vi "WVDIAL+HSRL_v5.3.vi"() -> ()   [LabVIEW 2012]
uses:
  C:/Users/H2ODial/Desktop/Shared Telescope WV DIAL Code/Libraries and VIs/PowerMeterCommands.dll
  Shared Telescope WV DIAL Code/Libraries and VIs/PowerMeterCommands.dll
  <vilib>/DAQmx/write.llb/DAQmx Write (Digital 1D Bool NChan 1Samp 1Line).vi
  <vilib>/DAQmx/miscellaneous.llb/DAQmx Fill In Error Info.vi
  <vilib>/Analysis/baseanly.llb/Mean (DBL).vi
  NCAR_DIAL_Labview/AMCS_Data.vi
  Shared Telescope WV DIAL Code/Libraries and VIs/Scalar_Data.vi
  <vilib>/Analysis/NI_AALBase.lvlib
  Shared Telescope WV DIAL Code/Libraries and VIs/Scalar_Data_2.vi
  Shared Telescope WV DIAL Code/Libraries and VIs/Scalar_Data_4.vi
  Shared Telescope WV DIAL Code/Libraries and VIs/Scalar_Data_3.vi
  Shared Telescope WV DIAL Code/bristol/CLDevIFace.dll
panel:
  out "sigma_off_total":dbl[](array[numeric])=[4.7361664206831265e-25, 4.704555265189846e-25, 4.67312277669019e-25, 4.641868603215992e-25, 4.610792386086212e-25, 4.5798937599868365e-25, 4.549172353018389e-25, 4.51862778677416e-25, 4.488259676402069e-25, 4.458067630633013e-25, 4.428051251896184e-25, 4.398210136337557e-25, 4.368543873901429e-25, 4.339052048374652e-25, 4.309734237462183e-25, 4.280590012841455e-25, 4.251618940197595e-25, 4.2228205793205105e-25, 4.194194484107976e-25, 4.165740202676913e-25, 4.137457277365156e-25, 4.109345244819803e-25, 4.0814036360397235e-25, 4.0536319764083216e-25, 4.026029785750973e-25, 3.99859657840818e-25, 3.9713318632399474e-25, 3.944235143701286e-25, 3.917305917875353e-25, 3.8905436785136965e-25, 3.8639479130808273e-25, 3.8375181038031018e-25, 3.8112537276873907e-25, 3.785154256573241e-25, 3.759219157169389e-25, 3.7334478910754945e-25, 3.7078399148261516e-25, 3.6823946799305074e-25, 3.6571116328753168e-25, 3.631990215175425e-25, 3.6070298633991576e-25, 3.5822300091890585e-25, 3.5575900792854463e-25, 3.5331094955517765e-25, 3.5087876749908485e-25, 3.4846240297677933e-25, 3.4606179672362523e-25, 3.436768889934375e-25, 3.413076195617018e-25, 3.3895392772615455e-25, 3.3661575230847493e-25, 3.342930316532612e-25, 3.319857036317709e-25, 3.296937056408611e-25, 3.2741697460261917e-25, 3.251554469671832e-25, 3.2290905870931807e-25, 3.2067774533121854e-25, 3.1846144186158143e-25, 3.162600828540832e-25, 3.140736023869109e-25, 3.119019340630677e-25, 3.097450110083946e-25, 3.0760276586997706e-25, 3.0547513081546247e-25, 3.0336203753156617e-25, 3.0126341721968216e-25, 2.991792005980208e-25, 2.971093178956684e-25, 2.9505369885181706e-25, 2.930122727127669e-25, 2.9098496822848683e-25, 2.889717136509742e-25, 2.8697243672739283e-25, 2.8498706470054586e-25, 2.830155243027821e-25, 2.8105774175268934e-25, 2.7911364274987386e-25, 2.7718315247081357e-25, 2.752661955653541e-25, 2.7336269615027698e-25, 2.7147257780457946e-25, 2.6959576356446162e-25, 2.6773217591650263e-25, 2.6588173679341805e-25, 2.6404436756788697e-25, 2.622199890449384e-25, 2.604085214561746e-25, 2.586098844541831e-25, 2.568239971051803e-25, 2.550507778817499e-25, 2.5329014465553983e-25, 2.5154201469120286e-25, 2.4980630463842063e-25, 2.480829305237817e-25, 2.4637180774559744e-25, 2.446728510637542e-25, 2.4298597459368107e-25, 2.413110917982359e-25, 2.3964811547911274e-25, 2.379969577731832e-25, 2.3635753013998594e-25, 2.347297433572206e-25, 2.3311350751401097e-25, 2.31508732002067e-25, 2.2991532551047967e-25, 2.2833319601734517e-25, 2.2676225078671837e-25, 2.252023963583222e-25, 2.236535385474671e-25, 2.221155824352112e-25, 2.2058843236723785e-25, 2.190719919472833e-25, 2.1756616403747133e-25, 2.160708507518757e-25, 2.1458595345686165e-25, 2.1311137277120556e-25, 2.1164700856449227e-25, 2.1019275995907964e-25, 2.087485253289068e-25, 2.073142023094825e-25, 2.0588968779652238e-25, 2.0447487795305943e-25, 2.0306966821944526e-25, 2.016739533161752e-25, 2.0028762726015144e-25, 1.9891058337447025e-25, 1.975427143010045e-25, 1.9618391201384895e-25, 1.948340678436903e-25, 1.9349307248979029e-25, 1.9216081604537808e-25, 1.9083718801827206e-25, 1.895220773627962e-25, 1.8821537249925881e-25, 1.869169613534671e-25, 1.8562673138214617e-25, 1.8434456961361037e-25, 1.8307036268484988e-25, 1.8180399688349342e-25, 1.8054535818752412e-25, 1.7929433231795034e-25, 1.7805080478581835e-25, 1.7681466094122697e-25, 1.755857860345701e-25, 1.7436406526975642e-25, 1.7314938387295936e-25, 1.7194162714756045e-25, 1.7074068054790102e-25, 1.695464297486202e-25, 1.683587607177604e-25, 1.6717755978952424e-25, 1.6600271375100748e-25, 1.6483410991903818e-25, 1.6367163622623877e-25, 1.6251518130749766e-25, 1.6136463459136442e-25, 1.6021988639543779e-25, 1.5908082801260055e-25, 1.5794735181698975e-25, 1.5681935136280992e-25, 1.5569672147704635e-25, 1.5457935837366772e-25, 1.534671597460114e-25, 1.5236002488417742e-25, 1.5125785477293987e-25, 1.5016055220247154e-25, 1.4906802187584044e-25, 1.479801705155579e-25, 1.468969069798589e-25, 1.4581814235650682e-25, 1.4474379007909321e-25, 1.436737660408928e-25, 1.4260798867874899e-25, 1.4154637909757664e-25, 1.4048886116065242e-25, 1.3943536158832026e-25, 1.3838581006765858e-25, 1.3734013932288368e-25, 1.3629828522951373e-25, 1.3526018689008124e-25, 1.342257867119734e-25, 1.3319503049616873e-25, 1.3216786750244633e-25, 1.31144250521248e-25, 1.301241359412424e-25, 1.291074837942134e-25, 1.280942578189995e-25, 1.2708442550183176e-25, 1.2607795810937358e-25, 1.2507483073612695e-25, 1.240750223055036e-25, 1.2307851560870465e-25, 1.2208529730375792e-25, 1.210953579206839e-25, 1.2010869185647356e-25, 1.191252973591614e-25, 1.181451765122348e-25, 1.1716833520039885e-25, 1.1619478307265666e-25, 1.1522453350562395e-25, 1.1425760353747595e-25, 1.1329401381799674e-25, 1.1233378853998675e-25, 1.113769553537836e-25, 1.1042354529141042e-25, 1.0947359268328863e-25, 1.0852713503919777e-25, 1.0758421297055504e-25, 1.0664487005835578e-25, 1.0570915274849075e-25, 1.047771102223147e-25, 1.03848794275529e-25, 1.0292425918306789e-25, 1.0200356155490214e-25, 1.010867602053661e-25, 1.0017391599688187e-25, 9.926509169958122e-26, 9.836035183502962e-26, 9.745976252120823e-26, 9.65633913229687e-26, 9.567130708754601e-26, 9.478357978493009e-26, 9.390028035717989e-26, 9.302148055431555e-26, 9.214725277448196e-26, 9.127766990988825e-26, 9.041280518865252e-26, 8.955273202137755e-26, 8.869752384860457e-26, 8.784725399226806e-26, 8.700199550942864e-26, 8.616182105040356e-26, 8.532680271869519e-26, 8.449701193777957e-26, 8.367251931994412e-26, 8.285339454310501e-26, 8.203970622936562e-26, 8.123152183149593e-26, 8.042890752341435e-26, 7.963192809815122e-26, 7.884064686929539e-26, 7.805512558301465e-26, 7.727542432949971e-26, 7.650160146934502e-26, 7.57337135604093e-26, 7.497181529080177e-26, 7.421595942284274e-26, 7.346619674445024e-26, 7.272257601587051e-26, 7.198514394124386e-26, 7.125394512886316e-26, 7.052902207211764e-26, 6.981041512330182e-26, 6.909816249334807e-26, 6.839230023128457e-26, 6.769286223445015e-26, 6.699988025335878e-26, 6.631338390073311e-26, 6.563340066584491e-26, 6.49599559494312e-26, 6.42930730805647e-26, 6.363277335648878e-26, 6.297907608168418e-26, 6.233199860791015e-26, 6.169155638647973e-26, 6.105776301230497e-26, 6.043063030280447e-26, 5.981016833347322e-26, 5.919638551567296e-26, 5.858928867629214e-26, 5.798888310028938e-26, 5.739517264230729e-26, 5.680815977446289e-26, 5.622784570821595e-26, 5.565423042824561e-26, 5.508731282073838e-26, 5.452709076027738e-26, 5.397356119112836e-26, 5.342672021546054e-26, 5.288656322652946e-26, 5.235308497562398e-26, 5.182627968877097e-26, 5.1306141180432717e-26, 5.079266295448115e-26, 5.0285838305725196e-26, 4.9785660439920176e-26, 4.9292122597178655e-26, 4.880521816085966e-26, 4.832494077663027e-26, 4.785128445476612e-26, 4.738424375125138e-26, 4.6923813828266026e-26, 4.6469990631962226e-26, 4.602277098489981e-26, 4.558215278470542e-26, 4.5148135069875e-26, 4.472071819308421e-26, 4.4299904003223627e-26, 4.3885695940220764e-26, 4.34780992252792e-26, 4.3077121010301005e-26, 4.2682770570367184e-26, 4.229505941304242e-26, 4.191400156132326e-26, 4.153961360924621e-26, 4.1171915050160506e-26, 4.081092840060667e-26, 4.045667941127819e-26, 4.0109197318421695e-26, 3.976851511059284e-26, 3.94346696850793e-26, 3.910770219989253e-26, 3.878765828740234e-26, 3.847458837721502e-26, 3.8168548023517886e-26, 3.786959816579413e-26, 3.7577805545800425e-26, 3.729324308299501e-26, 3.7015990199603826e-26, 3.674613333708746e-26, 3.648376631776354e-26, 3.622899094820171e-26, 3.598191740617036e-26, 3.574266496427956e-26, 3.5511362455100554e-26, 3.528814896198588e-26, 3.507317461176492e-26, 3.486660118207953e-26, 3.466860307888483e-26, 3.4479368137858184e-26, 3.4299098560632234e-26, 3.412801205464934e-26, 3.3966342919810845e-26, 3.3814343251481105e-26, 3.367228427279176e-26, 3.354045786622697e-26, 3.3419178044404247e-26, 3.3308782806715067e-26, 3.3209635809193336e-26, 3.312212860029802e-26, 3.3046682753827244e-26, 3.2983752185562495e-26, 3.29338260025694e-26, 3.2897431142923784e-26, 3.287513568833748e-26, 3.2867552048982673e-26, 3.2875340853067966e-26, 3.289921476512414e-26, 3.2939942920704573e-26, 3.299835560859249e-26, 3.3075349233297295e-26, 3.31718918068937e-26, 3.3289028648791126e-26, 3.342788865753138e-26, 3.358969065149828e-26, 3.377575025168756e-26, 3.398748657265788e-26, 3.422642954607728e-26, 3.449422652081664e-26, 3.4792648667855453e-26, 3.512359674236963e-26, 3.5489105220039706e-26, 3.5891344431644435e-26, 3.633261965097536e-26, 3.6815365592521375e-26, 3.734213474993317e-26, 3.791557697858917e-26, 3.8538406892390413e-26, 3.9213356153192504e-26, 3.9943102879548856e-26, 4.073017384110245e-26, 4.1576808542827767e-26, 4.248477496232471e-26, 4.345512364768352e-26, 4.448786294634738e-26, 4.5581537709586704e-26, 4.6732692284515773e-26, 4.793519837808654e-26, 4.9179435948328834e-26, 5.0451328371338053e-26, 5.1731255142748e-26, 5.299290837924887e-26, 5.420222023626943e-26, 5.53165663953385e-26, 5.628454891291683e-26, 5.704674823501702e-26, 5.753787062260405e-26, 5.769064643115553e-26, 5.74415889460443e-26, 5.673827133946316e-26, 5.554718344465795e-26, 5.386066929337925e-26, 5.170120323121083e-26, 4.912158035835312e-26, 4.6200514475002547e-26, 4.3034358779098605e-26, 3.9726716277435353e-26, 3.6378128374023453e-26, 3.307772708312355e-26, 2.989791844851222e-26, 2.6892241436515096e-26, 2.409585649271807e-26, 2.1527785770835842e-26, 1.919402511159775e-26, 1.709083279709411e-26, 1.5207745119483158e-26, 1.3530095944864033e-26, 1.2040974338307356e-26, 1.0722654911053451e-26, 9.55758170763187e-27, 8.529000269297322e-27, 7.621326815896537e-27, 6.820331294600264e-27, 6.113193384990869e-27, 5.4884768053552995e-27, 4.936054405988233e-27, 4.447006306596712e-27, 4.01350649482812e-27, 3.6287074114691265e-27, 3.286628665045252e-27, 2.982053133857502e-27, 2.710432190494805e-27, 2.467800620632622e-27, 2.2507010863407657e-27, 2.0561176436578528e-27, 1.8814175678696082e-27, 1.724300676600419e-27, 1.5827553313450851e-27, 1.4550203259299805e-27, 1.3395518832270707e-27, 1.234995172388499e-27, 1.1401596616151055e-27, 1.0539978395563054e-27, 9.755868171920564e-28, 9.041124308282113e-28, 8.388554686323786e-28, 7.791797569678583e-28, 7.245218245948973e-28, 6.743819381596948e-28, 6.283163098755046e-28, 5.8593032346752675e-28, 5.468726321210164e-28, 5.108300131750884e-28, 4.775228773786931e-28, 4.467013412002027e-28, 4.181417907319234e-28, 3.916438696977483e-28, 3.670278362224614e-28, 3.4413224156682114e-28, 3.2281188706205514e-28, 3.029360261582784e-28, 2.8438677764436214e-28, 2.6705772634396255e-28, 2.5085268535677297e-28, 2.356846015299008e-28, 2.2147458604462534e-28, 2.081510545634908e-28, 1.9564896453728212e-28, 1.8390913738842352e-28, 1.7287765586913761e-28, 1.6250532759661657e-28, 1.5274720714661247e-28, 1.435621701168333e-28, 1.3491253280333026e-28, 1.2676371266924668e-28, 1.1908392491273447e-28, 1.1184391104493528e-28, 1.0501669588488019e-28, 9.857737007616221e-29, 9.250289505277767e-29, 8.677192817164208e-29, 8.136466585155294e-29, 7.626270269664177e-29, 7.144890498931933e-29, 6.690729697909333e-29, 6.262295865445962e-29, 5.858193379226559e-29, 5.477114719070298e-29, 5.117833016685385e-29, 4.779195345355935e-29, 4.460116672941723e-29, 4.159574412717862e-29, 3.8766035085313356e-29, 3.610292001520259e-29, 3.359777029252782e-29, 3.1242412137098097e-29, 2.902909398873338e-29, 2.695045702172569e-29, 2.499950848733905e-29, 2.3169597597114745e-29, 2.1454393688082381e-29, 1.984786644280984e-29, 1.8344267951922419e-29, 1.6938116433705343e-29, 1.5624181441700836e-29, 1.439747040443755e-29, 1.3253216363128416e-29, 1.2186866778564523e-29, 1.1194073298259488e-29, 1.027068237868702e-29, 9.41272667323786e-30, 8.616417100740263e-30, 7.878135520832268e-30, 7.194427947435567e-30, 6.561998239457055e-30, 5.9777022134514484e-30, 5.438542128318805e-30, 4.941661497222303e-30, 4.4843401864961795e-30, 4.0639897652743174e-30, 3.678149073494049e-30, 3.32447997937297e-30, 3.000763300568808e-30, 2.7048948662138683e-30, 2.4348816997231054e-30, 2.1888383046853783e-30, 1.9649830384363482e-30, 1.7616345601080574e-30, 1.5772083417641433e-30, 1.41021323314241e-30, 1.2592480721156737e-30, 1.1229983345711438e-30, 1.0002328188090904e-30, 8.898003608818597e-31, 7.906265785078758e-31, 7.017106423265677e-31, 6.221220742613051e-31, 5.509975737248236e-31, 4.875378732287941e-31, 4.3100462574946304e-31, 3.8071732687790596e-31, 3.3605027540420555e-31, 2.964295765136466e-31, 2.6133019224912582e-31, 2.302730443047367e-31, 2.028221746319981e-31, 1.785819698883956e-31, 1.571944569933226e-31, 1.383366812786611e-31, 1.217181992487339e-31, 1.0707887255920024e-31, 9.41901183885076e-32, 8.286711261751362e-32, 7.282214916074516e-32, 6.400758489832818e-32, 5.623904147671109e-32, 4.938867921697972e-32, 4.334463318815432e-32, 3.80089121769985e-32, 3.329583042957907e-32, 2.9130592710425146e-32, 2.544799971983946e-32, 2.219126721730452e-32, 1.9310955232755848e-32]
  out "sigma_on_total":dbl[](array[numeric])=[1.4787315438349907e-23, 1.471501798802285e-23, 1.464231394662418e-23, 1.4569216526022592e-23, 1.4495738897409737e-23, 1.4421894186265373e-23, 1.434769546715974e-23, 1.4273155759788748e-23, 1.4198288023456042e-23, 1.4123105152791947e-23, 1.4047619973042604e-23, 1.3971845236586865e-23, 1.3895793617371425e-23, 1.381947770795712e-23, 1.3742910015857432e-23, 1.3666102958094782e-23, 1.3589068859169402e-23, 1.3511819946965545e-23, 1.343436834852627e-23, 1.3356726088660775e-23, 1.3278905084359422e-23, 1.3200917143654812e-23, 1.3122773962181173e-23, 1.3044487120136741e-23, 1.2966068079379167e-23, 1.2887528181705935e-23, 1.280887864645543e-23, 1.2730130566668176e-23, 1.2651294909304667e-23, 1.2572382511131376e-23, 1.2493404078126522e-23, 1.2414370183434812e-23, 1.2335291264934119e-23, 1.2256177624718979e-23, 1.217703942715269e-23, 1.2097886697548654e-23, 1.2018729320712635e-23, 1.1939577040847508e-23, 1.1860439459053391e-23, 1.178132603369378e-23, 1.1702246078860594e-23, 1.1623208764429943e-23, 1.1544223114245504e-23, 1.1465298007100527e-23, 1.1386442174876053e-23, 1.1307664203452922e-23, 1.1228972532006195e-23, 1.1150375452637873e-23, 1.1071881110338761e-23, 1.0993497503734642e-23, 1.0915232484490551e-23, 1.0837093757279006e-23, 1.075908888098364e-23, 1.0681225268339973e-23, 1.0603510186352726e-23, 1.0525950757460925e-23, 1.0448553958493267e-23, 1.037132662354594e-23, 1.0294275442393744e-23, 1.0217406963238484e-23, 1.0140727591488213e-23, 1.0064243592154774e-23, 9.987961090294116e-24, 9.911886071512357e-24, 9.836024383391568e-24, 9.760381736518965e-24, 9.684963704924737e-24, 9.60977572847412e-24, 9.534823112538791e-24, 9.460111030247358e-24, 9.385644523289062e-24, 9.311428503379682e-24, 9.237467752939021e-24, 9.1637669272307e-24, 9.09033055529708e-24, 9.017163041332023e-24, 8.944268665880828e-24, 8.871651587851976e-24, 8.799315845358803e-24, 8.727265357183314e-24, 8.65550392483017e-24, 8.584035233431315e-24, 8.512862853443734e-24, 8.441990241976577e-24, 8.371420744879967e-24, 8.30115759752875e-24, 8.231203926927024e-24, 8.161562752887824e-24, 8.092236989774732e-24, 8.023229448060604e-24, 7.954542835889658e-24, 7.886179760290278e-24, 7.818142729624757e-24, 7.750434154096213e-24, 7.683056347675882e-24, 7.616011530181347e-24, 7.549301828314853e-24, 7.482929277057427e-24, 7.416895821895255e-24, 7.351203319362845e-24, 7.285853539749422e-24, 7.220848167799621e-24, 7.156188804409643e-24, 7.091876968465427e-24, 7.02791409755192e-24, 6.964301550724863e-24, 6.901040608572782e-24, 6.838132475952623e-24, 6.775578282364756e-24, 6.713379084183873e-24, 6.651535865939141e-24, 6.590049541293287e-24, 6.5289209550606835e-24, 6.46815088430602e-24, 6.40774003944497e-24, 6.347689066346921e-24, 6.2879985469666566e-24, 6.228669001264069e-24, 6.169700887964062e-24, 6.111094606297088e-24, 6.0528504971542e-24, 5.994968844369398e-24, 5.937449875851488e-24, 5.880293765105849e-24, 5.82350063219817e-24, 5.767070545238083e-24, 5.7110035214439225e-24, 5.655299527942129e-24, 5.5999584837121235e-24, 5.544980260090087e-24, 5.490364682162052e-24, 5.436111530002443e-24, 5.3822205392790905e-24, 5.328691403076694e-24, 5.275523772106918e-24, 5.2227172566077816e-24, 5.170271426653518e-24, 5.118185813533807e-24, 5.066459910980123e-24, 5.015093175565678e-24, 4.964085027910957e-24, 4.9134348538588365e-24, 4.863142005178444e-24, 4.813205800593375e-24, 4.7636255264628436e-24, 4.714400437887786e-24, 4.665529759575633e-24, 4.617012686584397e-24, 4.568848385057435e-24, 4.521035993359352e-24, 4.473574622567741e-24, 4.4264633574709985e-24, 4.379701257140268e-24, 4.333287356089523e-24, 4.2872206644216265e-24, 4.241500168960551e-24, 4.196124833867207e-24, 4.151093601530227e-24, 4.106405392776687e-24, 4.06205910811475e-24, 4.01805362783006e-24, 3.9743878130977926e-24, 3.931060506426416e-24, 3.888070532187342e-24, 3.845416697225424e-24, 3.803097791801521e-24, 3.761112589558677e-24, 3.719459848784516e-24, 3.6781383122768084e-24, 3.6371467083176915e-24, 3.596483751198191e-24, 3.556148141569368e-24, 3.5161385668725815e-24, 3.476453702237941e-24, 3.437092210484289e-24, 3.398052742913235e-24, 3.359333939535743e-24, 3.3209344298325475e-24, 3.282852832810783e-24, 3.2450877578143793e-24, 3.20763780456859e-24, 3.1705015639611164e-24, 3.1336776181464896e-24, 3.097164541012893e-24, 3.0609608986345336e-24, 3.0250652497092765e-24, 2.9894761456426302e-24, 2.9541921311120647e-24, 2.9192117444089036e-24, 2.8845335177057522e-24, 2.8501559773849925e-24, 2.8160776443587784e-24, 2.7822970344442195e-24, 2.7488126586004656e-24, 2.7156230232245448e-24, 2.6827266305003526e-24, 2.6501219784943642e-24, 2.6178075617335478e-24, 2.5857818711071018e-24, 2.554043394426032e-24, 2.5225906166099657e-24, 2.4914220197581437e-24, 2.460536083562059e-24, 2.4299312854227364e-24, 2.3996061007879786e-24, 2.3695590033135076e-24, 2.3397884650752963e-24, 2.3102929567234233e-24, 2.2810709477376482e-24, 2.2521209066220334e-24, 2.223441301144551e-24, 2.195030598367685e-24, 2.1668872649808488e-24, 2.139009767421492e-24, 2.1113965718990352e-24, 2.0840461448985418e-24, 2.0569569529523272e-24, 2.0301274631283374e-24, 2.0035561428054193e-24, 1.9772414602815678e-24, 1.9511818844995554e-24, 1.9253758853690898e-24, 1.899821933940881e-24, 1.8745185024029975e-24, 1.849464064377468e-24, 1.824657094743691e-24, 1.8000960701355398e-24, 1.775779468759368e-24, 1.7517057706694626e-24, 1.727873457712613e-24, 1.7042810137920967e-24, 1.680926924924265e-24, 1.6578096792577794e-24, 1.6349277672442792e-24, 1.6122796816898694e-24, 1.5898639178429036e-24, 1.5676789735498486e-24, 1.545723349156838e-24, 1.523995547803786e-24, 1.5024940753570163e-24, 1.4812174405527824e-24, 1.4601641549998617e-24, 1.439332733283451e-24, 1.418721693095806e-24, 1.3983295551688655e-24, 1.3781548434656219e-24, 1.3581960850812125e-24, 1.3384518105195583e-24, 1.31892055350055e-24, 1.2996008512285673e-24, 1.280491244321182e-24, 1.2615902768608962e-24, 1.2428964965013605e-24, 1.2244084544556605e-24, 1.2061247055972778e-24, 1.18804380847374e-24, 1.170164325267996e-24, 1.1524848220267015e-24, 1.1350038684587006e-24, 1.1177200382345184e-24, 1.1006319087873e-24, 1.0837380614524356e-24, 1.0670370815482544e-24, 1.0505275583081984e-24, 1.0342080849145352e-24, 1.0180772586459747e-24, 1.002133680786328e-24, 9.86375956699353e-25, 9.708026958102332e-25, 9.554125116984566e-25, 9.402040220982259e-25, 9.251758488791391e-25, 9.10326618133062e-25, 8.956549601324274e-25, 8.811595093934017e-25, 8.668389047146285e-25, 8.526917891169106e-25, 8.387168099226145e-25, 8.249126187726412e-25, 8.11277871624403e-25, 7.978112287690921e-25, 7.845113548837181e-25, 7.7137691895700685e-25, 7.584065944292599e-25, 7.455990591003361e-25, 7.329529951800705e-25, 7.204670893184894e-25, 7.0814003260182975e-25, 6.959705205656102e-25, 6.839572532380776e-25, 6.720989350586905e-25, 6.603942749997578e-25, 6.488419865446174e-25, 6.374407876399595e-25, 6.261894007954661e-25, 6.150865530211098e-25, 6.041309758809611e-25, 5.933214054752622e-25, 5.826565824909757e-25, 5.7213525213155325e-25, 5.617561642453114e-25, 5.515180732168093e-25, 5.41419738053984e-25, 5.314599223588945e-25, 5.2163739433775345e-25, 5.119509268339076e-25, 5.023992973354091e-25, 4.929812879269966e-25, 4.83695685390146e-25, 4.745412811324431e-25, 4.655168712306681e-25, 4.566212564494616e-25, 4.478532422285788e-25, 4.392116386922725e-25, 4.3069526067810185e-25, 4.223029277063312e-25, 4.1403346405654575e-25, 4.058856986900904e-25, 3.978584653260092e-25, 3.8995060243022608e-25, 3.821609531984159e-25, 3.7448836561800954e-25, 3.6693169242484616e-25, 3.594897911308621e-25, 3.5216152405774533e-25, 3.4494575830558584e-25, 3.3784136580262306e-25, 3.308472232608705e-25, 3.239622122625241e-25, 3.1718521918713437e-25, 3.1051513529593895e-25, 3.0395085668400436e-25, 2.974912843267899e-25, 2.9113532407655295e-25, 2.8488188666707203e-25, 2.7872988773817864e-25, 2.7267824785261776e-25, 2.667258924823239e-25, 2.6087175203327154e-25, 2.5511476187464887e-25, 2.49453862309765e-25, 2.4388799863481035e-25, 2.3841612111128817e-25, 2.3303718501202106e-25, 2.277501506014524e-25, 2.2255398318054605e-25, 2.1744765307872185e-25, 2.1243013566313854e-25, 2.0750041137677605e-25, 2.0265746572786782e-25, 1.979002893228296e-25, 1.9322787785775259e-25, 1.886392321556429e-25, 1.8413335817176915e-25, 1.7970926700451188e-25, 1.7536597491883382e-25, 1.711025033495423e-25, 1.6691787893275044e-25, 1.6281113350234714e-25, 1.5878130413225444e-25, 1.5482743312291127e-25, 1.509485680363358e-25, 1.471437617088968e-25, 1.4341207226803577e-25, 1.3975256314606232e-25, 1.3616430310380968e-25, 1.3264636623565183e-25, 1.2919783200560773e-25, 1.2581778524977242e-25, 1.2250531619775e-25, 1.1925952049379949e-25, 1.1607949921510753e-25, 1.1296435889026462e-25, 1.0991321151545042e-25, 1.0692517457601112e-25, 1.0399937106080184e-25, 1.011349294910818e-25, 9.83309839259911e-26, 9.558667400044944e-26, 9.290114492484407e-26, 9.027354752457115e-26, 8.770303823915941e-26, 8.518877916321012e-26, 8.27299380543734e-26, 8.03256883542986e-26, 7.797520921491743e-26, 7.567768551541595e-26, 7.343230788324e-26, 7.123827271679794e-26, 6.909478220177844e-26, 6.700104434191661e-26, 6.495627296924976e-26, 6.295968777330477e-26, 6.101051431943822e-26, 5.910798406908099e-26, 5.725133440543019e-26, 5.543980865221508e-26, 5.367265609180593e-26, 5.194913199682845e-26, 5.0268497641937015e-26, 4.8630020330495616e-26, 4.703297341402659e-26, 4.547663631716583e-26, 4.396029455705198e-26, 4.2483239762150683e-26, 4.104476969986872e-26, 3.9644188294962993e-26, 3.8280805650176317e-26, 3.6953938068621367e-26, 3.5662908074279575e-26, 3.4407044436409546e-26, 3.318568218574498e-26, 3.1998162639406745e-26, 3.0843833417969425e-26, 2.972204847042788e-26, 2.863216809168607e-26, 2.7573558942900653e-26, 2.654559407219964e-26, 2.554765293444751e-26, 2.457912141186444e-26, 2.363939182937315e-26, 2.2727862979161852e-26, 2.1843940134449242e-26, 2.0987035070561285e-26, 2.0156566082825927e-26, 1.9351958002386438e-26, 1.8572642216201332e-26, 1.781805668084179e-26, 1.7087645941906986e-26, 1.6380861147912063e-26, 1.5697160066987254e-26, 1.5036007100119938e-26, 1.4396873298802572e-26, 1.3779236375531374e-26, 1.3182580719565103e-26, 1.2606397408702273e-26, 1.2050184221481847e-26, 1.1513445649242606e-26, 1.0995692906135215e-26, 1.0496443940040375e-26, 1.0015223440988908e-26, 9.551562851196472e-27, 9.10500037130056e-27, 8.675080968505971e-27, 8.261356382660395e-27, 7.863385130749629e-27, 7.48073251201452e-27, 7.112970610797966e-27, 6.759678299302436e-27, 6.420441238803092e-27, 6.094851880388082e-27, 5.7825094633272326e-27, 5.4830200137799664e-27, 5.195996341708768e-27, 4.921058036596805e-27, 4.6578314617210455e-27, 4.405949747513591e-27, 4.165052783663769e-27, 3.934787209455887e-27, 3.714806402699178e-27, 3.504770468163001e-27, 3.304346223221544e-27, 3.1132071826646397e-27, 2.9310335423411182e-27, 2.7575121603379643e-27, 2.5923365371878643e-27, 2.435206794071242e-27, 2.2858296495546067e-27, 2.143918394444303e-27, 2.0091928647685935e-27, 1.8813794130513052e-27, 1.7602108778360022e-27, 1.6454265510772036e-27, 1.5367721436594311e-27, 1.4339997490158732e-27, 1.336867804720128e-27, 1.2451410519362652e-27, 1.1585904929406186e-27, 1.0769933462831097e-27, 1.000133000176548e-27, 9.277989633650412e-28, 8.597868139363997e-28, 7.958981459067521e-28, 7.359405136173592e-28, 6.797273736804779e-28, 6.2707802483043625e-28, 5.778175453184356e-28, 5.317767281066632e-28, 4.88792013621742e-28, 4.487054202631287e-28, 4.1136447250920456e-28, 3.7662212671886986e-28, 3.443366945925029e-28, 3.1437176427613727e-28, 2.865961192022443e-28, 2.6088365460259276e-28, 2.371132917499321e-28, 2.151688899969665e-28, 1.949391565444193e-28, 1.7631755410820872e-28, 1.5920220644483194e-28, 1.434958017745442e-28, 1.2910549427114306e-28, 1.1594280355518867e-28, 1.0392351235578676e-28, 9.296756237302285e-29, 8.299894847295184e-29, 7.394561126257081e-29, 6.573932819721393e-29, 5.831560330926628e-29, 5.161355567587526e-29, 4.557580677838355e-29, 4.014836686968421e-29, 3.528052051321694e-29, 3.0924711433038544e-29, 2.7036426854519976e-29, 2.3574081494715414e-29, 2.0498901383377131e-29, 1.777480770825479e-29, 1.5368300866534752e-29, 1.324834492861e-29, 1.1386252715954142e-29, 9.755571703889079e-30, 8.33197096263397e-30, 7.093129354141314e-30, 6.018625201493139e-30, 5.089827655697999e-30, 4.2897899756888136e-30, 3.603144942924524e-30, 3.01600262483193e-30, 2.515850699194995e-30, 2.091457544318933e-30, 1.7327782923547947e-30, 1.4308640334140687e-30, 1.1777743469393509e-30, 9.664933233041098e-31, 7.90849223599496e-31, 6.4543790881185804e-31, 5.255501504793574e-31, 4.2710291498533e-31, 3.46574691447889e-31, 2.809449101215201e-31, 2.2763747343352457e-31, 1.8446839685184108e-31, 1.495975304311734e-31, 1.2148430597163782e-31, 9.88474284013865e-32, 8.062840460655379e-32, 6.595877825497762e-32, 5.413091605652855e-32, 4.457216970219223e-32, 3.682221884745194e-32, 3.051338447860446e-32, 2.5353689151588993e-32, 2.111243128547078e-32]
  out "FileHour":i32=1
  out "L_Count":i32=763
  out "background start":u32=534
  in  "Tab Control 2":enum32{"WV ND ", "Beta aerosol"}(tab)
  out "Absolute Humdity":dbl[][](graph)=[[8.013524111720983, 11.092691238585498, 10.288221424893004, 9.585235543366469, 9.124349496709476, 7.922146661387423, 6.43212978075061, 6.65485118409192, 5.791003774591024, 5.36848606757388, 6.67460656379689, 5.935278628524312, 5.9856556340421845, 5.650166412066087, 5.358776976004566, 5.192654509264062, 4.925979260947111, 4.712563230203951, 4.329866427542913, 4.451826428685255, 4.756195124715099, 5.108044302901964, 4.751411039361093, 4.489181622537253, 3.737884330358757, 3.49073010674943, 3.9561366161724636, 4.719803048978352, 5.569629756780132, 6.285825882940165, 6.401804214100326, 5.955414796937688, 5.51889050588234, 5.209168052079253, 4.701835299576782, 4.630863252048436, 4.7066044948864265, 4.05528208798291, 4.632676987395666, 4.158823928633111, 4.699057947310015, 4.836965507895837, 4.737451804077713, 4.5132002398747835, 4.456157443873025, 4.32678379860644, 4.3093686574942724, 4.45865308519626, 4.340659868127958, 4.35232021408519, 3.643303086400929, 3.449988462089912, 3.3747258695791094, 3.17536369682735, 3.8717997904591805, 3.470162712497249, 3.856064549342613, 3.7088392501494374, 3.044004427358953, 3.3734186815883525, 3.0038156893614354, 3.034632240721526, 2.9674388039874557, 2.968346598385485, 2.558411980209298, 2.9987035305223118, 1.830798603341773, 1.985152828296957, 2.2742059018740557, 1.4997148541296401, 3.317740084405948, 3.1525842391224335, 3.3399613035461027, 3.346726519806233, 3.074849546353178, 2.6633489165508526, 3.2227003756697052, 2.7189183888944277, 2.41709116886834, 2.2878902079654804, 0.5566014311811843, 0.07127573913739212, -0.618419878963139, -0.8272211167165782, -0.9314508411121427, -0.6530566075787011, 0.06364118320104996, 0.7666113681832725, 1.360439270288413, 1.6489443581267853, 1.6010434708855796, 1.3363373133731895, 1.0765794030634948, 0.720959404037179, 0.4191305473317959, 0.26604510638431506, -0.025165402876267902, 0.1366199825101397, 0.6239339797942876, 1.550813303234633, 3.090739385617948, 4.761493001739283, 6.124270063819525, 8.538382013658808, 11.425052881091746, 9.65055967811851, 10.915587541664499, 12.729085631448612, 10.984473617772355, 16.301044099557103, 13.123755357766695, 7.780694671791993, 5.740537802892409, -0.31582738817183914, 2.4404649385545043, 7.114121651645781, 9.538781747442743, 6.354185086513254, 3.622117494877131, -4.0915981242938315, -1.159606171848143, 6.7640444801423385, 8.995504493825495, 10.389398503184573, 4.045683899100252, 0.003592192615548344, -2.629746525367323, -1.3604087110373004, -0.11029507889894587, -0.18400479097918468, -1.5722195068682385, -5.7920251850837925, -6.389239141780525, -3.186567588031156, -2.0584572218598485, -0.8310390063944286, -2.3727320561666434, -3.2820659747537353, -1.5131867727828292, -0.2861325643070063, -0.0791790440308039, 0.559099803054959, 0.2042303831245666, -0.44959487787876057, -0.6534818881145138, -1.13070332806575, -0.8370418712578157, -0.525977817157662, 0.05209489012004466, 0.21432025686680853, 0.5098615468039083, 0.5517740319688078, 0.9740697360200072, 1.8133267419305859, 2.0447091135601654, 2.6699084491034193, 2.4293959646613534, 1.454559510164313, 1.547575490735375, 1.7369946350546264, 1.7818720675739486, 2.4529745546318207, 2.18979954988764, 1.2211051927374852, 1.4668172992201733, 1.1881587522475676, 0.24708618976996918, 1.481991200481501, 0.9054676022560789, 0.6925233611336278, 0.7297268637564226, 0.3907135610725875, 0.15570078197763523, 2.4282440354053705, 2.3354482725531627, 1.1346044286013615, 1.9175385233886442, -0.8437685317346915, -0.3307482719078713, 0.47510562519216437, 2.482557430100584, 4.405029194633034, 3.833307540280627, 3.911032309002459, 2.9840203518239106, 4.844948148576043, 9.189677913322322, 9.970834390200139, 4.333205976962303, 0.8851905554896997, 0.537001112015682, -2.5225878362154392, 3.503757279919347, 0.30788715192909855, -5.174345752409806, -5.076317979097928, -8.837569874173193, -9.61411308904375, -0.44973803955927844, -3.2855259007407707, -3.6549167064717816, 1.78627421633821, -4.2379507677675194, -2.580617864570767, 3.1133701481237215, 4.804398665087993, 1.3565505544629082, 10.129022892732497, -7.576983797172085, 1.7172524032070147, 12.042679500140002, 13.309868432733435, 30.752131210373516, 15.19346881686317, -14.357572381686072, -18.229811798426834, -24.810486525744537, 1.0876196074210494, 81.575504510787, 95.65046720530243, 119.1495369519025, 79.2086587433161, 66.85908282291253, 0.8590524981517791, 46.8622425556482, 34.5172109379284, 71.74596501405112, 224.09160799629288, 68.18635539213379, 50.438357517156795, -93.74543443322608, -65.58963655593323, -73.29681727166235, 248.51527294070166, 74.82208173544622, 122.68245291460212, -115.0623040444003, -193.79112617387963, 459.9200936829966, -194.2378575583177, -131.45821392390621, 77.6834538920087, -122.83393804903073, -273.71825868845315, 332.0052992138547, -511.911198790546, -506.02785083502636, -289.83609721884216, -1714.3795471816625, 12.419730981910083, -121.88490739997839, -379.6105035874339, 249.26740392220114, -326.63750577538104, -1836.7213589755293, -264.6384923955867, 1107.2799647203044, -111.76502064831344, 140.9229405639405, -372.967152298866, 310.40468567480906, -63.87814127749086, 546.4791343076924, -340.0025136352076, 972.3405061781073, -1157.6851530907131, -1541.28588671552, 396.86656347236936, 464.11054720621064, -410.6631243237224, -1120.4941883092201, -1356.6857890508506, -1006.2172125895717, -57.18235363041792, 452.55419588813646, 1696.8518100513775, 1976.644154767608, 2353.269047473912, 103.88997581645728, 247.14372078823683, -172.49513834273407, 1392.436547815471, 1053.8594059556765, 1879.87861980049, -36.5562780975342, -383.003140650159, -1206.8935063926363, -2357.287854726186, 691.4265506115088, -1879.9385609164433, -2717.708257587145, -2878.005455653812, -2846.019105764703, -2030.0266501758895, -1035.6136862460694, -2926.2523124745385, -254.5677562186089, -196.26687287046437, 440.565270098482, 3353.107367441271, 6754.482681664373, 3894.379407442549, 5818.779031116694, 275.0551211608562, 143.4015325424874, 2333.5761741191163, -298.5788857156622, -59.01882814774661, -1158.077256921881, -912.278255502008, -3695.402824407278, -1233.1715667640563, -4954.319620969596, -205.3481255900909, -67.05749967044153, -138.6451609663425, -1934.8736921200682, -140.73223454929482, 227.36196532639724, 602.1489982454652, 834.8047002035399, -4706.917824621832, -889.2629422848714, -5346.760504196195, -2299.918580325633, -747.6640688460263, -477.40401824691816, -1347.8762430719107, -1286.5934396877838, -1006.0214110632136, 978.1761008903106, 4112.3789369771075, -815.5132035622793, 4381.420720327582, 3348.322798021013, 813.1489005635628, 2671.6819443453132, 983.1399000987108, 2023.777142257615, -2048.8629469441007, -2595.3357864836134, -1769.7055217793031, 3681.0238547835256, 5227.864122609879, 889.4024431118, 4049.897234507725, -449.0121696580251, -2486.9589737756805, -1664.6810407588496, 7039.234373622698, 3729.4110873975173, 4675.856598322998, -3176.130930424592, -26637.319616657882, 195.86644013782384, -197.81632575970642, 9990.75731964173, 7314.828324103919, -8778.07689285618, -6109.368401060864, -7559.186529976081, -5886.883404034405, -1045.9731526529101, 27970.323731761884, 4414.23233858691, -2701.3411763173244, -8494.839503751893, -6203.114044026042, 7694.171891508432, 9167.053482593556, 537.4286812940435, 4740.313935450109, 10502.908241370114, -1747.6388500440808, 2782.747913621642, 4079.8758863085004, -9651.2321523187, -3448.1241819121947, -19160.742472812428, -11803.164416636693, 9107.402402118081, -2857.6358814290475, -16301.11892363841, 915.4758133647605, -6199.685334636605, 86904.97937190029, -1673.2110274870029, -27173.718172329987, -175875.6375753611, -51426.386711433624, -39937.77183785317, -43255.44826186634, -54879.307327893686, -55184.85363606102, -39460.14591645426, -125656.60884272974, -16525.613992068582, -5436.813862077934, 160296.49432357878, 25357.465678612807, 9965.587697227144, 22851.587040093276, 43587.91416570906, 1757.2623095771235, -4553.556563885617, 39398.74364737146, -13878.046320554735, -22867.14444003368, -42131.699611613825, -64831.6648748474, -15867.164219875149, -39025.50516912196, -15821.761497495734, 69671.19364625846, 25141.99521242797, 15672.51590699608, 2662.304996208152, 8738.383479181082, 18058.896278346223, 44691.02277938234, -20243.21737777961, -1397.5594239007644, -12858.426552655406, -177125.639372152, -50000.66690364448, -27249.918371031632, 34123.17040967579, 83244.97120261466, 68959.44189274254, 24061.26591849187, 17443.96926280221, -16536.644546936812, 2869.2848412540507, 79583.04654881793, -29505.109760835767, -14305.428576573662, -23508.365106003766, -70027.76613371944, 28355.291917658065, 83413.81461548817, 60795.12694828051, 117098.32852207759, 258363.99739456666, 207589.24777410782, -23207.117568479105, 257018.6960502074, 33687.00301388019, 139991.7696829697, -85679.00826200172, 114153.0732389654, -42323.29108014541, -97946.2642061314, -297128.8225593948, -633494.2532802554, 30164.819537164905, -285062.21932897554, 20002.330100714807, -113619.98112104517, 89551.21552739848, -217382.38609179927, -285163.4608941957, -197927.68145352538, 130817.18416054407, 518039.0692672737, -366530.34738765116, 502395.0597158051, -116148.54408511781, -137657.22716846893, -153901.29948622966, 753163.4678734696, 577767.6447593329, 403166.29740177, 62501.33017968078, 717262.2383827901, 933824.1875649366, -634718.4086711712, -797302.5686909804, -349979.8438580412, 276254.3387246677, -753562.5789965567, -814.8355216278218, -784675.9408398503, -2027108.8603061775, -952729.1134820146, -804864.4770871834, -217674.35668206058, 1042495.7762176967, -274256.81191459665, -1003080.5390808955, -639594.1299538026, 1308690.97177827, 3821786.3447531303, 3122017.5489116167, 7346802.957570168, -1474805.2200785223, 9152536.79596, 1764761.7674513892, -8033959.797272627, 2128113.1158438805, -930005.2403280559, -7470162.602741275, -17278427.11173834, 1707025.1883956885, 13756139.166704044, 12024030.869362636, 10138183.081979012, 5069983.9182277415, 4286649.837321222, -22466674.014733188, -41528811.09220256, -20932767.14997173, -21295884.90120367, -692749.2987715302, -2778761.2828054084, 13434527.424383366, 2448811.581341309, 7341988.369137925, 54089991.938083746, -74351662.90754429, 103662777.09978938, -4162015.3993728594, -283660131.6044327, -40985094.58470669, -251054358.32237974, 108430641.20922936, -237257897.0270308, -698373761.5964577, 102415874.42354193, 2133000504.2990403, -139045389.20634097, 259300660.71948236, 631848947.7857363, 3307603797.596202, 2304753315.2244596, -1585263684.771963, 1264891768.041471, -382485493.9997457, -3586118671.5480056, 280291910.4616509, -317712325.0631372, 7038783518.743804, 917514824.129406, -14929172335.896292, -41150181801.02589, -54918033378.87475, 17609412153.846558, 113770720031.12256, 5952062153.46267, -19610954237.452915, -16896952728.569017, -24560286332.59649, -18523503867.204674, -5632856335.653218, 21785186731.319187, 0.0, 0.0, 0.0, 0.0, 0.0, 0.0]] caption="Water Vapor Number Density"
  out "CH3 RingBuffer long":dbl[][](array[numeric])
  out "CH3 RingBuffer short":dbl[][](array[numeric])
  in  "?":T1(tab)=enum."NRB combined"
  out "NRB WV Offline":dbl[][](graph)=[[2.136490397874901e-05, 7.775503892965314e-05, 0.0001738194317437546, 0.00031327898325496123, 0.00050905074146314, 0.0007709921923120845, 0.0011210082558800684, 0.001550816723073192, 0.0020922995036787386, 0.002746060414814386, 0.0034899724155252982, 0.004455719513652091, 0.0056747566751014075, 0.007223380288301658, 0.00908075375523663, 0.011265206327745593, 0.013831195790574737, 0.016857418407965303, 0.020424052485010676, 0.0243685673607689, 0.028710655546787027, 0.03349119534582278, 0.03856751063876057, 0.04404526030609718, 0.04958547935456178, 0.05512400687795353, 0.06037107802519336, 0.06544847897156217, 0.07062759095245083, 0.0757767117489249, 0.08129948299742407, 0.0871530456268756, 0.09360230512929102, 0.0996288790263056, 0.1059750258749744, 0.1121245379906857, 0.11715490531088922, 0.12213149908108062, 0.12771722335425853, 0.13307007280019367, 0.13876359912564343, 0.14491708319643634, 0.14928741669348666, 0.15391368150982457, 0.15765722712958113, 0.16077312739567534, 0.16419270999977167, 0.16714287789562318, 0.17007128120826956, 0.17377808411288473, 0.17772199031124758, 0.18089323981276878, 0.18462049445431242, 0.18737581097625, 0.19062936857164584, 0.19320469712387803, 0.19512822789155068, 0.1978649563844547, 0.19740722030595018, 0.20024362409091995, 0.20093417992598095, 0.19951653286337925, 0.20079269657801999, 0.19949070403330754, 0.2002976233169027, 0.20068192827424414, 0.20023155346997104, 0.1988609121300482, 0.19624486334414099, 0.19686275648435436, 0.19760844148317042, 0.19889404932396576, 0.2014091275232545, 0.20082981556674798, 0.20027013916793066, 0.20012784441128417, 0.20013698108096678, 0.20333618328901248, 0.20551133792406634, 0.20644159598677791, 0.20889841489188998, 0.20878103938207954, 0.21364943581221388, 0.22812399963865276, 0.2572034592206941, 0.31167733057671954, 0.39575343812216957, 0.5150167022204695, 0.7142583901170365, 1.2455111425139842, 2.2482754765406043, 3.705918715137743, 5.6162609103702374, 7.614723851719535, 9.787588324178028, 12.363218665485435, 15.78357953525832, 21.051935757233093, 27.37063645113918, 34.129547162604936, 39.33700281217425, 39.55034318328333, 35.36833950254932, 27.755874501690236, 19.245435141872182, 12.931819104076864, 8.933787018458988, 6.985508108543602, 6.055943951018168, 5.146358299495447, 4.177729790219288, 3.06974300078666, 2.0195604870029427, 1.2651059600818206, 0.7202222547753562, 0.3579263437139261, 0.1959056044073879, 0.10567278730784416, 0.04945784916592421, 0.03963686293626402, 0.03712057711628809, 0.030422198242041534, 0.032989132356697023, 0.03798575250157523, 0.041696881156003, 0.04629445112625132, 0.0459127314402871, 0.04647354088151787, 0.04489253092309751, 0.04903448937146409, 0.05526702074555916, 0.06452120608230616, 0.09534720438654214, 0.14407395528088807, 0.22750600998341844, 0.3668341424807134, 0.5534477588148872, 0.7923067704039555, 1.0630710947003668, 1.3203669943271144, 1.5421012359818196, 1.6678349738115243, 1.6574560611004452, 1.5334334103409804, 1.3218361909494654, 1.106324267711738, 0.9556252405841946, 0.8888862098039311, 0.9019348753897559, 0.9807916000433566, 1.096729618579646, 1.2211653737035626, 1.3663922001089581, 1.54338261806784, 1.7652368019100166, 2.0023829796967823, 2.223472132463722, 2.357151716351204, 2.3730638622363656, 2.313547208153507, 2.182278642240312, 2.0452728503122306, 1.9279164930003736, 1.8433784639098634, 1.8076699507050376, 1.7857603737938472, 1.7549087156980685, 1.7202701186500102, 1.6742031610692216, 1.6234732789291013, 1.6055038373780797, 1.6263623269316103, 1.69256717514342, 1.8351758457677287, 2.0004340133073115, 2.1289955819156194, 2.173458864049445, 2.0977573328300085, 1.944787493448179, 1.7599302986197884, 1.5816147502395692, 1.443862437402755, 1.3365164375340444, 1.2542210417094724, 1.185258035175079, 1.1213375574374271, 1.0596427224650145, 0.9894655271291357, 0.9343148838494275, 0.8841844059041496, 0.8408980011169703, 0.8153555516392741, 0.77712215992639, 0.7508687021971843, 0.7347705413230167, 0.7123257625074284, 0.6997857108929589, 0.6856937968305397, 0.6626021448305889, 0.6312790261349708, 0.6072850465979636, 0.567864507202352, 0.5368052589856285, 0.5326912863872157, 0.5582141087971394, 0.6299830440182558, 0.720115748723174, 0.7924764811743044, 0.8062811411614069, 0.787334707648705, 0.7106091809741025, 0.6292057721928113, 0.5553227618734741, 0.5003852535932269, 0.4791365754523358, 0.45711337428391147, 0.47227169340160197, 0.4464582418939512, 0.4008838108240358, 0.35182007771739726, 0.2823472978980242, 0.22294271676391242, 0.177688875389446, 0.15934500769821883, 0.15283656944078436, 0.14979540206976624, 0.15798853870864044, 0.1716046248623979, 0.1617240497641898, 0.1554409196764749, 0.1551826409341482, 0.12212440108432684, 0.09899210608396831, 0.08709450797513986, 0.069975084605282, 0.06888857789419713, 0.07538379774818305, 0.060106463892844054, 0.04903969700546438, 0.049128556424437794, 0.034715943622214626, 0.04378874925638807, 0.03694692568737197, 0.018992186230873148, 0.016662256809373745, 0.01219247359832311, 0.0075799284701044065, 0.009775530263112594, 0.013671439417785265, -0.0009793877694979514, -0.019603584345628988, -0.027934146587577625, -0.03467584204644256, -0.031628802114807585, -0.0019651268158940955, 0.0031542472892356235, 0.01589477039448426, 0.011175819832271703, 0.004505036855485832, -0.009004071554783184, -0.02462783346401739, -0.02351077242593529, -0.02996155259895564, -0.0096733021923099, -0.02350205911572084, -0.011879534308935298, -0.01236798758930022, -0.03127238588529212, -0.02024828166698114, -0.023418148555395327, -0.02318093160730606, -0.0002484310224400282, 0.005756017022915046, 0.013361249871438118, 0.014051490728565812, 0.0005115832228950398, 0.014686037673131374, 0.00986149374430582, -0.012633432275644976, -0.0037733819756610144, -0.024216228199947676, -0.03809634525007328, -0.0002689310142219862, 0.0016250106729653149, 0.0010909828455718546, 0.010895002945306797, -0.003595627588424957, -0.014204346299952824, -0.022342786315738376, -0.017885206918780542, -0.030614782013864392, -0.048289927166425786, -0.02978789209648048, -0.032216728531529966, 0.007889997927850903, 0.0037266131067918867, 0.01214412938415374, 0.01013866577999612, -0.00030019979775574207, 0.04916039631049798, 0.02788791233704273, 0.029298558654322213, 0.0189082891800152, 0.002482592952606906, 0.02176183134839148, 0.011423982978437417, 0.006646069958871979, -0.014440605517120132, -0.01111464946221091, 0.0053782481168627265, -0.004763428975458543, 0.042166922442077114, 0.04057344963103103, 0.024610124666575462, 0.01965818600825279, -0.013412220317672039, -0.01417210170463194, 0.001924199870581562, 0.03428455476090574, 0.03404136819062828, 0.012110093859300066, -0.009168211567350155, -0.01704915407067093, -0.03630708233467275, -0.0010640350119696224, 0.01867599129811249, 0.026331027234676004, 0.037811869809353325, 0.027502195108505188, 0.015114645066578622, -0.024280937313118645, -0.03775204504219293, -0.061065241569420406, -0.06929878506250564, -0.04760699606754217, -0.0813772459216619, -0.06457491141663163, -0.03644361229527094, -0.025854710863836006, 0.034677106972259356, 0.0347512344659542, 0.012044478991961082, -0.016855567338495796, -0.02635810712246815, -0.034638176037959136, -0.04931080720682156, -0.023180991031541847, -0.018706072430049247, -0.035173376628972707, -0.014259848128118018, -0.012548773013092608, -0.03328436695589118, -0.0022315981418272062, -0.01613056932103034, -0.03512365242523112, -0.04227262830242234, -0.06290949278746856, -0.06426657268273134, -0.08034960954799464, -0.027416448166531143, -0.012398782587012727, 0.011294204664155323, 0.028318075596104227, -0.04612177162076009, -0.04264763046545193, -0.02518930042459734, -0.036784566000318604, 0.002728444819674346, 0.03109082965087382, -0.028807508268508284, -0.05854278218754848, -0.022304543157316115, -0.06384737974428505, 0.00031312664730838175, 0.08625750762613756, 0.06345589788076947, 0.0797028106052045, 0.039023242173582925, -0.0040194340864300755, -0.024567198756508535, -0.046306074755731806, -0.07545874792893113, -0.11000453352741804, -0.08730882775559108, -0.09970915749072717, -0.1083992943059125, -0.0752678187966486, -0.08273427504998342, -0.09332340081182539, -0.035581121227181406, -0.02464114971697337, -0.01565161529763444, 0.01694178758131119, -0.024673216762682245, -0.0527404795035317, -0.13918749511882642, -0.13689248654649638, -0.1368738152513097, -0.12223847848556366, -0.06894814564777403, -0.07163306422792635, -0.016460352708239517, 0.019269219131989406, 0.0007307512636522593, 0.0053242104998820336, -0.019741551386681974, -0.04357129594714732, -0.032606406530512444, -0.04306439126756656, -0.052494662833103, -0.0468898620446755, -0.03989861710788867, -0.060520445106696505, -0.06810379250455728, -0.07922815835996076, -0.05404233415375057, -0.006617552485008731, 0.007822757521129226, 0.0385153125472173, 0.014018599869587324, 0.03570966708044792, 0.009966492587340071, 0.022430915133182766, 0.047489056030846084, -0.01981296556357138, 0.012593849034625447, -0.03632622579391642, -0.05105408566445973, -0.0059739146525617836, -0.025248872181091776, -0.06861373515570814, -0.0931629968448598, -0.16095636265884472, -0.11953692187441008, -0.13703178717617584, -0.09787498966045152, -0.03291762000026509, -0.039510315076274345, 0.014452783678493748, 0.010401452894195824, -0.012407894949626115, -0.06581941028068224, -0.03470638026779735, -0.02625779068082451, -0.012855651064119341, 0.007347352592016884, 0.022364702609174978, -0.028754853735309782, -0.05325353832194253, -0.04737131524328885, -0.041435152949554806, -0.010061802435893781, -0.01309234174401523, 0.01038177464161978, -0.006256522553794316, 0.01861947785186535, 0.06802615328591222, -0.009391549201155104, 0.0089609954340762, -0.01752642097352804, -0.033064478366325034, 0.07884041724772482, 0.041510417380815685, 0.07012606571180015, 0.05179277951492146, 0.009236399696613622, 0.01537878122060108, -0.025986214442708534, 0.04333186751210588, 0.04129154425489769, 0.03401816912610726, 0.024188212452394452, -0.05559288583079401, -0.010310668357449307, 0.06515639198330683, 0.10093664616692918, 0.13727113338028335, 0.11176083086071802, 0.04006308816298479, 0.05312502313573901, 0.04350592286552358, 0.0335453431647745, -0.03629560887442465, -0.05086707606566926, -0.047128218267760875, -0.02300051078495332, 0.003981953422003735, -0.015193595954791275, -0.07413797965351307, -0.10077793006454908, -0.06961874542154309, -0.08480419620488844, -0.07998051772407751, -0.03687506054234993, -0.05704503814136076, 0.0022029277038573157, 0.012165019769335211, -0.02609348816062642, -0.014492742372722509, 0.007835111847244815, -0.00618079946917177, -0.02171920762410189, -0.09147052328793727, -0.14699135926076087, -0.18439698436194357, -0.16048287672919304, -0.11796178450135289, -0.08925421901782307, 0.018269376343669524, -0.07336424832980767, -0.03770306553747256, -0.06513836589457632, -0.07894286774142562, -0.1034991083145259, -0.12052637681425568, -0.10460413024437729, -0.08077708921123379, 0.03874339568595994, 0.06663104404536727, 0.06719072131823209, 0.001215296623842227, -0.059473010880979164, -0.0774582115742726, -0.07345210061457812, -0.06077558049493359, 0.028800659232751383, 0.03637101248077918, 0.04587054100166154, 0.008770342137779344, -0.026096097862234633, 0.01167718180186694, -0.03674739625737049, 0.05119518958451774, 0.05106829346994571, 0.020183464800455513, 0.00353727811847548, -0.0035504869293726533, 0.030129747469836536, 0.055606124813770544, 0.09041024245012798, 0.07567566864532188, -0.011508347631405813, -0.044223136967964635, 0.026168130890529724, -0.012633477682001572, 0.13147202398101346, 0.14367600184170182, 0.08773073438997787, 0.029350253496344146, -0.12832360267704623, -0.1947140514856176, -0.16268115084290252, -0.13451929695453085, -0.1154253796700557, -0.056542436512332046, 0.0, 0.0, 0.0, 0.0, 0.0]] caption="Water Vapor Number Density"
  out "NRB HSRL Combined":dbl[][](graph)=[[3.531676609707886e-05, 8.061574065986715e-05, 0.00016344179170028832, 0.0003009082062207329, 0.000493811808511556, 0.0008223864205134831, 0.0012684467983665926, 0.0018343674875886862, 0.0025194771357405312, 0.0033925755089252857, 0.004554285196186569, 0.005950856388546895, 0.0075749989985705824, 0.009601220716645627, 0.01213974382059549, 0.015417534214227929, 0.01917760014105109, 0.023663127634360875, 0.028531485854115347, 0.033435164780009935, 0.0395531467738367, 0.04596018240323892, 0.05355271446329748, 0.06211359773054181, 0.07096669811434725, 0.07965705757789024, 0.0876666974930519, 0.09636728122532447, 0.10456125831305335, 0.11269660456596702, 0.12222476367055601, 0.1311395500446344, 0.1406880879821002, 0.15104620016805184, 0.16077275790183962, 0.16936391305383575, 0.17804585653385074, 0.1874161986441458, 0.19445462379456105, 0.20443145674437624, 0.2127067706339174, 0.2194292481116527, 0.2275147813166004, 0.23172151697900242, 0.23558264536212947, 0.23819885180906342, 0.24172892750410635, 0.24407906172424962, 0.24910975258578105, 0.2532004212823352, 0.25695596200755494, 0.2616753330151798, 0.2643774010606967, 0.26973081943263416, 0.2721375193339814, 0.27543751337424777, 0.27757114226891005, 0.2770867766338415, 0.2769335649297082, 0.28001294109789915, 0.28101385553807223, 0.2803798956057076, 0.2823230307838201, 0.27877689380931103, 0.2766544269900473, 0.27842701343030657, 0.2733437238185507, 0.26936057589567314, 0.2699703285231389, 0.2637307899518629, 0.2626995379139601, 0.2681603848264793, 0.2658710435738473, 0.2681538389819979, 0.2695902847164711, 0.26428648479582484, 0.25918333402960053, 0.2594925909088434, 0.25931701342947316, 0.2628829656161306, 0.2697398647867225, 0.27264877597199927, 0.2786180454881513, 0.29205269937814765, 0.3252498569405913, 0.3814090863698512, 0.47182667044409204, 0.5962682566908027, 0.797955300576425, 1.3183740493913436, 2.380837322937936, 4.01138438222123, 6.110508828771353, 8.376221605832542, 10.778888399741756, 13.589387449693461, 17.36322353991467, 23.25277188830477, 30.714519537230125, 38.58190095028087, 44.64975240907065, 45.30107744249218, 40.52386008260214, 31.951954414874805, 22.352364199157538, 14.90434861196459, 10.152407738150949, 7.687003363199806, 6.546254603104619, 5.568147665297147, 4.462763964347426, 3.2597031309384144, 2.1382421481391836, 1.2734714752113379, 0.6917363768071955, 0.3259600914164094, 0.14507051528035733, 0.05323672210745899, 0.005824930666770837, 0.0020408309402987755, -0.002398649336410658, -0.006835795012773685, -0.017841899989752406, -0.0207757652926152, -0.015759001213820716, -0.015423644087072716, -0.020905447065967694, -0.015475466431209691, -0.014820949732257595, -0.01286845579476302, 0.008890401599736664, 0.009790040243493291, 0.03803884557008005, 0.08997845455472989, 0.1630708922747877, 0.30425925996395575, 0.48789376872070667, 0.7228581704165505, 0.9967253060588264, 1.2550471244945107, 1.4666136349975456, 1.5960417315451763, 1.584000646348964, 1.454582367885092, 1.2739968242856423, 1.0660050825750664, 0.9139713399034067, 0.8483545407758429, 0.8510608864316965, 0.915940296748561, 1.0403291990115375, 1.1592736455822856, 1.2969604732271667, 1.4922504400017442, 1.6928829653520483, 1.931648846349778, 2.1466941330657536, 2.2547356427667045, 2.25934108888167, 2.1985191071480403, 2.0535678698940103, 1.9190809462519638, 1.8385306546246223, 1.758248620545835, 1.722033375642803, 1.7100486865979938, 1.6408259892731523, 1.6004290174831073, 1.5688890752720748, 1.4927391149841311, 1.4822243305917242, 1.4925466807597423, 1.5447426623576304, 1.6822658345336154, 1.8390333892805433, 1.98003017241296, 2.0499149452331387, 2.0116087927817863, 1.8818920743524898, 1.6960391433963309, 1.532214359897392, 1.3752764132157296, 1.283741323793992, 1.2089445494184268, 1.1339173341114988, 1.0680776410566735, 0.9568031080646108, 0.8609487728127759, 0.7676829103689111, 0.6881389613670481, 0.6837922843230365, 0.6550326593822933, 0.650230197976444, 0.6418361628791813, 0.6139254104463531, 0.6050348370968283, 0.5774533610318786, 0.6141837983185974, 0.6128789759316083, 0.6041687057730426, 0.5683483053130848, 0.47984857084465277, 0.4168922925576732, 0.3989322840580105, 0.46373897538460235, 0.555186263149815, 0.6300029096409825, 0.6871283988778601, 0.7273437276274323, 0.6775490147103279, 0.61539622571733, 0.5319696681798262, 0.4202741662630375, 0.3556733322268652, 0.3577064291599813, 0.37745338273603374, 0.3692080934646814, 0.3452738459074838, 0.2987019393882553, 0.204901108161069, 0.13811756708009482, 0.09789746495040876, 0.06369588858453065, 0.0851254896373914, 0.049771985724565614, 0.06616715909107164, 0.045508653618133756, 0.03826015421590885, 0.05579916625908955, 0.04047946747851708, 0.04964437858153962, -0.003920481254164459, -0.03200761170358941, -0.03363614438106183, -0.05551251010515025, -0.05360853977749061, -0.05658761471497385, -0.055793582731741294, -0.06511808042290688, -0.015454242335175401, 0.0065350802447480885, -0.02367319028532979, 0.005383650587619062, -0.08051081211939673, -0.09088128235515767, -0.08326358207337975, -0.09243964459039607, -0.01802168701254031, -0.06009510892052768, -0.06043835623454874, -0.12730285014491113, -0.1732567045335944, -0.16097432034042072, -0.2205102239931707, -0.17528836182137936, -0.2158996279020748, -0.19859830530039155, -0.12650224181619474, -0.15152087533062866, -0.0993888561865209, -0.06503220990567117, -0.0865819341155925, -0.06028301191547161, -0.11624912442569094, -0.18607207104052714, -0.15576861982187543, -0.16639075484229107, -0.13754745811168945, -0.12280749674758697, -0.0954712817437387, -0.1144936513021672, -0.05151464230313125, -0.013800887699379741, -0.06441914495362096, -0.077802665739456, -0.09899148731368074, -0.11005274154848672, -0.11996397627544518, -0.0529760790640059, -0.06639063190050937, -0.10624715596110039, -0.13353495890348904, -0.1625513619742886, -0.16478932238059749, -0.09834480405061008, -0.0870915800982878, -0.05457725401987913, -0.023558560466441572, -0.11810581994775339, -0.0919064868088516, -0.08369502133480551, -0.1312973959791811, -0.1350911912843443, -0.15698645760622135, -0.2170971060130658, -0.24110761957802668, -0.2268871405504334, -0.1990920276831138, -0.17823789338062818, -0.15496759624021444, -0.09382054362331216, -0.14095659329198104, -0.16591998474168732, -0.1266355431253272, -0.12830599040241528, -0.03879693075663992, 0.0030873501169492263, 0.021863414823045, 0.012459375972985434, -0.031073636197037752, -0.07614684270216611, -0.17581366059915515, -0.12257966374534782, -0.10652977795069862, -0.0919393589379882, -0.10418960466607896, -0.14853402723568698, -0.15560650132308554, -0.13052484914634344, -0.047604537244022894, -0.060982227127842216, -0.0522779770285684, -0.07076856836963476, -0.07097159764711837, -0.09312344086973898, -0.10945565943083456, -0.05595611327908435, -0.08542420984907258, -0.051535860778968615, -0.06604002805122486, -0.14422166391773605, -0.09061584699183797, -0.06562686876077772, -0.025795342732587465, 0.059399845204291896, 0.03324831085546676, -0.07231597616102353, -0.07428578947372878, -0.10248101609232989, -0.11503314355154573, -0.017482929484017837, -0.14385006167903397, -0.19239972117888707, -0.1895355216413721, -0.18729663761510418, -0.09532625982081648, -0.08830363134310815, -0.08187532732678537, -0.10054383533312507, -0.09355248193701554, -0.04966285845346254, -0.11912095312066076, -0.13323624432343245, -0.15172886998345647, -0.23313539403329803, -0.14903494278802173, -0.13083263964146513, -0.12868727464633575, -0.085106302760298, -0.07218740559658902, -0.13304893687591104, -0.14894887752017383, -0.18292828901343702, -0.21191754689572054, -0.1936292362507364, -0.1803969726840255, -0.18471256779136655, -0.24367751000854748, -0.17740144979138425, -0.18728340126983503, -0.10140480625042803, -0.15775810019508663, -0.22940283389859986, -0.16731509740258, -0.3876131636330018, -0.2265968605407243, -0.23115640123927553, -0.3270760636590232, -0.12309015635246696, -0.13623045470659, -0.1080864839623596, -0.10193389898435114, -0.154043746581354, -0.1805229578891064, -0.18096490528112386, -0.13671694923363756, -0.11101287173930682, -0.061530502490122846, -0.06830750893541247, -0.2712918883632617, -0.27268491245801324, -0.28685422344212735, -0.3799186508007351, -0.12639984140824773, -0.218179019198421, -0.28305029935710907, -0.08212294128151061, -0.06598864250155385, 0.0023535481489806768, 0.04352579748479461, -0.06554211986945647, -0.05370644925871785, -0.0612716309257711, -0.08156091515528195, -0.08030688410892786, -0.20457780394668731, -0.10380363167084537, -0.024092985899341134, -0.02120457063589285, 0.03005556696974859, -0.017996796655364408, -0.1536576358701627, -0.1329449265184344, -0.12242260141619214, -0.19343502080184155, -0.25190839866467185, -0.2287051108188207, -0.19722311685495295, -0.154781958840542, -0.02790898403739257, -0.12878758368531334, -0.2220200862308351, -0.1225773001187034, -0.12376338767393817, 0.010786604437314261, 0.1831073068870652, -0.015943321950705157, -0.07590004873899277, -0.18189812852326892, -0.31172618173624683, -0.2530834358344872, -0.2385367638650208, -0.2941885485770619, -0.305281403923959, -0.2701309307749537, -0.26304660843227107, -0.07226091338388518, -0.08142777003463683, -0.019016976858571528, 0.00525440846806823, -0.053053681265056794, 0.012983587269094151, -0.033694867856858796, -0.11091231142046352, -0.11875325413737071, -0.10699789430842764, -0.11870084003214688, -0.11089061660156734, -0.23458125283183098, -0.2529148256244628, -0.4288224178313208, -0.2996893523497138, -0.1866837303660876, -0.1791736682699893, 0.17539499897384417, 0.1873795632009268, 0.3310914840217238, 0.3532803030909103, 0.13139290130944103, 0.07206305862225437, -0.20097490869966247, -0.25795209936321317, -0.18418064736444073, -0.12959416597226747, 0.043275254908333616, 0.20422659048073927, 0.28301663927841686, 0.2544567377665192, 0.06947428200142952, -0.14562271687097747, -0.2651097572971141, -0.40487413882842566, -0.32944003738672123, -0.31064453918321194, -0.2888934660311954, -0.15521840703125456, -0.07305960672249047, -0.06592291388501377, -0.11645848600542173, -0.1974364702529806, -0.18370604007000374, -0.1849926324518976, -0.29739630442528847, -0.393620675991152, -0.3846800603005865, -0.2610391360218423, -0.21735702573528842, -0.12034087866859368, -0.23257631624631298, -0.5159023302604658, -0.5643153245622305, -0.5168596231074912, -0.5735629474298685, -0.2932785056082486, -0.26336537431780055, -0.3409789732557187, -0.3068401000097705, -0.3618419426049688, -0.4298641802173086, -0.26253459117819666, -0.21734569261408065, -0.36343194245767735, -0.10426275201842423, -0.30384563314516977, -0.29359381812791696, -0.20214812612039343, -0.31238221851169495, -0.12953733855038707, 0.04195690329174565, 0.09442420519013836, 0.05519411294452378, 0.1257932161948304, 0.051488070825899034, -0.05456135251503387, 0.01703054906720575, -0.27541842933194677, -0.40048747643374033, -0.385762500938531, -0.4402025077536688, -0.19799789145039912, -0.08898929271967145, -0.21237953765015377, -0.17540084678170167, -0.1578743096599539, -0.2742734445622387, -0.002436737171364981, 0.07368037711105412, 0.02071979378917679, 0.0013077537259663333, -0.15740837823375597, -0.030356790602889767, -0.1859405296872888, 0.12706864380343363, 0.17079224816161137, 0.2707909977271951, 0.34732934495585593, 0.15684292416417286, 0.31025532470498407, 0.09959333873238324, 0.1877552065332669, 0.11085521824358033, -0.10488763260890145, -0.06685371471338611, -0.32639774933060184, -0.35629253277281314, -0.2032230352272696, -0.05641430043163983, 0.0779826533670776, 0.1456469760312101, -0.05329683718955327, -0.1523950086848071, -0.2015529406653876, -0.031206672270889402, 0.027637547685797997, -0.07330143093795252, 0.0, 0.0, 0.0, 0.0, 0.0]] caption="Water Vapor Number Density"
  out "CH 1 (WV off) counts display":dbl[][](graph)=[[61.08, 53.08, 57.08, 40.08, 44.08, 51.08, 51.08, 42.08, 46.08, 53.08, 66.08, 61.08, 80.08, 96.08, 78.08, 103.08, 109.08, 125.08, 119.08, 151.07999999999998, 152.07999999999998, 154.07999999999998, 157.07999999999998, 164.07999999999998, 173.07999999999998, 195.07999999999998, 191.07999999999998, 199.07999999999998, 211.07999999999998, 225.07999999999998, 223.07999999999998, 213.07999999999998, 246.07999999999998, 224.07999999999998, 213.07999999999998, 263.08, 219.07999999999998, 234.07999999999998, 223.07999999999998, 217.07999999999998, 211.07999999999998, 202.07999999999998, 211.07999999999998, 225.07999999999998, 245.07999999999998, 216.07999999999998, 167.07999999999998, 226.07999999999998, 190.07999999999998, 201.07999999999998, 194.07999999999998, 191.07999999999998, 176.07999999999998, 162.07999999999998, 168.07999999999998, 171.07999999999998, 164.07999999999998, 169.07999999999998, 144.07999999999998, 159.07999999999998, 148.07999999999998, 146.07999999999998, 138.07999999999998, 143.07999999999998, 115.08, 116.08, 100.08, 112.08, 103.08, 96.08, 95.08, 102.08, 87.08, 75.08, 105.08, 93.08, 77.08, 82.08, 79.08, 69.08, 50.08, 72.08, 66.08, 73.08, 100.08, 83.08, 94.08, 125.08, 128.07999999999998, 180.07999999999998, 133.07999999999998, 171.07999999999998, 160.07999999999998, 187.07999999999998, 217.07999999999998, 194.07999999999998, 226.07999999999998, 495.08, 817.08, 1252.08, 1644.08, 1616.08, 1380.08, 924.08, 435.08, 137.07999999999998, 55.08, 39.08, 64.08, 35.08, 28.08, 24.08, 29.08, 28.08, 28.08, 39.08, 11.079999999999998, 30.08, 36.08, 20.08, 24.08, 21.08, 41.08, 10.079999999999998, 12.079999999999998, 14.079999999999998, 18.08, 32.08, 4.079999999999998, 14.079999999999998, 32.08, 18.08, 28.08, 14.079999999999998, 34.08, 34.08, 97.08, 143.07999999999998, 190.07999999999998, 313.08, 481.08, 573.08, 615.08, 568.08, 482.08, 387.08, 333.08, 299.08, 259.08, 224.07999999999998, 261.08, 329.08, 397.08, 411.08, 511.08, 625.08, 674.08, 725.08, 701.08, 721.08, 676.08, 547.08, 509.08, 451.08, 416.08, 442.08, 383.08, 391.08, 368.08, 398.08, 374.08, 378.08, 368.08, 418.08, 342.08, 422.08, 541.08, 594.08, 585.08, 614.08, 470.08, 420.08, 290.08, 338.08, 267.08, 280.08, 274.08, 288.08, 244.07999999999998, 202.07999999999998, 240.07999999999998, 221.07999999999998, 185.07999999999998, 195.07999999999998, 188.07999999999998, 191.07999999999998, 162.07999999999998, 156.07999999999998, 116.08, 106.08, 93.08, 105.08, 98.08, 100.08, 97.08, 97.08, 122.08, 135.07999999999998, 122.08, 143.07999999999998, 147.07999999999998, 121.08, 84.08, 70.08, 61.08, 64.08, 57.08, 60.08, 49.08, 65.08, 65.08, 50.08, 66.08, 55.08, 52.08, 58.08, 43.08, 26.08, 38.08, 35.08, 47.08, 39.08, 11.079999999999998, 15.079999999999998, 28.08, 16.08, 5.079999999999998, 18.08, 19.08, 13.079999999999998, 6.079999999999998, 25.08, 13.079999999999998, 8.079999999999998, -1.9200000000000017, 5.079999999999998, 11.079999999999998, 3.0799999999999983, 15.079999999999998, -0.9200000000000017, 11.079999999999998, -2.9200000000000017, -7.920000000000002, -7.920000000000002, -8.920000000000002, -4.920000000000002, -5.920000000000002, -7.920000000000002, -8.920000000000002, -6.920000000000002, -0.9200000000000017, -4.920000000000002, -6.920000000000002, -13.920000000000002, -10.920000000000002, -5.920000000000002, 3.0799999999999983, -11.920000000000002, 3.0799999999999983, -3.9200000000000017, -0.9200000000000017, -0.9200000000000017, 9.079999999999998, -3.9200000000000017, -5.920000000000002, 5.079999999999998, 3.0799999999999983, -1.9200000000000017, 5.079999999999998, -0.9200000000000017, 4.079999999999998, 2.0799999999999983, -2.9200000000000017, -5.920000000000002, 1.0799999999999983, 11.079999999999998, -1.9200000000000017, -3.9200000000000017, 2.0799999999999983, -7.920000000000002, 14.079999999999998, 13.079999999999998, -10.920000000000002, 6.079999999999998, -6.920000000000002, -0.9200000000000017, 3.0799999999999983, -0.9200000000000017, 1.0799999999999983, -9.920000000000002, -3.9200000000000017, -6.920000000000002, 1.0799999999999983, -1.9200000000000017, 5.079999999999998, -9.920000000000002, 15.079999999999998, 16.08, 0.0799999999999983, -10.920000000000002, 2.0799999999999983, 4.079999999999998, 7.079999999999998, -4.920000000000002, 1.0799999999999983, 6.079999999999998, -6.920000000000002, 9.079999999999998, 2.0799999999999983, 10.079999999999998, 12.079999999999998, -5.920000000000002, 3.0799999999999983, 0.0799999999999983, 5.079999999999998, -2.9200000000000017, 0.0799999999999983, -1.9200000000000017, 7.079999999999998, -9.920000000000002, 8.079999999999998, 3.0799999999999983, -6.920000000000002, -9.920000000000002, -10.920000000000002, -3.9200000000000017, -12.920000000000002, -3.9200000000000017, -13.920000000000002, -4.920000000000002, -1.9200000000000017, -4.920000000000002, -11.920000000000002, -0.9200000000000017, -1.9200000000000017, 5.079999999999998, -5.920000000000002, 4.079999999999998, -10.920000000000002, -5.920000000000002, -16.92, 3.0799999999999983, -0.9200000000000017, 5.079999999999998, -7.920000000000002, -1.9200000000000017, -5.920000000000002, -1.9200000000000017, 2.0799999999999983, 2.0799999999999983, 1.0799999999999983, -2.9200000000000017, -0.9200000000000017, -10.920000000000002, 2.0799999999999983, -1.9200000000000017, -3.9200000000000017, -2.9200000000000017, -1.9200000000000017, 9.079999999999998, -2.9200000000000017, -2.9200000000000017, 3.0799999999999983, -5.920000000000002, 6.079999999999998, 11.079999999999998, -5.920000000000002, -0.9200000000000017, -6.920000000000002, -12.920000000000002, 0.0799999999999983, -4.920000000000002, 5.079999999999998, -4.920000000000002, 4.079999999999998, -1.9200000000000017, 0.0799999999999983, 6.079999999999998, 7.079999999999998, -6.920000000000002, 9.079999999999998, 13.079999999999998, -12.920000000000002, 2.0799999999999983, 4.079999999999998, -11.920000000000002, 1.0799999999999983, -7.920000000000002, 12.079999999999998, -7.920000000000002, -0.9200000000000017, 9.079999999999998, -7.920000000000002, -4.920000000000002, 10.079999999999998, 7.079999999999998, -8.920000000000002, 2.0799999999999983, 8.079999999999998, -5.920000000000002, -10.920000000000002, -1.9200000000000017, -3.9200000000000017, 1.0799999999999983, 9.079999999999998, 12.079999999999998, -7.920000000000002, -7.920000000000002, 2.0799999999999983, -12.920000000000002, 2.0799999999999983, -11.920000000000002, -9.920000000000002, -17.92, 7.079999999999998, 14.079999999999998, 7.079999999999998, 8.079999999999998, -6.920000000000002, 11.079999999999998, -0.9200000000000017, 8.079999999999998, 5.079999999999998, -5.920000000000002, -3.9200000000000017, -11.920000000000002, -2.9200000000000017, -4.920000000000002, -3.9200000000000017, -8.920000000000002, 1.0799999999999983, -6.920000000000002, -9.920000000000002, -2.9200000000000017, 7.079999999999998, -10.920000000000002, 10.079999999999998, -6.920000000000002, -11.920000000000002, 12.079999999999998, -2.9200000000000017, 5.079999999999998, -6.920000000000002, 9.079999999999998, -20.92, -6.920000000000002, 0.0799999999999983, -0.9200000000000017, -8.920000000000002, 1.0799999999999983, -6.920000000000002, 9.079999999999998, -3.9200000000000017, -8.920000000000002, -16.92, -4.920000000000002, 1.0799999999999983, -19.92, -0.9200000000000017, 11.079999999999998, 1.0799999999999983, 1.0799999999999983, -1.9200000000000017, 4.079999999999998, 2.0799999999999983, -2.9200000000000017, 6.079999999999998, 0.0799999999999983, -3.9200000000000017, 3.0799999999999983, 11.079999999999998, -7.920000000000002, -15.920000000000002, 4.079999999999998, -8.920000000000002, 6.079999999999998, -2.9200000000000017, 2.0799999999999983, -5.920000000000002, -7.920000000000002, 4.079999999999998, 2.0799999999999983, -2.9200000000000017, 1.0799999999999983, -8.920000000000002, -2.9200000000000017, -6.920000000000002, 1.0799999999999983, 7.079999999999998, 2.0799999999999983, -2.9200000000000017, -11.920000000000002, 4.079999999999998, 4.079999999999998, 6.079999999999998, 3.0799999999999983, -1.9200000000000017, -0.9200000000000017, -7.920000000000002, -3.9200000000000017, -10.920000000000002, -14.920000000000002, 3.0799999999999983, 1.0799999999999983, -1.9200000000000017, 5.079999999999998, -2.9200000000000017, -7.920000000000002, -7.920000000000002, -4.920000000000002, 3.0799999999999983, -6.920000000000002, -4.920000000000002, 1.0799999999999983, 1.0799999999999983, 7.079999999999998, 1.0799999999999983, 0.0799999999999983, -5.920000000000002, -6.920000000000002, -1.9200000000000017, 5.079999999999998, 1.0799999999999983, -9.920000000000002, 9.079999999999998, 2.0799999999999983, -9.920000000000002, -6.920000000000002, -3.9200000000000017, -8.920000000000002, -8.920000000000002, 18.08, 7.079999999999998, -5.920000000000002, -1.9200000000000017, 2.0799999999999983, -7.920000000000002, 3.0799999999999983, -3.9200000000000017, 2.0799999999999983, 3.0799999999999983, -4.920000000000002, 5.079999999999998, 6.079999999999998, -8.920000000000002, -0.9200000000000017, 6.079999999999998, 9.079999999999998, 0.0799999999999983, 0.0]] caption="Water Vapor Number Density"
  out "CH 3 (HSRL comb) counts display":dbl[][](graph)=[[208.0, 79.0, 37.0, 69.0, 47.0, 69.0, 24.0, 32.0, 69.0, 87.0, 156.0, 106.0, 105.0, 160.0, 100.0, 152.0, 175.0, 197.0, 190.0, 202.0, 240.0, 232.0, 270.0, 232.0, 272.0, 271.0, 305.0, 320.0, 323.0, 332.0, 318.0, 376.0, 364.0, 378.0, 340.0, 378.0, 401.0, 339.0, 302.0, 350.0, 322.0, 319.0, 363.0, 298.0, 372.0, 294.0, 282.0, 326.0, 280.0, 262.0, 291.0, 294.0, 300.0, 258.0, 226.0, 275.0, 242.0, 246.0, 257.0, 225.0, 198.0, 185.0, 214.0, 148.0, 183.0, 181.0, 175.0, 153.0, 202.0, 175.0, 204.0, 121.0, 90.0, 114.0, 115.0, 82.0, 85.0, 86.0, 90.0, 126.0, 124.0, 122.0, 123.0, 65.0, 115.0, 117.0, 134.0, 195.0, 234.0, 230.0, 184.0, 189.0, 191.0, 210.0, 274.0, 262.0, 289.0, 555.0, 894.0, 1435.0, 1802.0, 1630.0, 1391.0, 961.0, 412.0, 194.0, 37.0, 80.0, 62.0, 83.0, 48.0, 23.0, 26.0, 30.0, 52.0, 67.0, 65.0, 88.0, 51.0, -2.0, 16.0, -21.0, 11.0, -4.0, 16.0, 14.0, 28.0, 18.0, 36.0, 9.0, 2.0, 45.0, 14.0, 29.0, 25.0, 61.0, 113.0, 132.0, 216.0, 324.0, 405.0, 656.0, 650.0, 730.0, 548.0, 398.0, 304.0, 330.0, 283.0, 275.0, 247.0, 287.0, 397.0, 461.0, 444.0, 540.0, 629.0, 701.0, 671.0, 655.0, 634.0, 565.0, 542.0, 473.0, 390.0, 411.0, 424.0, 368.0, 325.0, 370.0, 369.0, 361.0, 371.0, 323.0, 371.0, 402.0, 530.0, 553.0, 499.0, 582.0, 485.0, 361.0, 339.0, 320.0, 291.0, 272.0, 280.0, 253.0, 270.0, 252.0, 229.0, 178.0, 186.0, 211.0, 200.0, 192.0, 187.0, 119.0, 144.0, 147.0, 108.0, 101.0, 112.0, 72.0, 92.0, 112.0, 103.0, 103.0, 122.0, 141.0, 134.0, 130.0, 98.0, 71.0, 73.0, 40.0, 124.0, 66.0, 80.0, 57.0, 61.0, 51.0, 73.0, 28.0, 72.0, 56.0, 38.0, 57.0, 56.0, 23.0, 33.0, 33.0, 26.0, 22.0, 49.0, 23.0, 9.0, -17.0, 58.0, 8.0, 32.0, 22.0, 14.0, -15.0, 24.0, 10.0, 1.0, 40.0, 8.0, 21.0, -17.0, -23.0, 16.0, 27.0, -32.0, 4.0, 16.0, 5.0, -20.0, -44.0, -16.0, -12.0, 18.0, 19.0, -7.0, 12.0, 6.0, -6.0, 29.0, -6.0, -1.0, 8.0, 42.0, -5.0, 26.0, -29.0, -48.0, 17.0, 24.0, 7.0, 39.0, -29.0, 22.0, -42.0, 12.0, -17.0, -2.0, -18.0, -67.0, -4.0, -10.0, 26.0, -14.0, 43.0, 28.0, -30.0, 6.0, 13.0, 0.0, -33.0, -3.0, 32.0, -4.0, 4.0, 1.0, -59.0, 22.0, 1.0, -1.0, -25.0, 12.0, -14.0, 0.0, 1.0, -10.0, 10.0, 10.0, -25.0, -9.0, -5.0, 15.0, 40.0, 8.0, 14.0, 15.0, -16.0, 22.0, -14.0, -17.0, 12.0, -15.0, -18.0, 2.0, 5.0, 36.0, -12.0, -8.0, -3.0, 7.0, -7.0, -9.0, 33.0, -17.0, 31.0, 65.0, 39.0, -19.0, -13.0, -1.0, 18.0, -32.0, -38.0, -5.0, -29.0, -2.0, 27.0, 21.0, 1.0, -6.0, 13.0, 8.0, -51.0, 13.0, 18.0, -2.0, 27.0, 25.0, 24.0, 8.0, 11.0, -2.0, -17.0, -14.0, -24.0, 0.0, 17.0, 2.0, 38.0, 7.0, 18.0, 0.0, 43.0, 3.0, -22.0, 32.0, 21.0, 12.0, 11.0, -20.0, 27.0, 20.0, 15.0, -25.0, 13.0, 17.0, -26.0, -20.0, 51.0, 31.0, -3.0, 2.0, -4.0, 20.0, 5.0, 16.0, 10.0, 0.0, -3.0, -1.0, 2.0, -9.0, -53.0, -14.0, 26.0, 18.0, -3.0, -25.0, 26.0, 34.0, 18.0, -2.0, 1.0, 0.0, 5.0, -17.0, -22.0, -13.0, -30.0, 15.0, -17.0, 6.0, -20.0, 1.0, 6.0, 45.0, -15.0, -5.0, -19.0, -2.0, 34.0, 1.0, 23.0, 31.0, -30.0, 24.0, 22.0, 10.0, 36.0, 0.0, 46.0, -9.0, -27.0, 32.0, -19.0, -4.0, -63.0, -8.0, -6.0, 20.0, 6.0, 32.0, 4.0, -20.0, 17.0, -15.0, -9.0, 20.0, 16.0, -16.0, -3.0, -40.0, -10.0, -5.0, -31.0, 2.0, -8.0, 9.0, 24.0, 19.0, -18.0, 12.0, -11.0, 40.0, -11.0, 13.0, 9.0, 12.0, 1.0, -3.0, -13.0, 7.0, -23.0, -23.0, 1.0, -7.0, 7.0, -25.0, -5.0, -17.0, 48.0, -11.0, 23.0, -1.0, -11.0, -16.0, 8.0, 12.0, 41.0, 2.0, 3.0, 43.0, 17.0, 25.0, -9.0, 36.0, 23.0, -2.0, 19.0, 36.0, -9.0, -2.0, 3.0, 29.0, -2.0, -33.0, 18.0, 7.0, 3.0, 6.0, -4.0, 8.0, 38.0, -3.0, 32.0, -1.0, -11.0, 2.0, 9.0, 32.0, 0.0, -10.0, -49.0, -6.0, 2.0, -10.0, 31.0, -15.0, 25.0, 3.0, 17.0, -14.0, -26.0, 21.0, 5.0, -10.0, 9.0, 8.0, 5.0, -17.0, 0.0]] caption="Water Vapor Number Density"
  out "CH3 (HSRL combined) smooth S":dbl[](array[numeric])=[89.2305681818182, 50.94079545454545, 45.903863636363624, 47.53738636363635, 49.926590909090905, 57.73625, 65.42090909090909, 72.42943181818183, 78.59704545454547, 85.71920454545456, 95.09136363636365, 104.39534090909093, 113.21920454545455, 123.72204545454547, 136.25329545454545, 152.06295454545455, 167.5231818181818, 184.34420454545455, 199.45784090909092, 210.92374999999998, 226.28454545454545, 239.54590909090905, 255.33284090909083, 271.93795454545443, 286.295909090909, 297.077159090909, 303.1595454545453, 309.8470454545453, 313.3953409090908, 315.6282954545453, 320.56863636363624, 322.78170454545443, 325.60556818181806, 329.3044318181817, 330.76181818181806, 329.3527272727271, 327.7788636363635, 327.1112499999998, 322.230568181818, 322.0373863636362, 318.9379545454544, 313.5544318181817, 310.1737499999998, 301.73909090909075, 293.3101136363635, 283.8413636363635, 275.94363636363624, 267.16238636363624, 261.66806818181806, 255.44931818181806, 249.18795454545443, 244.1112499999999, 237.42943181818174, 233.35840909090905, 226.97204545454542, 221.60556818181817, 215.5686363636364, 207.8527272727273, 200.77034090909098, 196.30159090909095, 190.60840909090913, 184.1055681818182, 179.55159090909092, 171.81295454545455, 165.3101136363636, 161.37261363636364, 153.7447727272727, 147.09136363636364, 143.18795454545455, 135.9209090909091, 131.6084090909091, 130.6396590909091, 126.00613636363639, 123.67943181818183, 121.05159090909092, 115.5743181818182, 110.42375000000001, 107.74193181818183, 104.96352272727273, 103.76465909090909, 103.8584090909091, 102.43511363636364, 102.1709090909091, 104.56011363636365, 113.71068181818183, 130.23909090909092, 157.38681818181817, 194.32715909090905, 254.08852272727262, 409.85840909090894, 721.6226136363634, 1183.7845454545454, 1754.0771590909094, 2338.994772727273, 2928.366931818182, 3589.739090909091, 4450.73909090909, 5756.230568181818, 7321.497613636364, 8857.883977272728, 9925.98909090909, 9879.599886363636, 8777.716363636362, 6931.994772727272, 4867.554431818181, 3241.4436363636364, 2191.398181818182, 1638.2476136363637, 1373.489090909091, 1149.832840909091, 907.3498863636364, 652.707840909091, 421.62545454545455, 247.1709090909091, 132.09420454545455, 61.222045454545466, 26.79306818181818, 9.668068181818176, 1.0402272727272697, 0.3584090909090875, -0.4143181818181856, -1.1614772727272773, -2.9825000000000044, -3.417159090909095, -2.5506818181818227, -2.4569318181818227, -3.2779545454545493, -2.3887500000000035, -2.252386363636367, -1.9256818181818212, 1.3101136363636332, 1.420909090909088, 5.437954545454542, 12.670909090909085, 22.622613636363628, 41.582840909090905, 65.69363636363636, 95.89534090909089, 130.28454545454545, 161.66238636363633, 186.19647727272724, 199.7561363636363, 195.49477272727265, 177.07147727272724, 152.99477272727268, 126.3044318181818, 106.84420454545453, 97.84704545454542, 96.84704545454542, 102.8385227272727, 115.24761363636361, 126.72488636363636, 139.90954545454545, 158.86124999999996, 177.8669318181817, 200.3129545454544, 219.74193181818165, 227.8697727272726, 225.47772727272715, 216.69363636363624, 199.93511363636352, 184.57147727272718, 174.67943181818177, 165.03738636363636, 159.69363636363636, 156.68227272727273, 148.55727272727273, 143.18795454545457, 138.71636363636364, 130.44647727272726, 128.0203409090909, 127.41806818181816, 130.34988636363636, 140.31295454545452, 151.62261363636364, 161.38113636363633, 165.18795454545452, 160.29306818181817, 148.3044318181818, 132.19931818181817, 118.13113636363634, 104.88397727272724, 96.84420454545452, 90.21920454545453, 83.7135227272727, 78.01181818181817, 69.14534090909089, 61.562954545454545, 54.318636363636365, 48.182272727272725, 47.37829545454545, 44.915227272727265, 44.12545454545453, 43.10840909090908, 40.81295454545453, 39.81295454545454, 37.6140909090909, 39.602727272727265, 39.122613636363624, 38.18227272727271, 35.562954545454524, 29.730568181818164, 25.577159090909078, 24.236249999999984, 27.898181818181804, 33.07431818181817, 37.16806818181817, 40.1481818181818, 42.091363636363624, 38.83852272727271, 34.94363636363635, 29.92374999999999, 23.420909090909078, 19.63681818181817, 19.565795454545444, 20.454999999999988, 19.82431818181817, 18.369772727272718, 15.747613636363631, 10.704999999999998, 7.151022727272725, 5.023181818181816, 3.2390909090909075, 4.290227272727271, 2.486249999999998, 3.276022727272725, 2.233409090909088, 1.861249999999997, 2.6907954545454507, 1.9351136363636325, 2.352727272727269, -0.18420454545454978, -1.4910227272727312, -1.5535227272727312, -2.542159090909095, -2.4342045454545493, -2.5478409090909135, -2.4910227272727314, -2.8830681818181865, -0.6785227272727317, 0.2845454545454502, -1.0222727272727317, 0.2305681818181775, -3.420000000000005, -3.829090909090914, -3.4796590909090956, -3.831931818181823, -0.7410227272727313, -2.4512500000000044, -2.4455681818181865, -5.1103409090909135, -6.900113636363641, -6.3603409090909135, -8.644431818181822, -6.817727272727277, -8.331931818181824, -7.604659090909095, -4.80636363636364, -5.712613636363641, -3.718295454545459, -2.414318181818186, -3.1898863636363677, -2.2040909090909135, -4.218295454545459, -6.701250000000004, -5.567727272727278, -5.902954545454551, -4.8432954545454585, -4.292159090909095, -3.3120454545454585, -3.9427272727272773, -1.7609090909090954, -0.4682954545454589, -2.1700000000000044, -2.601818181818186, -3.2864772727272773, -3.627386363636368, -3.9256818181818223, -1.721136363636368, -2.141590909090913, -3.4029545454545493, -4.24670454545455, -5.133068181818186, -5.167159090909095, -3.0620454545454585, -2.692727272727277, -1.6756818181818227, -0.718295454545459, -3.5762500000000044, -2.7637500000000044, -2.499545454545459, -3.8944318181818227, -3.979659090909095, -4.5932954545454585, -6.309204545454549, -6.959772727272732, -6.505227272727277, -5.670000000000004, -5.042159090909095, -4.354659090909095, -2.6188636363636406, -3.9086363636363677, -4.570568181818186, -3.4654545454545502, -3.4881818181818227, -1.0478409090909135, 0.08284090909090469, 0.5828409090909048, 0.32999999999999563, -0.817727272727277, -1.9910227272727317, -4.567727272727277, -3.164318181818186, -2.7325000000000044, -2.343295454545459, -2.6387500000000044, -3.7381818181818227, -3.8915909090909135, -3.2438636363636406, -1.1756818181818225, -1.4967045454545498, -1.2751136363636406, -1.7154545454545496, -1.7097727272727317, -2.229659090909095, -2.604659090909095, -1.3234090909090952, -2.008068181818186, -1.204090909090913, -1.5336363636363677, -3.329090909090913, -2.0790909090909135, -1.4967045454545498, -0.5847727272727316, 1.3385227272727231, 0.744772727272723, -1.610340909090913, -1.6444318181818223, -2.255227272727277, -2.516590909090913, -0.38022727272727697, -3.1103409090909135, -4.135909090909095, -4.050681818181823, -3.9796590909090956, -2.0137500000000044, -1.8546590909090952, -1.7097727272727314, -2.0876136363636406, -1.9313636363636408, -1.0194318181818225, -2.4313636363636406, -2.7040909090909135, -3.0620454545454585, -4.678522727272732, -2.9739772727272764, -2.5961363636363677, -2.539318181818186, -1.6700000000000044, -1.4086363636363677, -2.5819318181818223, -2.874545454545459, -3.510909090909095, -4.045000000000004, -3.6756818181818227, -3.405795454545459, -3.4682954545454585, -4.550681818181822, -3.295000000000004, -3.4597727272727314, -1.8631818181818223, -2.883068181818186, -4.170000000000004, -3.02511363636364, -6.971136363636369, -4.053522727272732, -4.113181818181823, -5.789318181818187, -2.167159090909095, -2.385909090909095, -1.883068181818186, -1.7665909090909135, -2.655795454545459, -3.096136363636368, -3.087613636363641, -2.320568181818186, -1.8745454545454587, -1.0336363636363677, -1.1415909090909135, -4.510909090909095, -4.510909090909096, -4.721136363636369, -6.221136363636369, -2.05920454545455, -3.5364772727272773, -4.564886363636368, -1.3177272727272769, -1.0535227272727314, 0.03738636363635939, 0.6879545454545412, -1.0307954545454587, -0.8404545454545498, -0.9540909090909134, -1.2637500000000044, -1.2381818181818225, -3.1387500000000044, -1.5847727272727314, -0.36602272727273155, -0.32056818181818614, 0.4521590909090868, -0.26943181818182244, -2.289318181818186, -1.9711363636363677, -1.8063636363636406, -2.84045454545455, -3.681363636363641, -3.3262500000000044, -2.854659090909095, -2.2296590909090956, -0.40011363636364067, -1.8376136363636406, -3.15295454545455, -1.7325000000000041, -1.7410227272727317, 0.15102272727272295, 2.551590909090905, -0.2211363636363679, -1.0478409090909133, -2.4995454545454585, -4.263750000000004, -3.445568181818186, -3.2325000000000044, -3.968295454545459, -4.098977272727277, -3.6103409090909135, -3.499545454545459, -0.9569318181818226, -1.0734090909090952, -0.24954545454545884, 0.06863636363635939, -0.6898863636363679, 0.16806818181817756, -0.43420454545454973, -1.4228409090909133, -1.516590909090913, -1.3603409090909133, -1.502386363636368, -1.3972727272727314, -2.942727272727277, -3.158636363636368, -5.331931818181823, -3.7097727272727314, -2.3006818181818227, -2.198409090909095, 2.1424999999999956, 2.2788636363636323, 4.008977272727268, 4.258977272727268, 1.5771590909090865, 0.8612499999999955, -2.3915909090909135, -3.0563636363636406, -2.1728409090909135, -1.5222727272727319, 0.5061363636363593, 2.37829545454545, 3.2817045454545415, 2.937954545454541, 0.7987499999999956, -1.6671590909090952, -3.022272727272732, -4.596136363636369, -3.723977272727277, -3.4967045454545493, -3.2381818181818223, -1.7325000000000041, -0.8120454545454588, -0.7296590909090952, -1.2836363636363681, -2.167159090909095, -2.0080681818181865, -2.0137500000000044, -3.223977272727277, -4.249545454545459, -4.135909090909095, -2.7950000000000044, -2.317727272727277, -1.2779545454545498, -2.459772727272732, -5.43420454545455, -5.920000000000004, -5.400113636363641, -5.968295454545459, -3.039318181818186, -2.7182954545454585, -3.505227272727277, -3.1415909090909135, -3.689886363636368, -4.366022727272732, -2.6557954545454585, -2.1898863636363677, -3.6472727272727314, -1.0421590909090952, -3.025113636363641, -2.911477272727277, -1.99670454545455, -3.073409090909095, -1.2694318181818227, 0.4095454545454503, 0.9180681818181775, 0.53454545454545, 1.213522727272723, 0.4947727272727229, -0.5222727272727316, 0.16238636363635944, -2.616022727272732, -3.7893181818181865, -3.6359090909090956, -4.133068181818187, -1.851818181818186, -0.8290909090909133, -1.971136363636368, -1.6217045454545498, -1.4540909090909135, -2.516590909090913, -0.02227272727273155, 0.6709090909090867, 0.1879545454545412, 0.011818181818177509, -1.4171590909090952, -0.27227272727273166, -1.6614772727272773, 1.131136363636359, 1.5146590909090865, 2.3924999999999956, 3.057272727272723, 1.3754545454545415, 2.710681818181814, 0.8669318181818139, 1.6282954545454502, 0.9578409090909049, -0.9029545454545498, -0.5734090909090952, -2.789318181818186, -3.033636363636368, -1.723977272727277, -0.47681818181818625, 0.6567045454545409, 1.2220454545454502, -0.44556818181818625, -1.2694318181818225, -1.6728409090909133, -0.258068181818186, 0.22772727272726845, -0.6018181818181861]
  out "CH3 (HSRL combined) smooth L":dbl[](array[numeric])=[97.9276530612245, 54.374931972789106, 46.824761904761914, 47.954013605442185, 51.966768707482984, 58.3876870748299, 67.33071428571427, 73.84091836734692, 81.045, 90.04414965986398, 100.93190476190479, 112.2346258503402, 124.28734693877558, 136.7201700680273, 149.0152380952382, 162.67085034013616, 176.66489795918375, 191.54329931972796, 205.2796938775511, 218.4837755102041, 231.04670068027212, 243.62493197278906, 257.64789115646244, 271.51013605442154, 284.9106462585031, 297.11302721088407, 307.5586054421766, 316.658945578231, 325.4097959183671, 333.25843537414937, 339.76013605442154, 343.39959183673443, 346.2422789115644, 347.92340136054395, 347.86897959183653, 348.9718707482991, 347.41149659863925, 344.42765306122425, 341.25163265306105, 337.22527210884334, 333.13003401360527, 329.7507823129249, 326.1019727891154, 321.5305442176868, 316.81115646258473, 310.90979591836697, 303.98462585033985, 296.4344557823126, 289.15469387755076, 280.77969387755076, 272.17765306122425, 264.4302040816324, 255.66149659863922, 247.6189795918366, 240.48377551020397, 233.08836734693878, 226.36387755102047, 219.48292517006809, 211.93955782312932, 204.37578231292522, 195.84772108843543, 187.60027210884357, 179.43105442176875, 171.99568027210893, 166.12918367346947, 160.43360544217697, 155.61217687074839, 151.51098639455793, 145.2992517006804, 140.30435374149673, 135.66319727891167, 130.27204081632664, 126.78989795918373, 122.06285714285718, 117.96846938775514, 113.71591836734699, 111.21421768707488, 111.10962585034018, 117.57986394557827, 140.25163265306128, 182.6734013605443, 249.62238095238098, 341.9854761904762, 477.029693877551, 673.857925170068, 940.8477210884355, 1258.903843537415, 1575.6768027210883, 1844.925102040816, 2034.961666666666, 2133.364727891156, 2157.7439795918353, 2138.3213605442165, 2133.1734013605433, 2248.1929591836724, 2560.0926190476184, 3047.3332653061225, 3718.1376870748304, 4410.07306122449, 4953.437857142857, 5237.400442176871, 5031.440408163266, 4376.2754421768705, 3413.666598639455, 2347.2660884353736, 1442.9191496598637, 793.751632653061, 394.67510204081634, 182.56880952380948, 82.7193197278912, 43.020340136054436, 30.2745918367347, 26.770340136054436, 24.195510204081643, 22.837517006802734, 21.749931972789128, 20.46846938775511, 19.945510204081643, 19.08411564625851, 17.944659863945585, 17.135986394557825, 15.980374149659866, 15.262687074829934, 14.035646258503402, 13.740578231292515, 13.898741496598637, 13.359625850340132, 14.2762925170068, 14.869829931972792, 16.345170068027212, 20.288197278911568, 28.173401360544222, 44.58326530612244, 75.44976190476194, 125.36217687074829, 197.03904761904755, 285.49823129251683, 381.1768027210883, 474.2218707482991, 551.7456802721086, 609.0841156462585, 647.2031632653061, 669.1096258503402, 680.5143877551022, 688.8026530612246, 694.2847959183674, 695.104523809524, 689.2490816326532, 674.6776530612246, 654.9667687074832, 635.8094557823131, 622.3987414965987, 616.4387074829932, 617.8961904761904, 625.7405782312924, 634.499931972789, 639.7176190476189, 634.1121768707482, 613.6096258503399, 581.2439795918365, 541.1444897959183, 499.2745918367346, 464.1215306122448, 435.0730612244896, 412.7337755102037, 395.54925170067986, 377.3842857142853, 360.3332653061221, 341.4735714285711, 323.221020408163, 304.82646258503377, 286.2133673469385, 269.98802721088407, 255.25503401360513, 243.21591836734666, 231.85792517006783, 219.43530612244888, 206.50163265306117, 192.39108843537417, 177.68190476190483, 165.18870748299324, 152.05350340136062, 140.92510204081643, 131.74397959183685, 122.57901360544226, 115.59517006802727, 107.7490816326531, 100.1665986394558, 93.18445578231294, 85.36557823129255, 80.32391156462586, 74.75928571428572, 69.7984013605442, 66.43105442176869, 62.19465986394555, 58.77459183673467, 55.449761904761885, 51.87153061224489, 48.889387755102035, 46.642789115646266, 44.6198299319728, 42.58581632653063, 39.72782312925172, 36.85367346938777, 34.97272108843539, 34.05180272108845, 32.53734693877553, 32.45571428571431, 30.907244897959192, 28.0713605442177, 26.687857142857155, 23.713367346938778, 22.135986394557825, 21.45231292517007, 19.927653061224493, 19.238877551020416, 18.76098639455783, 17.476972789115653, 15.875782312925175, 13.926802721088437, 10.457414965986393, 8.442959183673468, 5.7210204081632625, 4.449761904761902, 3.9353061224489783, 3.0211904761904753, 3.9897278911564604, 3.300102040816325, 3.068809523809522, 2.6164285714285693, 1.146190476190475, 0.9854761904761893, 1.6614965986394545, 1.2575850340136043, 2.0951700680272096, 2.1631972789115634, 0.9778231292516993, -0.5476870748299344, -0.9805102040816351, -1.28918367346939, -1.595306122448982, 0.3188095238095227, 0.22697278911564517, -0.20500000000000113, -0.18374149659864059, -0.16928571428571548, 0.5432993197278897, 0.9795238095238081, 0.1725510204081614, -0.06894557823129438, -1.7526190476190495, -2.642925170068029, -3.190544217687077, -3.926938775510206, -3.6080612244897976, -3.3189455782312938, -2.0706462585034022, -2.187142857142858, -1.8410544217687086, -2.3410544217687086, -3.0145238095238107, -3.3376530612244917, -3.470306122448982, -2.5629931972789137, -2.136972789115648, -1.8240476190476207, -1.89122448979592, -2.084251700680274, -1.55278911564626, -1.901428571428573, -1.659931972789117, -1.2534693877551033, -1.8027891156462599, -1.418435374149661, -1.6208163265306137, -1.5578911564625864, -1.3725170068027226, -1.0315306122448993, -1.0902040816326544, -1.8282993197278925, -2.272176870748301, -2.482210884353743, -2.5111224489795934, -1.9575510204081645, -1.3631632653061236, -1.8767687074829946, -1.432040816326532, -1.0332312925170082, -2.2330612244897976, -2.5417346938775527, -2.105510204081634, -2.5417346938775522, -1.3393537414966001, -0.26197278911564736, -1.6599319727891166, -1.7305102040816338, -2.2577210884353756, -2.9771088435374162, -1.8427551020408177, -1.9303401360544232, -1.9771088435374162, -1.7330612244897974, -1.7840816326530629, -1.8648639455782328, -1.155680272108845, -0.13867346938775627, -0.6403741496598653, -0.10806122448979723, -1.2067006802721103, -1.6233673469387768, -0.9558503401360555, -1.5740476190476203, -0.14462585034013714, -0.8827210884353753, -1.5663945578231306, -1.426088435374151, -1.6089115646258516, -1.039183673469389, -0.7934353741496609, -0.7432653061224501, -1.0255782312925181, -0.5578911564625861, -0.8623129251700694, -0.9745578231292531, -2.0060204081632667, -2.4481972789115662, -2.712653061224491, -2.6692857142857154, -2.8572108843537425, -2.7755782312925183, -2.209251700680273, -2.2738775510204094, -1.7364625850340145, -1.9337414965986404, -1.241564625850341, -0.7534693877551032, -0.7670748299319743, -1.1888435374149677, -1.9388435374149677, -2.746666666666668, -1.6641836734693893, -1.138673469387756, -1.2381632653061234, 0.03309523809523718, -0.04343537414966078, -0.007721088435375112, -0.518775510204083, -1.643775510204083, -2.386972789115648, -2.468605442176872, -1.3852721088435385, -1.374217687074831, -1.0774489795918378, -0.7313605442176883, -0.7415646258503416, -0.2670748299319743, -0.2194557823129266, -0.63357142857143, -1.0408843537414976, -1.4677551020408175, -1.9490476190476203, -2.6140136054421785, -2.901428571428573, -1.9864625850340152, -2.150578231292519, -1.352959183673471, -1.2135034013605457, -1.562993197278913, -1.1896938775510215, -1.4269387755102052, -0.9277891156462597, -0.5595918367346953, -0.3095918367346951, -0.8555102040816337, -1.752619047619049, -2.419285714285716, -2.4031292517006815, -1.9252380952380967, -1.0264285714285726, -0.46520408163265425, -0.2619727891156474, -0.13102040816326638, -0.6293197278911576, -1.1182653061224501, -1.1896938775510215, -1.392074829931974, -0.783231292517008, -0.33680272108843684, -0.5987074829931986, -0.30874149659864075, -0.4788095238095251, -0.36741496598639556, 0.7822448979591824, 0.8613265306122435, 0.9718707482993183, 0.8485714285714272, 0.1725510204081619, 0.6147278911564612, 0.41914965986394426, -0.2730272108843551, -0.059591836734694925, -0.34445578231292623, -0.10551020408163372, -0.23476190476190606, -0.21010204081632783, 0.25333333333333197, -0.057891156462586385, 0.8766326530612234, 0.9523129251700668, 0.656394557823128, 1.0288435374149647, 0.6793537414965976, -0.33085034013605547, 0.16319727891156333, 0.4939795918367335, -0.12081632653061347, 1.0024829931972774, 0.04840136054421651, -0.2611224489795932, 0.19040816326530483, -1.4311904761904777, -1.1063605442176887, -1.415884353741498, -1.6854421768707497, -0.7645238095238107, -1.2985374149659878, -1.660782312925172, -1.0434353741496616, -0.7075510204081649, -0.6794897959183689, 0.5092857142857128, -0.17268707482993362, -0.3436054421768724, 0.3417687074829916, -1.351258503401362, -1.0723469387755116, -0.6454761904761919, -1.1072108843537427, -0.034931972789116694, -0.12931972789115753, -0.6786394557823141, -1.0953061224489806, -1.2041496598639467, 0.11132653061224351, 0.5756122448979578, 1.2108163265306109, 0.8485714285714271, -0.3971768707483004, -0.8682653061224501, -1.1854421768707495, -1.359761904761906, -0.5085714285714302, -0.16673469387755288, -0.26622448979592017, 0.46421768707482824, -0.48051020408163403, -1.2330612244897972, -0.3436054421768729, -1.4847619047619074, -1.0289795918367373, -0.6267687074829957, -1.6335714285714302, -0.8461564625850353, -0.22540816326530766, -0.6004081632653075, -0.08340136054421904, 0.33156462585033886, -0.8163945578231303, -0.23731292517006902, -0.028129251700681424, -0.3265986394557835, -0.16928571428571546, -0.2492176870748311, -0.5323809523809535, 0.016088435374148558, 1.037346938775509, 0.8196598639455769, 0.46591836734693737, 0.4038435374149648, -0.4439455782312936, -1.0221768707483005, -0.966904761904763, -1.4677551020408175, -0.8869727891156478, 0.6028231292516992, 1.213367346938774, 1.9012925170068016, 1.7754421768707471, 1.0628571428571416, 1.1011224489795908, 0.43105442176870634, 0.14363945578231188, -0.565544217687076, -0.7764285714285726, -0.9830612244897972, -1.1012585034013618, -1.2662244897959196, -1.8963265306122459, -1.6097619047619058, -1.3129931972789128, -0.41333333333333455, 0.7660884353741482, 0.6478911564625836, 0.6861564625850327, 2.1368367346938757, 2.151292517006801, 2.658945578231291, 2.492278911564624, 1.0135374149659855, 0.23972789115646154, 0.06370748299319628, -0.47030612244898057, 0.474421768707482, 0.9531632653061215, 1.4370068027210872, 1.5628571428571414, 0.9217006802721075, 1.227823129251699, 1.0356462585033999, 1.8188095238095225, 2.221870748299318, 1.9072448979591823, 1.1853061224489783, 0.850272108843536, 0.11812925170067927, 0.7040136054421755, 0.8536734693877538, 0.25843537414965845, 0.3732312925170052, -0.9932653061224503, -0.6072108843537429, -0.22710884353741634, -0.046836734693878807, 0.4344557823129239, 0.24397959183673362, 0.03904761904761794, 0.380034013605441, 0.06965986394557705, 0.15129251700680152, 0.3188095238095226, -0.17948979591836844, 0.027993197278910364, 0.04925170068027093, 0.5960204081632642, 0.5620068027210873, 0.6734013605442166, -0.11486394557823232, -1.1403741496598654, -1.626768707482995, -1.2347619047619063, -0.3002380952380971, 0.23717687074829785, 1.0832653061224478, -0.025578231292517906, -0.4966666666666675]
  out "CH3 Bin Readings":dbl[](array[numeric])=[612.0, 483.0, 441.0, 473.0, 451.0, 473.0, 428.0, 436.0, 473.0, 491.0, 560.0, 510.0, 509.0, 564.0, 504.0, 556.0, 579.0, 601.0, 594.0, 606.0, 644.0, 636.0, 674.0, 636.0, 676.0, 675.0, 709.0, 724.0, 727.0, 736.0, 722.0, 780.0, 768.0, 782.0, 744.0, 782.0, 805.0, 743.0, 706.0, 754.0, 726.0, 723.0, 767.0, 702.0, 776.0, 698.0, 686.0, 730.0, 684.0, 666.0, 695.0, 698.0, 704.0, 662.0, 630.0, 679.0, 646.0, 650.0, 661.0, 629.0, 602.0, 589.0, 618.0, 552.0, 587.0, 585.0, 579.0, 557.0, 606.0, 579.0, 608.0, 525.0, 494.0, 518.0, 519.0, 486.0, 489.0, 490.0, 494.0, 530.0, 528.0, 526.0, 527.0, 469.0, 519.0, 521.0, 538.0, 599.0, 638.0, 634.0, 588.0, 593.0, 595.0, 614.0, 678.0, 666.0, 693.0, 959.0, 1298.0, 1839.0, 2206.0, 2034.0, 1795.0, 1365.0, 816.0, 598.0, 441.0, 484.0, 466.0, 487.0, 452.0, 427.0, 430.0, 434.0, 456.0, 471.0, 469.0, 492.0, 455.0, 402.0, 420.0, 383.0, 415.0, 400.0, 420.0, 418.0, 432.0, 422.0, 440.0, 413.0, 406.0, 449.0, 418.0, 433.0, 429.0, 465.0, 517.0, 536.0, 620.0, 728.0, 809.0, 1060.0, 1054.0, 1134.0, 952.0, 802.0, 708.0, 734.0, 687.0, 679.0, 651.0, 691.0, 801.0, 865.0, 848.0, 944.0, 1033.0, 1105.0, 1075.0, 1059.0, 1038.0, 969.0, 946.0, 877.0, 794.0, 815.0, 828.0, 772.0, 729.0, 774.0, 773.0, 765.0, 775.0, 727.0, 775.0, 806.0, 934.0, 957.0, 903.0, 986.0, 889.0, 765.0, 743.0, 724.0, 695.0, 676.0, 684.0, 657.0, 674.0, 656.0, 633.0, 582.0, 590.0, 615.0, 604.0, 596.0, 591.0, 523.0, 548.0, 551.0, 512.0, 505.0, 516.0, 476.0, 496.0, 516.0, 507.0, 507.0, 526.0, 545.0, 538.0, 534.0, 502.0, 475.0, 477.0, 444.0, 528.0, 470.0, 484.0, 461.0, 465.0, 455.0, 477.0, 432.0, 476.0, 460.0, 442.0, 461.0, 460.0, 427.0, 437.0, 437.0, 430.0, 426.0, 453.0, 427.0, 413.0, 387.0, 462.0, 412.0, 436.0, 426.0, 418.0, 389.0, 428.0, 414.0, 405.0, 444.0, 412.0, 425.0, 387.0, 381.0, 420.0, 431.0, 372.0, 408.0, 420.0, 409.0, 384.0, 360.0, 388.0, 392.0, 422.0, 423.0, 397.0, 416.0, 410.0, 398.0, 433.0, 398.0, 403.0, 412.0, 446.0, 399.0, 430.0, 375.0, 356.0, 421.0, 428.0, 411.0, 443.0, 375.0, 426.0, 362.0, 416.0, 387.0, 402.0, 386.0, 337.0, 400.0, 394.0, 430.0, 390.0, 447.0, 432.0, 374.0, 410.0, 417.0, 404.0, 371.0, 401.0, 436.0, 400.0, 408.0, 405.0, 345.0, 426.0, 405.0, 403.0, 379.0, 416.0, 390.0, 404.0, 405.0, 394.0, 414.0, 414.0, 379.0, 395.0, 399.0, 419.0, 444.0, 412.0, 418.0, 419.0, 388.0, 426.0, 390.0, 387.0, 416.0, 389.0, 386.0, 406.0, 409.0, 440.0, 392.0, 396.0, 401.0, 411.0, 397.0, 395.0, 437.0, 387.0, 435.0, 469.0, 443.0, 385.0, 391.0, 403.0, 422.0, 372.0, 366.0, 399.0, 375.0, 402.0, 431.0, 425.0, 405.0, 398.0, 417.0, 412.0, 353.0, 417.0, 422.0, 402.0, 431.0, 429.0, 428.0, 412.0, 415.0, 402.0, 387.0, 390.0, 380.0, 404.0, 421.0, 406.0, 442.0, 411.0, 422.0, 404.0, 447.0, 407.0, 382.0, 436.0, 425.0, 416.0, 415.0, 384.0, 431.0, 424.0, 419.0, 379.0, 417.0, 421.0, 378.0, 384.0, 455.0, 435.0, 401.0, 406.0, 400.0, 424.0, 409.0, 420.0, 414.0, 404.0, 401.0, 403.0, 406.0, 395.0, 351.0, 390.0, 430.0, 422.0, 401.0, 379.0, 430.0, 438.0, 422.0, 402.0, 405.0, 404.0, 409.0, 387.0, 382.0, 391.0, 374.0, 419.0, 387.0, 410.0, 384.0, 405.0, 410.0, 449.0, 389.0, 399.0, 385.0, 402.0, 438.0, 405.0, 427.0, 435.0, 374.0, 428.0, 426.0, 414.0, 440.0, 404.0, 450.0, 395.0, 377.0, 436.0, 385.0, 400.0, 341.0, 396.0, 398.0, 424.0, 410.0, 436.0, 408.0, 384.0, 421.0, 389.0, 395.0, 424.0, 420.0, 388.0, 401.0, 364.0, 394.0, 399.0, 373.0, 406.0, 396.0, 413.0, 428.0, 423.0, 386.0, 416.0, 393.0, 444.0, 393.0, 417.0, 413.0, 416.0, 405.0, 401.0, 391.0, 411.0, 381.0, 381.0, 405.0, 397.0, 411.0, 379.0, 399.0, 387.0, 452.0, 393.0, 427.0, 403.0, 393.0, 388.0, 412.0, 416.0, 445.0, 406.0, 407.0, 447.0, 421.0, 429.0, 395.0, 440.0, 427.0, 402.0, 423.0, 440.0, 395.0, 402.0, 407.0, 433.0, 402.0, 371.0, 422.0, 411.0, 407.0, 410.0, 400.0, 412.0, 442.0, 401.0, 436.0, 403.0, 393.0, 406.0, 413.0, 436.0, 404.0, 394.0, 355.0, 398.0, 406.0, 394.0, 435.0, 389.0, 429.0, 407.0, 421.0, 390.0, 378.0, 425.0, 409.0, 394.0, 413.0, 412.0, 409.0, 387.0]
  out "CH2 (molecular) smoothed":dbl[](array[numeric])=[24.055714285714288, 14.077823129251705, 11.944319727891157, 10.899251700680274, 10.356734693877552, 9.764897959183674, 9.446020408163267, 9.359285714285715, 9.385646258503403, 10.30826530612245, 11.376292517006803, 12.998741496598642, 15.037857142857149, 16.163707482993207, 18.248741496598655, 19.472380952380963, 21.40690476190477, 24.361836734693885, 26.665408163265308, 30.099081632653053, 32.750442176870735, 34.525952380952354, 37.435816326530585, 39.178163265306104, 41.500442176870735, 42.77850340136053, 44.00809523809523, 44.93921768707482, 45.902653061224484, 48.68071428571428, 49.61353741496598, 50.85248299319727, 51.551462585034, 50.87969387755101, 51.019999999999996, 49.61948979591836, 49.07867346938775, 48.30656462585034, 46.84568027210884, 46.538707482993196, 45.685816326530606, 44.72578231292517, 43.63649659863945, 43.06846938775509, 41.03870748299318, 40.20962585034012, 39.63224489795917, 38.17136054421767, 37.692619047619026, 36.75809523809521, 35.595680272108815, 34.966428571428544, 34.661156462585005, 33.18071428571427, 31.968979591836714, 31.395850340136043, 29.063367346938772, 28.325272108843535, 27.66030612244898, 25.999591836734695, 25.675612244897962, 24.98853741496599, 24.218129251700688, 23.487687074829942, 22.404353741496614, 21.906904761904777, 21.39414965986396, 21.332074829931983, 20.877142857142868, 20.039557823129265, 19.280204081632668, 17.843979591836746, 17.730034013605454, 17.231734693877563, 16.33122448979593, 16.488537414965997, 15.602482993197288, 14.964727891156471, 14.566768707483, 14.616088435374156, 15.020850340136061, 16.29891156462586, 18.002993197278922, 20.78615646258504, 25.509795918367352, 31.425612244897962, 39.7308843537415, 46.731734693877556, 53.372891156462586, 58.261496598639454, 60.13224489795918, 62.013197278911555, 61.51744897959182, 60.8516326530612, 62.85673469387753, 70.31591836734691, 81.82442176870744, 99.43411564625845, 119.47663265306117, 134.63394557823125, 144.19857142857143, 140.18156462585037, 122.79210884353743, 96.76744897959185, 68.04040816326531, 43.598231292517006, 25.72493197278912, 14.668809523809525, 7.948571428571432, 4.788707482993199, 2.981734693877551, 2.8490816326530606, 2.5055442176870746, 2.3524829931972784, 2.990238095238095, 2.241938775510204, 2.8057142857142847, 1.9995918367346934, 1.6160884353741491, 1.9460204081632648, 1.838877551020408, 2.026802721088435, 1.9171088435374148, 1.878843537414966, 1.8873469387755102, 1.59312925170068, 1.6662585034013606, 1.6067346938775509, 1.8516326530612246, 2.1186394557823127, 1.4902380952380956, 1.4052040816326532, 0.8652380952380954, 1.7215306122448977, 3.5038435374149666, 4.911156462585035, 7.224081632653062, 9.36013605442177, 11.684115646258508, 13.548911564625858, 14.388197278911575, 16.07357142857144, 17.224081632653075, 18.107585034013617, 19.45622448979593, 19.642448979591844, 18.668809523809532, 18.52085034013606, 17.677312925170078, 15.814217687074834, 15.49363945578232, 14.750442176870756, 14.843979591836742, 15.015748299319743, 15.342278911564641, 15.19176870748301, 15.127142857142871, 14.43326530612246, 14.040408163265313, 13.252142857142863, 11.98513605442177, 11.793809523809527, 10.997891156462586, 10.176462585034013, 8.827823129251701, 8.503843537414966, 7.843129251700683, 7.389897959183674, 7.634795918367349, 6.988537414965987, 5.512346938775511, 5.692619047619049, 5.347380952380953, 5.204523809523811, 6.344829931972789, 5.8278231292516995, 5.337176870748299, 4.837176870748298, 3.9018027210884343, 3.4825850340136046, 3.691768707482993, 3.714727891156462, 2.9953401360544216, 2.256394557823129, 1.383095238095238, 0.7189795918367348, 0.877142857142857, 1.6934693877551013, 1.2521428571428566, 0.6305442176870741, 0.4477210884353736, 0.772551020408163, 1.204523809523809, 1.5744217687074826, 1.1169387755102038, -0.6203061224489798, -0.98765306122449, -0.6823809523809526, -0.3575510204081635, 0.5931292517006803, 0.3397278911564626, -0.011462585034013525, -0.25721088435374145, -0.8022789115646257, -0.7784693877551019, -0.7087414965986393, -0.38646258503401343, 0.2648979591836735, 0.46897959183673465, 0.8252721088435373, 1.0455102040816326, 0.420510204081633, 0.30911564625850374, 0.11183673469387785, -0.5310204081632651, -1.0964965986394557, -1.3805102040816326, -2.0140136054421767, -1.9765986394557824, -1.9366326530612246, -1.0259183673469385, -1.0395238095238093, -1.9145238095238097, -1.5701360544217688, -1.604149659863946, -1.0412244897959186, -0.7308503401360542, -0.5505782312925168, -0.4876530612244896, -0.4919047619047618, -0.3507482993197278, -0.5429251700680271, -1.7163945578231292, -2.577789115646259, -2.241054421768708, -2.1067006802721093, -1.3048299319727896, -0.3813605442176869, 0.09057823129251717, -0.3337414965986393, -0.6883333333333331, -1.167925170068027, -1.8601020408163262, -1.2674149659863945, -1.4340816326530612, -1.7461564625850339, -1.8456462585034012, -2.056530612244898, -1.6670748299319724, -0.9136734693877551, 0.16625850340136095, -0.12710884353741447, -0.6177551020408157, -1.3754081632653055, -3.453639455782313, -3.2589115646258504, -2.755510204081633, -2.2784693877551025, -1.284421768707483, -1.2716666666666667, -1.4629931972789114, -1.6951360544217686, -0.804829931972789, -0.7929251700680271, -1.195986394557823, -0.39921768707482985, -1.5582312925170072, -1.7002380952380953, -1.159421768707483, -1.9442857142857144, -1.468095238095238, -1.5140136054421764, -2.1330612244897957, -1.8039795918367345, -1.151768707482993, -1.4060204081632652, -0.7087414965986394, -1.5913945578231297, -2.3396938775510208, -1.5021088435374155, -1.761462585034014, -0.5922448979591838, -0.6024489795918367, -1.5794897959183674, -0.7180952380952381, -0.9034693877551021, -0.18323129251700687, 0.7011224489795919, -0.03442176870748284, 0.5608163265306124, -0.2648639455782313, -0.2248979591836736, 0.77, -0.024217687074829936, 0.0786734693877551, -0.19173469387755093, -0.530170068027211, -0.7240476190476193, -0.9272789115646258, -0.7385034013605442, -1.1279591836734693, -0.6874829931972787, -0.3294897959183672, -0.3260884353741495, -0.2852721088435373, -0.6339115646258502, -0.889863945578231, -0.39496598639455766, -0.5922448979591834, -0.1441156462585032, -0.009761904761904694, -1.1067006802721089, -1.665374149659864, -1.7708163265306123, -1.133061224489796, -0.4221768707482993, -0.0905442176870746, -0.309081632653061, -0.4842517006802719, -0.3966666666666664, -0.732551020408163, -0.6551700680272106, -0.5123129251700678, -0.5760884353741494, 0.5761224489795919, 1.0327551020408163, 0.6390476190476191, 0.802312925170068, 0.7121768707482995, 0.46047619047619065, 1.2861564625850341, 0.7147278911564627, 0.5523129251700681, 0.01489795918367337, -0.29292517006802726, -0.28527210884353743, -1.025918367346939, -1.14156462585034, -1.417925170068027, -1.9434353741496597, -1.4587414965986396, -1.3745578231292517, -0.8099319727891154, 0.3686394557823132, 0.4868367346938778, 0.48938775510204097, -0.48850340136054415, -1.377108843537415, -1.5301700680272108, -1.6007482993197277, -1.460442176870748, -0.8490476190476188, -0.31758503401360527, -0.4111224489795918, -0.6245578231292517, -1.3201360544217686, -1.8345918367346938, -1.747006802721088, -1.7640136054421762, -1.559081632653061, -1.7036394557823125, -1.7495578231292517, -1.7138435374149656, -1.7699659863945576, -2.247006802721088, -2.1917346938775513, -2.0888435374149656, -1.707891156462585, -1.2410544217687072, -1.0216666666666665, -0.8507482993197277, -0.8328911564625849, -1.494455782312925, -1.5514285714285714, -2.079489795918367, -2.3388435374149656, -1.6237074829931972, -1.2980272108843534, -0.38306122448979574, -0.19598639455782296, 0.06846938775510222, 0.004693877551020603, 0.030204081632653257, 0.20452380952380966, 0.14244897959183686, 0.002142857142857335, -0.8694557823129251, -1.115204081632653, -1.4026190476190474, -1.4357823129251701, -1.1313605442176868, -1.307380952380952, -1.7342517006802716, -1.7189455782312923, -1.4995578231292517, -1.0327210884353741, -0.7640136054421769, -0.1679251700680271, 0.40095238095238106, -0.037823129251700616, 0.1509523809523811, -0.3022789115646257, -1.0021088435374148, -0.9213265306122448, -1.7886734693877553, -2.0412244897959186, -1.7555102040816328, -1.4017687074829934, -1.0854421768707483, -0.883061224489796, -0.8983673469387756, -1.1441156462585034, 0.016598639455782493, 0.39414965986394573, 0.4783333333333335, 0.013197278911564747, -0.5395238095238094, -0.3439455782312923, -0.31928571428571406, -0.22744897959183663, -0.11775510204081623, -0.07353741496598643, -0.4970068027210884, -0.4425850340136053, -1.0148639455782311, -1.17812925170068, -1.3771088435374148, -1.1313605442176868, -1.1160544217687074, -1.625408163265306, -1.2223469387755102, -1.4757482993197277, -1.1670748299319726, -1.244455782312925, -1.2010884353741496, -0.4919047619047616, -0.025918367346938503, 0.46727891156462603, 0.7589455782312926, 0.3915986394557825, 0.2895578231292519, -0.20278911564625834, -1.0021088435374148, -0.6866326530612243, -0.829489795918367, -0.30823129251700654, -0.403469387755102, -0.8839115646258502, -1.7197959183673472, -2.2368027210884356, -1.2869727891156464, -0.4910544217687075, 0.6390476190476191, 1.3133673469387754, 1.2487414965986394, 0.8788435374149659, 0.570170068027211, 0.223231292517007, -0.32183673469387736, -1.2070408163265303, -1.0599319727891154, -1.7019387755102038, -0.7674149659863946, -0.8133333333333336, -1.4978571428571432, -0.94343537414966, -1.7351020408163262, -1.0641836734693875, -0.37880952380952365, -0.7104421768707481, -0.48085034013605427, -0.6764285714285712, -0.363503401360544, 0.33717687074829955, 0.11013605442176894, 0.7351360544217689, 0.6900680272108843, 0.2853061224489796, 0.13479591836734695, -0.5310204081632652, -0.9697959183673468, -0.7291496598639454, -0.17557823129251682, -0.03612244897959166, 0.7351360544217689, 0.06166666666666665, 0.0004421768707483231, 0.5778231292517008, -0.09309523809523793, 0.23853741496598665, -0.05993197278911544, -1.1101020408163262, -1.1755782312925167, -0.9927551020408161, -0.7282993197278909, -0.024217687074829748, -0.4451360544217686, -0.5021088435374149, -0.36520408163265305, -0.3260884353741496, 0.08292517006802738, 0.029353741496598806, -0.1594217687074828, 0.1237414965986397, 0.5463605442176874, 0.30231292517006847, 0.07697278911564678, -0.13646258503401318, -1.2750680272108843, -0.8779591836734695, -0.7461564625850341, -1.892414965986395, -1.387312925170068, -0.8686054421768709, -0.8354421768707485, 0.1824149659863946, -0.14496598639455793, -0.31418367346938786, 0.25384353741496585, 0.26064625850340123, 0.949421768707483, 0.12034013605442179, -0.7572108843537415, -0.8745578231292517, -0.6764285714285714, -0.5539795918367346, -0.7640136054421769, -1.0565306122448979, -1.8924149659863945, -1.7478571428571428, -0.7852721088435373, -0.9068707482993195, -0.5361224489795916, -0.3779591836734692, -0.6407142857142855, 0.2368367346938778, 0.7725510204081635, 0.2232312925170069, -0.2580612244897958, -1.0556802721088432, -0.6908843537414965, -0.31503401360544186, -0.5539795918367343, -0.692585034013605, -1.3005782312925167, -0.6857823129251701, -0.1398639455782312, 0.9485714285714286, 1.3499319727891157, 0.9273129251700681, 1.0837755102040818, 1.1773129251700682, 0.4485714285714287, 0.8125170068027213, 0.40945578231292534]
  out "CH 2 Bin Readings":dbl[](array[numeric])=[373.0, 310.0, 317.0, 329.0, 302.0, 325.0, 337.0, 333.0, 288.0, 331.0, 317.0, 313.0, 338.0, 324.0, 318.0, 309.0, 316.0, 302.0, 323.0, 358.0, 302.0, 387.0, 368.0, 338.0, 367.0, 341.0, 360.0, 356.0, 370.0, 379.0, 367.0, 349.0, 364.0, 355.0, 363.0, 373.0, 356.0, 330.0, 371.0, 361.0, 305.0, 346.0, 361.0, 364.0, 338.0, 321.0, 328.0, 361.0, 343.0, 364.0, 318.0, 347.0, 381.0, 353.0, 314.0, 310.0, 318.0, 366.0, 297.0, 282.0, 324.0, 326.0, 363.0, 298.0, 319.0, 310.0, 350.0, 317.0, 323.0, 371.0, 340.0, 308.0, 308.0, 358.0, 322.0, 295.0, 313.0, 337.0, 324.0, 313.0, 327.0, 334.0, 280.0, 344.0, 327.0, 326.0, 303.0, 304.0, 293.0, 361.0, 328.0, 286.0, 317.0, 322.0, 331.0, 354.0, 300.0, 335.0, 342.0, 348.0, 337.0, 375.0, 381.0, 305.0, 317.0, 322.0, 348.0, 302.0, 295.0, 308.0, 316.0, 291.0, 314.0, 327.0, 305.0, 333.0, 306.0, 318.0, 312.0, 351.0, 295.0, 314.0, 302.0, 319.0, 305.0, 318.0, 317.0, 320.0, 278.0, 259.0, 286.0, 311.0, 288.0, 316.0, 286.0, 345.0, 314.0, 316.0, 340.0, 318.0, 328.0, 317.0, 341.0, 324.0, 300.0, 326.0, 319.0, 299.0, 340.0, 333.0, 324.0, 292.0, 300.0, 323.0, 325.0, 318.0, 323.0, 341.0, 323.0, 329.0, 327.0, 333.0, 320.0, 296.0, 334.0, 274.0, 297.0, 320.0, 336.0, 312.0, 349.0, 305.0, 307.0, 286.0, 299.0, 306.0, 317.0, 322.0, 303.0, 315.0, 345.0, 295.0, 308.0, 337.0, 316.0, 313.0, 309.0, 332.0, 309.0, 326.0, 308.0, 312.0, 283.0, 327.0, 325.0, 315.0, 308.0, 316.0, 270.0, 302.0, 344.0, 297.0, 318.0, 269.0, 296.0, 299.0, 341.0, 305.0, 287.0, 295.0, 340.0, 305.0, 286.0, 349.0, 308.0, 279.0, 317.0, 324.0, 320.0, 296.0, 285.0, 303.0, 325.0, 312.0, 308.0, 304.0, 302.0, 342.0, 334.0, 319.0, 293.0, 329.0, 320.0, 310.0, 310.0, 299.0, 314.0, 336.0, 309.0, 317.0, 313.0, 313.0, 336.0, 303.0, 281.0, 323.0, 313.0, 312.0, 302.0, 309.0, 281.0, 317.0, 290.0, 308.0, 291.0, 323.0, 291.0, 296.0, 306.0, 277.0, 320.0, 313.0, 295.0, 308.0, 290.0, 293.0, 301.0, 298.0, 288.0, 263.0, 300.0, 340.0, 304.0, 289.0, 313.0, 294.0, 261.0, 356.0, 293.0, 278.0, 276.0, 304.0, 292.0, 290.0, 317.0, 281.0, 325.0, 284.0, 304.0, 306.0, 315.0, 311.0, 321.0, 317.0, 296.0, 302.0, 324.0, 315.0, 328.0, 279.0, 320.0, 303.0, 327.0, 293.0, 312.0, 293.0, 286.0, 314.0, 322.0, 326.0, 301.0, 297.0, 338.0, 303.0, 297.0, 278.0, 298.0, 320.0, 302.0, 336.0, 316.0, 299.0, 305.0, 318.0, 276.0, 310.0, 286.0, 319.0, 323.0, 329.0, 316.0, 300.0, 317.0, 310.0, 277.0, 312.0, 291.0, 302.0, 290.0, 297.0, 323.0, 304.0, 297.0, 288.0, 296.0, 293.0, 298.0, 298.0, 316.0, 280.0, 312.0, 309.0, 311.0, 293.0, 281.0, 303.0, 268.0, 303.0, 303.0, 300.0, 298.0, 307.0, 322.0, 303.0, 335.0, 327.0, 325.0, 298.0, 314.0, 273.0, 338.0, 305.0, 269.0, 275.0, 291.0, 298.0, 283.0, 287.0, 317.0, 328.0, 317.0, 278.0, 335.0, 313.0, 284.0, 281.0, 307.0, 312.0, 278.0, 296.0, 327.0, 277.0, 293.0, 333.0, 280.0, 292.0, 337.0, 309.0, 295.0, 309.0, 329.0, 265.0, 332.0, 286.0, 313.0, 295.0, 322.0, 303.0, 300.0, 273.0, 290.0, 297.0, 300.0, 304.0, 289.0, 288.0, 279.0, 311.0, 303.0, 285.0, 291.0, 300.0, 312.0, 271.0, 310.0, 315.0, 295.0, 290.0, 331.0, 290.0, 301.0, 271.0, 290.0, 342.0, 306.0, 294.0, 278.0, 299.0, 291.0, 296.0, 294.0, 275.0, 303.0, 300.0, 269.0, 294.0, 303.0, 307.0, 289.0, 290.0, 285.0, 279.0, 320.0, 299.0, 307.0, 272.0, 334.0, 315.0, 299.0, 267.0, 322.0, 310.0, 297.0, 299.0, 282.0, 304.0, 290.0, 303.0, 293.0, 287.0, 309.0, 312.0, 312.0, 291.0, 312.0, 319.0, 278.0, 281.0, 285.0, 285.0, 311.0, 293.0, 308.0, 327.0, 284.0, 306.0, 305.0, 361.0, 311.0, 295.0, 317.0, 320.0, 311.0, 335.0, 283.0, 334.0, 290.0, 295.0, 304.0, 293.0, 315.0, 285.0, 297.0, 279.0, 329.0, 321.0, 306.0, 296.0, 288.0, 297.0, 293.0, 303.0, 336.0, 299.0, 264.0, 315.0, 335.0, 281.0, 299.0, 273.0, 311.0, 311.0, 314.0, 295.0, 268.0, 302.0, 272.0, 309.0, 323.0, 303.0, 320.0, 300.0, 320.0, 306.0, 320.0, 324.0, 297.0, 279.0, 308.0, 288.0, 286.0, 300.0, 300.0, 298.0, 295.0, 322.0, 312.0, 282.0, 341.0, 319.0, 306.0, 282.0, 292.0, 293.0, 292.0, 344.0, 286.0, 296.0, 285.0]
  in  "stop":bool
  in  "Reset Average":bool=TRUE
  in  "Save Data?":bool=TRUE
  in  "Collect Data?":bool=TRUE
  in  "ILX Address":i32=6 min=0 step=1
  in  "Lambda On DBR Current":dbl=171.13999999999868
  in  "Lambda Off DBR Current":dbl=172.9499999999997
  in  "Tab Control":T2(tab)=enum."g/m^3"
  out "Water Vapor Number Density":cluster{"Y":dbl[], "Y":dbl[]}[](graph)
  out "Absolute Humidity":cluster{"Y":dbl[], "Y":dbl[]}[](graph)
  out "NRB plot":cluster{"Y":dbl[], "Y":dbl[]}[](graph)
  in  "background length":i32=25
  out "Correction":cluster{"Y":dbl[], "Y":dbl[]}[](graph)
  in  "dead time":dbl=3.7e-08
  out "Optical Depth":cluster{"Y":dbl[], "Y":dbl[]}[](graph) caption="XY Graph"
  out "CH1 RingBuffer long":dbl[][](array[numeric])
  out "CH1 RingBuffer short":dbl[][](array[numeric])
  in  "Weather":T3(tab)=enum."Pulse Energy (Micro Joule)"
  out "Temperature (C)":dbl(graph)=16.945207570207558
  out "Pressure (mb)":dbl(graph)=832.1978021978022
  out "Relative Humdity (%)":dbl(graph)=59.93894993894994
  out "Pulse Energy (Micro Joule)":T4(graph)={"Online Pulse Energy"=5.135471428571428, "Pulse Energy Offline"=5.133192857142857}
  out "?":cluster{"mean":dbl, "mean":dbl}(graph)={"mean"=15378.368918445924, "mean"=113125.65628281415}
  out "Index":i32=764
  out "CH1 (WV off) smooth L":dbl[](array[numeric])=[54.19602272727275, 49.312500000000014, 48.9943181818182, 49.67045454545457, 51.65340909090911, 54.326704545454575, 58.031250000000014, 61.46306818181819, 65.51704545454547, 69.64772727272728, 73.15056818181819, 78.47159090909092, 85.15056818181819, 93.44886363636361, 102.32670454545452, 111.55965909090907, 121.31818181818178, 131.87499999999997, 143.38352272727272, 154.3778409090909, 164.95738636363637, 175.30965909090912, 184.69034090909096, 193.6931818181819, 200.9460227272728, 206.52556818181824, 209.73295454545462, 211.4176136363637, 212.68181818181824, 213.2272727272728, 214.24431818181827, 215.5369318181819, 217.6647727272728, 218.25000000000006, 219.07386363636374, 219.08806818181827, 216.71590909090918, 214.19318181818187, 212.65340909090918, 210.63068181818187, 209.06250000000006, 208.06250000000009, 204.49147727272734, 201.36079545454552, 197.20170454545465, 192.46022727272737, 188.2869318181819, 183.77556818181824, 179.44886363636368, 176.10511363636368, 173.1136363636364, 169.4971590909091, 166.5284090909091, 162.81818181818184, 159.6818181818182, 156.11647727272728, 152.1931818181818, 149.05681818181816, 143.7215909090909, 140.9715909090909, 136.86363636363637, 131.55681818181816, 128.2329545454545, 123.45738636363635, 120.17613636363635, 116.78977272727272, 113.07954545454542, 109.03124999999997, 104.50568181818178, 101.86363636363633, 99.39204545454544, 97.28124999999999, 95.83238636363636, 92.99431818181819, 90.28125000000001, 87.86079545454547, 85.59943181818181, 84.75284090909092, 83.50568181818183, 81.80113636363637, 80.74431818181819, 78.74431818181819, 78.65056818181819, 81.98863636363637, 90.26988636363637, 106.84090909090908, 132.52556818181816, 168.50284090909088, 228.32670454545453, 388.70454545454544, 684.2045454545455, 1098.6420454545455, 1620.4460227272727, 2138.806818181818, 2676.210227272727, 3288.78125, 4077.698863636364, 5260.156250000001, 6602.860795454548, 7948.676136363638, 8885.872159090912, 8771.213068181822, 7779.204545454549, 6101.309659090912, 4236.014204545456, 2835.3210227272734, 1940.6732954545455, 1496.4801136363635, 1276.596590909091, 1067.5596590909092, 852.9971590909091, 617.1477272727273, 399.7670454545453, 246.44318181818178, 138.0255681818182, 67.4659090909091, 36.30965909090909, 19.258522727272727, 8.863636363636358, 6.985795454545451, 6.434659090909088, 5.187499999999998, 5.5340909090909065, 6.2698863636363615, 6.772727272727272, 7.400568181818179, 7.224431818181816, 7.198863636363634, 6.8465909090909065, 7.363636363636362, 8.173295454545453, 9.397727272727266, 13.678977272727266, 20.36079545454545, 31.673295454545446, 50.3125, 74.78409090909093, 105.48011363636371, 139.4488636363637, 170.67897727272734, 196.47159090909093, 209.48011363636365, 205.28409090909093, 187.32954545454552, 159.30681818181827, 131.5511363636365, 112.11363636363649, 102.88920454545465, 103.00284090909102, 110.51136363636375, 121.9289772727274, 133.96590909090924, 147.9232954545456, 164.89204545454555, 186.12784090909096, 208.38636363636368, 228.4090909090909, 239.05965909090907, 237.65909090909088, 228.83238636363632, 213.21022727272728, 197.39772727272734, 183.8210227272728, 173.64204545454555, 168.23011363636374, 164.20170454545465, 159.44602272727283, 154.45170454545467, 148.5511363636365, 142.3693181818183, 139.1562500000001, 139.32954545454555, 143.32386363636374, 153.60227272727283, 165.50568181818193, 174.13068181818196, 175.76136363636377, 167.75284090909105, 153.80965909090924, 137.67045454545467, 122.37784090909102, 110.50852272727286, 101.18750000000009, 93.93465909090915, 87.81818181818184, 82.19602272727272, 76.84943181818181, 71.0028409090909, 66.34090909090908, 62.12499999999999, 58.46874999999999, 56.105113636363626, 52.923295454545446, 50.610795454545446, 49.01988636363637, 47.039772727272734, 45.744318181818194, 44.37215909090911, 42.44886363636364, 40.039772727272734, 38.13636363636364, 35.30965909090909, 33.051136363636374, 32.477272727272734, 33.701704545454554, 37.664772727272734, 42.63636363636364, 46.46875, 46.82670454545455, 45.29261363636364, 40.49431818181819, 35.519886363636374, 31.05681818181818, 27.72443181818182, 26.301136363636367, 24.860795454545457, 25.44886363636364, 23.83806818181818, 21.210227272727266, 18.44602272727272, 14.670454545454536, 11.48011363636363, 9.068181818181811, 8.059659090909086, 7.661931818181813, 7.443181818181813, 7.781249999999995, 8.377840909090903, 7.82670454545454, 7.45738636363636, 7.380681818181815, 5.758522727272726, 4.627840909090908, 4.0369318181818175, 3.215909090909091, 3.139204545454546, 3.4062500000000004, 2.693181818181819, 2.1789772727272725, 2.164772727272727, 1.517045454545454, 1.8977272727272723, 1.5880681818181814, 0.8096590909090905, 0.7045454545454543, 0.511363636363636, 0.3153409090909087, 0.40340909090909066, 0.5596590909090907, -0.039772727272727515, -0.7897727272727275, -1.1164772727272732, -1.3750000000000004, -1.244318181818182, -0.07670454545454575, 0.12215909090909063, 0.6107954545454541, 0.4261363636363633, 0.1704545454545451, -0.3380681818181822, -0.9176136363636368, -0.8693181818181821, -1.0994318181818186, -0.3522727272727276, -0.8494318181818185, -0.4261363636363639, -0.4403409090909094, -1.1051136363636367, -0.7102272727272729, -0.8153409090909094, -0.801136363636364, -0.00852272727272757, 0.19602272727272696, 0.4517045454545452, 0.47159090909090884, 0.017045454545454246, 0.48579545454545425, 0.3238636363636361, -0.4119318181818185, -0.12215909090909127, -0.7784090909090913, -1.2159090909090913, -0.00852272727272757, 0.051136363636363424, 0.03409090909090884, 0.33806818181818155, -0.11079545454545484, -0.4346590909090912, -0.678977272727273, -0.5397727272727276, -0.9176136363636367, -1.4375000000000002, -0.8806818181818185, -0.9460227272727276, 0.23011363636363608, 0.10795454545454519, 0.34943181818181795, 0.289772727272727, -0.008522727272727515, 1.3863636363636362, 0.78125, 0.815340909090909, 0.5227272727272727, 0.06818181818181784, 0.5937499999999997, 0.3096590909090906, 0.17897727272727243, -0.3863636363636367, -0.2954545454545458, 0.14204545454545425, -0.1250000000000003, 1.0994318181818177, 1.0511363636363633, 0.6335227272727268, 0.5028409090909087, -0.3409090909090913, -0.35795454545454586, 0.04829545454545425, 0.855113636363636, 0.8437499999999997, 0.29829545454545425, -0.2244318181818185, -0.4147727272727275, -0.8778409090909094, -0.025568181818182156, 0.44602272727272696, 0.6249999999999997, 0.8920454545454541, 0.6448863636363633, 0.352272727272727, -0.5625000000000002, -0.8693181818181821, -1.397727272727273, -1.5767045454545456, -1.0767045454545456, -1.829545454545455, -1.4431818181818186, -0.8096590909090913, -0.5710227272727276, 0.761363636363636, 0.758522727272727, 0.261363636363636, -0.36363636363636387, -0.5653409090909093, -0.738636363636364, -1.0454545454545459, -0.488636363636364, -0.392045454545455, -0.7329545454545459, -0.29545454545454586, -0.25852272727272774, -0.6818181818181823, -0.045454545454545886, -0.32670454545454586, -0.707386363636364, -0.8465909090909094, -1.2528409090909094, -1.272727272727273, -1.582386363636364, -0.5369318181818185, -0.24147727272727304, 0.21874999999999972, 0.5454545454545452, -0.8835227272727277, -0.8125000000000004, -0.4772727272727277, -0.6931818181818186, 0.05113636363636326, 0.5795454545454543, -0.5340909090909095, -1.079545454545455, -0.4090909090909097, -1.164772727272728, 0.005681818181817677, 1.5568181818181814, 1.1392045454545452, 1.4232954545454544, 0.6931818181818178, -0.07102272727272757, -0.4318181818181821, -0.8096590909090913, -1.3125000000000004, -1.9034090909090913, -1.5028409090909096, -1.7073863636363644, -1.8465909090909096, -1.2755681818181823, -1.394886363636364, -1.5653409090909094, -0.5937500000000003, -0.40909090909090945, -0.25852272727272757, 0.27840909090909055, -0.4034090909090913, -0.8579545454545459, -2.252840909090909, -2.204545454545455, -2.1931818181818183, -1.9488636363636367, -1.0937500000000004, -1.1306818181818186, -0.2585227272727276, 0.30113636363636337, 0.01136363636363602, 0.08238636363636327, -0.3039772727272731, -0.6676136363636367, -0.4971590909090912, -0.6534090909090912, -0.7926136363636367, -0.7045454545454548, -0.5965909090909094, -0.9005681818181821, -1.0085227272727275, -1.1676136363636365, -0.7926136363636367, -0.0965909090909094, 0.11363636363636337, 0.5568181818181814, 0.20170454545454508, 0.511363636363636, 0.14204545454545414, 0.3181818181818179, 0.6704545454545452, -0.27840909090909116, 0.17613636363636337, -0.5056818181818186, -0.7073863636363639, -0.08238636363636387, -0.34659090909090934, -0.9375000000000002, -1.267045454545455, -2.178977272727273, -1.6107954545454548, -1.838068181818182, -1.3068181818181823, -0.43750000000000033, -0.522727272727273, 0.19034090909090884, 0.1363636363636361, -0.16193181818181848, -0.8551136363636367, -0.4488636363636367, -0.33806818181818216, -0.1647727272727276, 0.09374999999999967, 0.2840909090909088, -0.363636363636364, -0.6704545454545457, -0.5937500000000003, -0.517045454545455, -0.12500000000000036, -0.16193181818181854, 0.12784090909090873, -0.0767045454545458, 0.22727272727272696, 0.8267045454545452, -0.11363636363636409, 0.10795454545454503, -0.2102272727272731, -0.394886363636364, 0.9374999999999998, 0.49147727272727243, 0.8267045454545451, 0.6079545454545452, 0.10795454545454516, 0.17897727272727243, -0.301136363636364, 0.4999999999999996, 0.4744318181818178, 0.3892045454545451, 0.2755681818181814, -0.6306818181818186, -0.1164772727272731, 0.732954545454545, 1.1306818181818177, 1.5312499999999996, 1.2414772727272723, 0.4431818181818179, 0.5852272727272725, 0.47727272727272696, 0.3664772727272724, -0.3948863636363641, -0.5511363636363641, -0.5085227272727277, -0.24715909090909133, 0.042613636363636076, -0.16193181818181854, -0.7869318181818186, -1.0653409090909096, -0.7329545454545457, -0.8892045454545459, -0.8352272727272732, -0.3835227272727276, -0.5909090909090913, 0.022727272727272402, 0.12499999999999961, -0.2670454545454549, -0.14772727272727307, 0.0795454545454542, -0.06250000000000033, -0.21875000000000033, -0.9176136363636365, -1.46875, -1.835227272727273, -1.5909090909090913, -1.164772727272728, -0.8778409090909098, 0.17897727272727224, -0.7159090909090915, -0.3664772727272731, -0.6306818181818186, -0.7613636363636367, -0.9943181818181819, -1.1534090909090908, -0.9971590909090908, -0.7670454545454545, 0.3664772727272725, 0.6278409090909087, 0.6306818181818178, 0.01136363636363602, -0.553977272727273, -0.7187500000000004, -0.678977272727273, -0.5596590909090913, 0.2642045454545451, 0.3323863636363633, 0.417613636363636, 0.0795454545454542, -0.2357954545454549, 0.10511363636363602, -0.3295454545454549, 0.4573863636363633, 0.4545454545454542, 0.17897727272727237, 0.031249999999999667, -0.03125000000000033, 0.26420454545454514, 0.48579545454545425, 0.7869318181818179, 0.6562499999999998, -0.09943181818181845, -0.3806818181818185, 0.22443181818181784, -0.1079545454545458, 1.1193181818181812, 1.2187499999999996, 0.7414772727272723, 0.24715909090909038, -1.0767045454545459, -1.6278409090909096, -1.355113636363637, -1.1164772727272732, -0.9545454545454548, -0.4659090909090913]
  out "CH1  Bin Readings":dbl[](array[numeric])=[116.0, 108.0, 112.0, 95.0, 99.0, 106.0, 106.0, 97.0, 101.0, 108.0, 121.0, 116.0, 135.0, 151.0, 133.0, 158.0, 164.0, 180.0, 174.0, 206.0, 207.0, 209.0, 212.0, 219.0, 228.0, 250.0, 246.0, 254.0, 266.0, 280.0, 278.0, 268.0, 301.0, 279.0, 268.0, 318.0, 274.0, 289.0, 278.0, 272.0, 266.0, 257.0, 266.0, 280.0, 300.0, 271.0, 222.0, 281.0, 245.0, 256.0, 249.0, 246.0, 231.0, 217.0, 223.0, 226.0, 219.0, 224.0, 199.0, 214.0, 203.0, 201.0, 193.0, 198.0, 170.0, 171.0, 155.0, 167.0, 158.0, 151.0, 150.0, 157.0, 142.0, 130.0, 160.0, 148.0, 132.0, 137.0, 134.0, 124.0, 105.0, 127.0, 121.0, 128.0, 155.0, 138.0, 149.0, 180.0, 183.0, 235.0, 188.0, 226.0, 215.0, 242.0, 272.0, 249.0, 281.0, 550.0, 872.0, 1307.0, 1699.0, 1671.0, 1435.0, 979.0, 490.0, 192.0, 110.0, 94.0, 119.0, 90.0, 83.0, 79.0, 84.0, 83.0, 83.0, 94.0, 66.0, 85.0, 91.0, 75.0, 79.0, 76.0, 96.0, 65.0, 67.0, 69.0, 73.0, 87.0, 59.0, 69.0, 87.0, 73.0, 83.0, 69.0, 89.0, 89.0, 152.0, 198.0, 245.0, 368.0, 536.0, 628.0, 670.0, 623.0, 537.0, 442.0, 388.0, 354.0, 314.0, 279.0, 316.0, 384.0, 452.0, 466.0, 566.0, 680.0, 729.0, 780.0, 756.0, 776.0, 731.0, 602.0, 564.0, 506.0, 471.0, 497.0, 438.0, 446.0, 423.0, 453.0, 429.0, 433.0, 423.0, 473.0, 397.0, 477.0, 596.0, 649.0, 640.0, 669.0, 525.0, 475.0, 345.0, 393.0, 322.0, 335.0, 329.0, 343.0, 299.0, 257.0, 295.0, 276.0, 240.0, 250.0, 243.0, 246.0, 217.0, 211.0, 171.0, 161.0, 148.0, 160.0, 153.0, 155.0, 152.0, 152.0, 177.0, 190.0, 177.0, 198.0, 202.0, 176.0, 139.0, 125.0, 116.0, 119.0, 112.0, 115.0, 104.0, 120.0, 120.0, 105.0, 121.0, 110.0, 107.0, 113.0, 98.0, 81.0, 93.0, 90.0, 102.0, 94.0, 66.0, 70.0, 83.0, 71.0, 60.0, 73.0, 74.0, 68.0, 61.0, 80.0, 68.0, 63.0, 53.0, 60.0, 66.0, 58.0, 70.0, 54.0, 66.0, 52.0, 47.0, 47.0, 46.0, 50.0, 49.0, 47.0, 46.0, 48.0, 54.0, 50.0, 48.0, 41.0, 44.0, 49.0, 58.0, 43.0, 58.0, 51.0, 54.0, 54.0, 64.0, 51.0, 49.0, 60.0, 58.0, 53.0, 60.0, 54.0, 59.0, 57.0, 52.0, 49.0, 56.0, 66.0, 53.0, 51.0, 57.0, 47.0, 69.0, 68.0, 44.0, 61.0, 48.0, 54.0, 58.0, 54.0, 56.0, 45.0, 51.0, 48.0, 56.0, 53.0, 60.0, 45.0, 70.0, 71.0, 55.0, 44.0, 57.0, 59.0, 62.0, 50.0, 56.0, 61.0, 48.0, 64.0, 57.0, 65.0, 67.0, 49.0, 58.0, 55.0, 60.0, 52.0, 55.0, 53.0, 62.0, 45.0, 63.0, 58.0, 48.0, 45.0, 44.0, 51.0, 42.0, 51.0, 41.0, 50.0, 53.0, 50.0, 43.0, 54.0, 53.0, 60.0, 49.0, 59.0, 44.0, 49.0, 38.0, 58.0, 54.0, 60.0, 47.0, 53.0, 49.0, 53.0, 57.0, 57.0, 56.0, 52.0, 54.0, 44.0, 57.0, 53.0, 51.0, 52.0, 53.0, 64.0, 52.0, 52.0, 58.0, 49.0, 61.0, 66.0, 49.0, 54.0, 48.0, 42.0, 55.0, 50.0, 60.0, 50.0, 59.0, 53.0, 55.0, 61.0, 62.0, 48.0, 64.0, 68.0, 42.0, 57.0, 59.0, 43.0, 56.0, 47.0, 67.0, 47.0, 54.0, 64.0, 47.0, 50.0, 65.0, 62.0, 46.0, 57.0, 63.0, 49.0, 44.0, 53.0, 51.0, 56.0, 64.0, 67.0, 47.0, 47.0, 57.0, 42.0, 57.0, 43.0, 45.0, 37.0, 62.0, 69.0, 62.0, 63.0, 48.0, 66.0, 54.0, 63.0, 60.0, 49.0, 51.0, 43.0, 52.0, 50.0, 51.0, 46.0, 56.0, 48.0, 45.0, 52.0, 62.0, 44.0, 65.0, 48.0, 43.0, 67.0, 52.0, 60.0, 48.0, 64.0, 34.0, 48.0, 55.0, 54.0, 46.0, 56.0, 48.0, 64.0, 51.0, 46.0, 38.0, 50.0, 56.0, 35.0, 54.0, 66.0, 56.0, 56.0, 53.0, 59.0, 57.0, 52.0, 61.0, 55.0, 51.0, 58.0, 66.0, 47.0, 39.0, 59.0, 46.0, 61.0, 52.0, 57.0, 49.0, 47.0, 59.0, 57.0, 52.0, 56.0, 46.0, 52.0, 48.0, 56.0, 62.0, 57.0, 52.0, 43.0, 59.0, 59.0, 61.0, 58.0, 53.0, 54.0, 47.0, 51.0, 44.0, 40.0, 58.0, 56.0, 53.0, 60.0, 52.0, 47.0, 47.0, 50.0, 58.0, 48.0, 50.0, 56.0, 56.0, 62.0, 56.0, 55.0, 49.0, 48.0, 53.0, 60.0, 56.0, 45.0, 64.0, 57.0, 45.0, 48.0, 51.0, 46.0, 46.0, 73.0, 62.0, 49.0, 53.0, 57.0, 47.0, 58.0, 51.0, 57.0, 58.0, 50.0, 60.0, 61.0, 46.0, 54.0, 61.0, 64.0, 55.0]
  out "CH1 (WV off) smooth S":dbl[](array[numeric])=[55.14255102040819, 48.79986394557827, 46.26840136054425, 45.81431972789119, 46.73353741496602, 48.688469387755134, 51.597482993197296, 55.711428571428584, 60.44017006802723, 65.59323129251703, 72.01670068027214, 78.99374149659866, 86.5226530612245, 94.81091836734696, 103.46312925170072, 112.46653061224495, 122.36874149659869, 132.72928571428577, 142.2207823129252, 151.7241836734694, 159.7411904761905, 167.6519047619048, 175.56176870748303, 183.05581632653065, 190.0005442176871, 195.8976530612245, 200.56091836734697, 204.56346938775516, 207.11534013605447, 210.15020408163272, 212.6093877551021, 214.5685714285715, 217.02605442176878, 217.30496598639462, 217.6638095238096, 217.28200680272116, 216.6723129251701, 215.7292857142858, 215.20632653061233, 213.99629251700685, 212.58642857142863, 211.5889795918368, 209.64765306122456, 207.72163265306128, 205.32792517006808, 202.02775510204089, 198.1910204081633, 193.10088435374152, 188.22928571428574, 183.19612244897965, 178.3389795918368, 174.217380952381, 169.54051020408167, 165.1935714285715, 160.79986394557827, 156.5566666666667, 152.09238095238095, 147.13574829931974, 141.6476530612245, 136.24374149659866, 131.15700680272113, 126.1187414965987, 121.75139455782319, 117.18251700680278, 112.64510204081638, 108.75479591836739, 105.21653061224492, 101.81091836734697, 99.3364285714286, 96.61704081632655, 93.99034013605444, 91.65785714285717, 88.24459183673471, 85.82962585034015, 83.29986394557824, 80.99374149659864, 79.84663265306123, 80.59153061224491, 87.99884353741497, 108.92486394557824, 147.88319727891155, 206.49884353741498, 288.51500000000004, 409.3840476190477, 584.7692517006803, 817.2709523809526, 1086.588979591837, 1348.757346938776, 1569.2598979591842, 1720.854285714286, 1802.4350680272112, 1829.1901700680273, 1824.6008843537413, 1840.185068027211, 1973.1655102040809, 2276.0192517006785, 2713.7318367346916, 3294.2173809523783, 3850.1604081632627, 4243.164659863944, 4419.618741496597, 4204.855986394556, 3641.5736734693855, 2849.683367346937, 1970.631496598638, 1214.3347278911556, 666.673163265306, 328.14850340136053, 150.97333333333333, 68.17996598639459, 35.47673469387756, 25.274353741496608, 22.486088435374157, 21.23863945578232, 19.970782312925174, 18.40615646258504, 17.541360544217696, 16.685068027210896, 16.017551020408174, 15.58217687074831, 15.09748299319729, 14.451224489795925, 14.140000000000004, 13.818571428571428, 13.437619047619044, 13.269251700680265, 13.2088775510204, 13.562619047619048, 14.312619047619048, 15.872993197278916, 19.62129251700681, 27.64510204081634, 45.25139455782315, 76.62384353741498, 126.59153061224494, 197.90020408163267, 284.3194217687075, 377.5796258503401, 466.3619387755101, 540.3687414965984, 596.2598979591836, 632.7352380952382, 654.8330272108843, 666.8899999999999, 674.3075170068028, 679.4716326530612, 678.7114285714285, 671.5175510204081, 656.6765646258502, 637.4962925170066, 620.6519047619047, 609.4418707482993, 604.967380952381, 607.6927210884354, 615.5872789115646, 623.64, 627.4988435374149, 621.124693877551, 602.0821768707483, 570.5447619047618, 531.8194217687073, 492.6723129251699, 456.626394557823, 428.4571768707482, 407.04391156462583, 389.36619047619047, 373.12639455782306, 357.3228231292516, 340.16040816326523, 321.9801360544217, 303.13999999999993, 283.8925510204081, 266.3313265306122, 253.1340476190476, 241.98268707482998, 231.99629251700685, 220.80241496598643, 206.77010204081637, 192.7343877551021, 178.9299659863946, 166.2139795918368, 154.61789115646263, 143.6348979591837, 133.30921768707483, 124.43676870748298, 116.09408163265306, 109.00734693877553, 102.35343537414968, 94.8253741496599, 88.61023809523812, 82.46653061224491, 77.01074829931974, 72.73948979591839, 68.61023809523813, 64.75989795918372, 60.8517346938776, 57.723333333333386, 54.52435374149665, 51.62724489795923, 49.68846938775514, 47.25649659863949, 44.65020408163268, 41.89765306122452, 39.17741496598642, 36.877244897959216, 35.42486394557825, 34.79136054421771, 33.684217687074856, 32.61448979591839, 30.850034013605452, 28.300714285714292, 25.74969387755102, 23.80581632653061, 22.675714285714285, 22.29476190476191, 22.139149659863946, 21.764149659863953, 20.560918367346943, 18.583027210884357, 16.43421768707483, 13.501394557823128, 11.381496598639453, 9.58727891156462, 8.230986394557819, 7.780306122448978, 6.968231292517006, 6.622993197278911, 6.363639455782312, 5.868741496598639, 5.511598639455781, 5.1051360544217665, 4.359387755102039, 3.9733333333333314, 3.602585034013604, 3.192721088435374, 3.3321768707482984, 2.941870748299319, 2.412108843537415, 2.1272448979591836, 1.4690816326530627, 1.3814965986394574, 1.3789455782312943, 1.1859183673469407, 1.329625850340138, 1.4350680272108867, 1.313469387755104, 1.0252040816326549, 0.8534353741496618, 0.6221428571428584, 0.44612244897959286, 0.5064965986394568, 0.3423809523809531, -0.14401360544217623, -0.058979591836734, -0.034319727891155796, -0.5020068027210879, -0.544523809523809, -0.6099999999999994, -0.7732653061224483, -0.3242857142857136, -0.022414965986393795, 0.05071428571428646, 0.37724489795918437, 0.17656462585034086, -0.027517006802720373, -0.14656462585033941, -0.6159523809523801, -0.33193877551020323, -0.2766666666666659, -0.010510204081631863, 0.3134693877551027, -0.030918367346938064, -0.08534013605442098, -0.5929931972789106, -0.6516666666666657, -0.4935034013605435, -0.23755102040816256, 0.020102040816327212, 0.1638095238095244, 0.1323469387755108, -0.2154421768707476, -0.47734693877550954, -0.9441836734693867, -0.843843537414965, -0.6099999999999991, -0.430578231292516, 0.16636054421768776, 0.36789115646258574, 0.37469387755102107, 0.49034013605442245, 0.07622448979591909, -0.2196938775510197, -0.3021768707482987, -0.42632653061224435, -0.16952380952380885, 0.04051020408163332, 0.006496598639456452, -0.024115646258502724, -0.08534013605442109, -0.17462585034013547, 0.07282312925170123, 0.011598639455783072, -0.30472789115646176, -0.3753061224489787, -0.8387414965986382, -0.8378911564625839, -0.745204081632652, -0.7111904761904752, -0.439931972789115, -0.2418027210884347, -0.15506802721088375, -0.21204081632653, -0.24350340136054355, -0.2239455782312919, -0.5334693877551011, -0.35234693877550904, -0.17037414965986278, -0.23159863945578119, 0.3678911564625859, 0.3109183673469394, 0.09153061224489858, 0.1663605442176877, -0.0113605442176865, -0.1950340136054416, -0.250306122448979, -0.2418027210884347, -0.2205442176870741, 0.01329931972789214, 0.1195918367346948, 0.007346938775510986, -0.09384353741496523, -0.2307482993197274, -0.10064625850340082, 0.25904761904761986, 0.39425170068027293, 0.46057823129251796, 0.47928571428571515, 0.09238095238095308, -0.08278911564625781, -0.08619047619047551, -0.29452380952380885, -0.39231292517006733, -0.4297278911564619, -0.2834693877551012, -0.25710884353741414, 0.09918367346938894, 0.16040816326530732, -0.05557823129251595, -0.2290476190476181, -0.576836734693877, -0.47649659863945515, -0.32258503401360494, -0.2154421768707476, -0.13551020408163197, -0.1253061224489789, -0.47649659863945504, -0.5275170068027204, -0.4535374149659856, -0.3115306122448972, -0.0003061224489789155, 0.5906802721088444, 0.7709523809523818, 0.3551360544217696, 0.17146258503401457, -0.015612244897958483, -0.29622448979591764, 0.1280952380952387, 0.2735034013605448, -0.16017006802721026, -0.10999999999999935, -0.3302380952380946, -0.6108503401360538, -0.44758503401360483, -0.26901360544217623, -0.27496598639455716, -0.015612244897958608, 0.009047619047619686, -0.22819727891156402, -0.4297278911564618, -0.34129251700680185, -0.6533673469387744, -0.3183333333333322, -0.16442176870748193, -0.28091836734693776, -0.07003401360544151, -0.23414965986394498, -0.20438775510204027, -0.3395918367346933, -0.29027210884353694, -0.3880612244897954, -0.35999999999999943, -0.33619047619047565, -0.21289115646258439, -0.10829931972789054, -0.004557823129251085, 0.2241836734693884, 0.37044217687074893, 0.3500340136054429, 0.1595578231292524, -0.19503401360544156, -0.22139455782312853, -0.22139455782312858, -0.20608843537414898, 0.20972789115646354, 0.297312925170069, 0.33132653061224593, 0.4163605442176882, 0.2871088435374159, 0.30751700680272176, 0.17316326530612308, 0.21142857142857197, 0.29986394557823187, -0.11850340136054363, 0.10258503401360602, -0.024965986394557133, -0.008809523809523129, 0.20547619047619117, 0.02265306122449045, 0.11363945578231349, -0.019013605442176267, -0.18312925170067967, -0.15251700680272046, -0.20438775510204021, -0.10744897959183619, 0.1476530612244904, 0.26414965986394623, 0.09153061224489872, 0.10598639455782402, -0.12190476190476102, -0.0020068027210876915, -0.05132653061224418, -0.2239455782312919, 0.04476190476190536, -0.34639455782312856, -0.3634013605442168, -0.11170068027210789, -0.09299319727891037, 0.10173469387755213, 0.3304761904761913, 0.16295918367347012, -0.076836734693877, 0.20717687074830002, 0.1323469387755109, 0.12639455782313003, -0.12020408163265223, -0.2792176870748291, -0.06068027210884272, -0.14656462585033936, 0.22248299319727965, -0.09129251700680209, -0.02666666666666602, -0.12870748299319656, -0.013061224489795215, 0.4435714285714294, 0.2726530612244907, 0.5983333333333345, 0.4350680272108855, 0.21568027210884447, 0.30496598639455874, 0.009897959183674032, -0.280918367346938, -0.524965986394557, -0.7213945578231284, -0.6839795918367338, -0.3651020408163259, -0.22564625850340078, -0.055578231292516454, 0.049863945578231865, -0.06238095238095177, 0.16976190476190545, 0.04646258503401432, -0.10234693877550954, 0.08812925170068095, -0.18142857142857075, 0.1714625850340143, 0.6314965986394565, 0.5098979591836741, 0.5184013605442181, 0.23523809523809583, -0.3855102040816319, -0.6754761904761895, -0.26901360544217573, -0.06833333333333227, 0.2896598639455792, 0.598333333333334, 0.4010544217687081, 0.21823129251700746, 0.08472789115646316, -0.02156462585033954, -0.32428571428571373, -0.20353741496598585, -0.3089795918367341, -0.282619047619047, -0.2171428571428565, -0.24265306122448915, -0.07258503401360485, 0.31261904761904846, 0.7080272108843548, 0.5447619047619059, 0.37299319727891267, 0.05836734693877642, -0.15931972789115578, -0.21119047619047554, -0.060680272108842886, -0.2979251700680265, -0.286870748299319, -0.10914965986394484, -0.006258503401359847, -0.3098299319727881, -0.4271768707482983, -0.779217687074829, -0.839591836734693, -0.5513265306122443, -0.5351700680272103, -0.16952380952380888, -0.07173469387755033, 0.15955782312925232, 0.019251700680272738, -0.250306122448979, -0.31748299319727835, -0.49860544217687014, -0.7358503401360538, -0.3081292517006794, -0.4229251700680263, 0.05071428571428707, 0.4877891156462599, 0.16040816326530724, -0.013061224489794687, -0.095544217687074, -0.04197278911564545, -0.05557823129251624, 0.032006802721089134, 0.010748299319728538, -0.13125850340135983, 0.40105442176870837, 0.21823129251700768, -0.3098299319727881, -0.42377551020408055, -0.7349999999999991, -0.551326530612244, -0.21969387755101966, -0.1848299319727884, -0.37105442176870673, -0.09554421768707383, -0.09809523809523713, -0.21799319727891053, -0.13891156462584936, -0.2970748299319721, -0.3497959183673462, -0.1491156462585027, 0.09153061224489858, 0.42401360544217764, 0.5719727891156471, 0.9486734693877562, 0.9112585034013616]
  out "CH0 (WV on) smoothed":dbl[](array[numeric])=[49.069523809523794, 41.67751700680271, 38.16391156462584, 36.35863945578231, 35.50744897959183, 35.93687074829931, 37.170714285714276, 38.89350340136053, 41.111190476190465, 44.268503401360526, 47.316972789115624, 50.925816326530594, 54.68942176870746, 58.43176870748297, 62.731088435374126, 66.89095238095234, 71.70727891156459, 76.17071428571424, 80.4997959183673, 84.57292517006798, 88.00149659863939, 90.94112244897953, 93.81017006802715, 95.98789115646252, 98.05421768707478, 100.02955782312921, 101.24979591836731, 102.33993197278906, 102.32972789115642, 102.17241496598635, 101.27530612244892, 100.2702040816326, 99.3280272108843, 97.77190476190471, 96.51170068027206, 95.05081632653055, 93.21833333333328, 91.82377551020403, 90.37989795918362, 88.62054421768703, 87.2685034013605, 85.3952040816326, 83.96153061224484, 82.29061224489791, 79.7310884353741, 77.57972789115641, 74.6622108843537, 71.74979591836731, 69.25489795918364, 66.9292176870748, 64.72258503401358, 62.446224489795895, 60.36204081632651, 57.994693877551, 55.57972789115644, 53.538061224489766, 52.02700680272106, 49.93517006802718, 47.72513605442175, 45.832278911564615, 43.09758503401359, 41.37394557823128, 39.3195238095238, 37.48789115646258, 36.09248299319727, 34.2319387755102, 33.419013605442174, 32.07802721088435, 31.137551020408168, 30.24044217687075, 29.058469387755103, 28.011700680272114, 27.29146258503402, 26.222585034013612, 25.322925170068032, 24.638401360544226, 23.537210884353748, 23.665612244897964, 25.614591836734697, 31.657959183673473, 42.74129251700681, 59.56272108843538, 83.16221088435375, 117.90370748299321, 168.68261904761903, 236.51595238095237, 316.32802721088433, 395.0763265306122, 462.2370408163265, 508.2685034013606, 530.7132312925171, 534.7174829931973, 525.7778571428573, 522.8450340136056, 555.210680272109, 638.8909523809526, 766.5950340136056, 940.3909523809526, 1109.9479251700684, 1234.1622108843542, 1288.7514965986397, 1221.3518367346942, 1049.2804081632657, 808.3118707482995, 549.4045578231294, 332.51595238095246, 178.89860544217692, 86.4547278911565, 39.237891156462574, 17.16986394557822, 8.544013605442176, 6.241292517006803, 5.4020068027210915, 4.887551020408167, 4.649455782312929, 3.8815986394557846, 3.8135714285714313, 3.869693877551023, 3.783809523809527, 3.9156122448979627, 3.4972448979591864, 3.1979251700680296, 2.9462244897959193, 2.898605442176872, 2.9615306122448994, 2.9802380952380965, 2.9275170068027214, 2.8569387755102045, 2.973435374149661, 3.4224149659863956, 4.2787074829932, 6.102687074829932, 9.79231292517007, 16.40880952380952, 27.896904761904757, 44.40540816326529, 64.14860544217686, 85.76850340136053, 105.3926530612245, 121.43091836734698, 133.5287074829933, 141.17921768707492, 146.1562585034015, 149.0329591836736, 151.48789115646272, 152.97853741496613, 153.20642857142872, 151.4173129251702, 147.9708843537416, 143.95557823129263, 140.02785714285724, 137.75404761904772, 136.3535374149661, 136.67156462585046, 138.2676530612246, 140.11374149659875, 140.8850000000001, 139.258299319728, 134.3382312925171, 126.49044217687083, 117.54486394557827, 108.41561224489796, 100.45812925170065, 94.95047619047615, 90.02190476190471, 85.98193877551016, 82.31187074829927, 78.24979591836728, 74.34503401360539, 70.57292517006796, 66.11969387755096, 61.828027210884315, 58.458979591836695, 55.34418367346936, 53.065272108843494, 50.89605442176867, 48.381598639455746, 45.13499999999996, 42.076326530612214, 38.466632653061204, 35.60353741496598, 33.38244897959183, 31.042312925170066, 29.312721088435374, 27.33057823129252, 25.35693877551021, 23.43942176870749, 21.634149659863944, 20.126496598639456, 18.54231292517007, 17.31187074829932, 16.07462585034014, 14.75744897959184, 14.061020408163268, 13.760000000000002, 13.15795918367347, 12.337380952380952, 11.703027210884354, 10.709829931972788, 10.382448979591835, 10.239591836734691, 9.62054421768707, 9.00319727891156, 8.532959183673462, 7.862040816326524, 7.795714285714279, 7.594183673469384, 7.158809523809523, 6.953877551020408, 6.560170068027213, 6.0261564625850355, 5.407108843537416, 5.078027210884354, 4.677517006802723, 4.940272108843539, 4.8135714285714295, 4.463231292517008, 4.093333333333335, 3.4096598639455795, 3.24044217687075, 3.0635714285714295, 2.597585034013606, 2.286360544217689, 1.6953741496598655, 1.191122448979593, 0.9861904761904775, 0.8042176870748312, 0.8935034013605455, 0.8084693877551032, 1.0644217687074837, 0.9224149659863949, 0.8322789115646259, 0.6792176870748299, 0.29741496598639466, 0.37309523809523826, 0.3892517006802722, 0.5185034013605443, 0.43431972789115664, 0.38755102040816347, 0.11204081632653089, -0.18472789115646238, -0.16346938775510184, -0.2910204081632652, -0.22724489795918357, -0.03676870748299313, 0.29401360544217714, 0.2668027210884357, 0.1154421768707487, 0.160510204081633, -0.08693877551020388, -0.02486394557823104, 0.19537414965986424, 0.15115646258503437, -0.02401360544217654, -0.16857142857142832, -0.11585034013605416, -0.20853741496598613, -0.2714625850340133, -0.10819727891156439, -0.16687074829931947, -0.18982993197278894, 0.05931972789115662, -0.02231292517006782, -0.09969387755102022, -0.06993197278911545, -0.0954421768707481, -0.1201020408163263, -0.177925170068027, 0.013401360544217936, 0.011700680272109104, 0.19877551020408188, 0.4028571428571432, 0.20217687074829963, -0.15156462585033983, -0.51891156462585, -0.7553061224489793, -0.5537755102040813, -0.17707482993197252, -0.09459183673469365, 0.17326530612244925, -0.06653061224489759, -0.18557823129251666, -0.05207482993197245, -0.003605442176870366, 0.36629251700680304, 0.34928571428571464, 0.39435374149659896, 0.1919727891156466, 0.034659863945578455, 0.023605442176870967, -0.023163265306122234, 0.1392517006802723, 0.13244897959183696, 0.12479591836734719, 0.03380952380952404, -0.4372789115646255, -0.5673809523809521, -0.746802721088435, -0.5988435374149655, -0.23659863945578197, 0.1222448979591842, 0.41816326530612297, 0.2685034013605449, 0.22003401360544286, 0.16391156462585083, -0.13370748299319676, -0.012108843537414614, 0.13414965986394597, -0.0027551020408159432, 0.1851700680272112, -0.16346938775510156, -0.2680612244897955, -0.2297959183673465, -0.11840136054421728, 0.34588435374149684, 0.15200680272108866, -0.16602040816326505, -0.16346938775510178, -0.5036054421768704, -0.29017006802721057, -0.09799319727891112, -0.21959183673469343, 0.054217687074830274, 0.13159863945578265, 0.14775510204081652, 0.07632653061224506, 0.11204081632653076, -0.34884353741496543, -0.3148299319727886, -0.3598979591836728, -0.5928911564625843, -0.5886394557823125, -0.5962925170068023, -0.5741836734693875, -0.755306122448979, -0.4500340136054416, -0.20173469387755033, 0.13414965986394625, 0.35013605442176915, 0.18772108843537452, -0.22809523809523785, -0.5903401360544215, -0.46789115646258467, -0.3420408163265303, -0.16431972789115612, -0.2748639455782311, -0.30037414965986375, -0.18472789115646232, -0.14901360544217662, 0.11459183673469414, 0.2719047619047622, -0.08268707482993151, -0.26295918367346893, -0.3956122448979587, -0.16602040816326458, 0.07802721088435427, 0.20897959183673523, 0.1987755102040821, -0.5588775510204076, -0.4415306122448974, -0.4313265306122443, -0.3539455782312919, 0.02615646258503422, 0.049965986394558015, -0.19833333333333314, -0.429625850340136, -0.4951020408163264, -0.7604081632653061, -0.3871088435374147, -0.04357142857142815, -0.1107482993197274, 0.6205442176870752, 0.41306122448979626, 0.39690476190476226, 0.4130612244897964, 0.004897959183673917, 0.018503401360544645, -0.21448979591836695, -0.17707482993197257, -0.22639455782312895, -0.24170068027210861, -0.18047619047619023, -0.3071768707482989, -0.39306122448979547, -0.3037755102040811, -0.34544217687074785, -0.1915306122448977, -0.42877551020408144, -0.48574829931972774, -0.41431972789115623, -0.4049659863945576, -0.038469387755101836, -0.2689115646258501, -0.22554421768707456, -0.44153061224489765, -0.6260544217687071, -0.5971428571428568, -0.7629591836734687, -0.668571428571428, -0.4934013605442171, -0.3071768707482988, -0.27146258503401327, -0.17452380952380908, -0.3173809523809519, -0.4202721088435369, -0.3165306122448976, -0.3046258503401358, -0.17282312925170035, 0.1630612244897961, 0.5584693877551024, 0.4232653061224496, 0.03295918367347006, -0.22299319727891082, -0.6481632653061218, -0.4678911564625847, -0.4253741496598636, -0.44748299319727847, -0.15326530612244862, -0.18982993197278875, 0.0014965986394560662, 0.10013605442176898, 0.01255102040816354, -0.311428571428571, -0.31653061224489754, -0.6524149659863938, -0.7238435374149653, -0.41346938775510145, -0.5019047619047612, -0.33098639455782264, -0.35819727891156417, -0.31312925170067984, -0.1583673469387753, -0.029115646258503214, 0.06952380952380978, 0.15200680272108869, 0.13329931972789147, -0.1889795918367343, -0.5546258503401358, -0.7374489795918364, -0.807176870748299, -0.605646258503401, -0.2791156462585031, -0.20768707482993168, -0.2519047619047616, -0.05122448979591811, -0.07928571428571408, -0.036768707482992935, 0.061020408163265545, 0.004897959183673729, 0.007448979591836969, 0.09758503401360566, -0.0027551020408161236, 0.006598639455782519, -0.06482993197278891, -0.2553061224489794, 0.04231292517006835, -0.2740136054421763, -0.19493197278911506, -0.3522448979591829, -0.5758843537414958, -0.41857142857142815, -0.559727891156462, -0.426224489795918, -0.5376190476190472, -0.19833333333333292, -0.21619047619047585, -0.27401360544217646, 0.18091836734693925, 0.043163265306122814, 0.13755102040816358, 0.35863945578231315, 0.013401360544217908, 0.1128911564625853, 0.29401360544217714, 0.2429931972789118, 0.05421768707483021, -0.17792517006802702, -0.25955782312925146, -0.13030612244897943, 0.04316326530612268, 0.13840136054421792, 0.23619047619047645, 0.2540476190476194, 0.5176530612244902, 0.3356802721088439, 0.31527210884353774, 0.10778911564625877, -0.1447619047619045, -0.18472789115646232, -0.38880952380952355, -0.27316326530612217, -0.4449319727891152, -0.24850340136054372, -0.40666666666666595, -0.477244897959183, -0.12860544217687025, -0.13795918367346888, 0.12734693877551048, 0.2668027210884356, -0.012108843537414676, 0.07632653061224504, 0.00404761904761923, 0.05336734693877569, 0.39180272108843556, 0.12479591836734724, 0.24299319727891186, 0.2336394557823132, 0.06527210884353764, 0.17411564625850368, -0.015510204081632326, -0.1192517006802718, 0.04571428571428621, -0.10479591836734652, -0.29442176870748227, -0.3590476190476183, -0.718741496598639, -0.5843877551020402, -0.1115986394557821, -0.2527551020408161, -0.16942176870748266, -0.2195918367346935, -0.3471428571428568, -0.17367346938775474, 0.11119047619047648, 0.19197278911564652, 0.16306122448979615, -0.17792517006802688, -0.3445918367346935, -0.1915306122448976, -0.37180272108843504, -0.04867346938775487, -0.17282312925170043, -0.432176870748299, -0.2825170068027208, 0.004047619047619411, 0.28465986394557863, 0.2293877551020412, 0.2770068027210889, 0.01510204081632684, -0.03421768707482964, 0.17496598639455813, -0.03591836734693843, -0.18132653061224452, -0.10309523809523774, 0.024455782312925528, 0.09163265306122476, 0.01935374149659891, 0.07887755102040847, 0.25489795918367425, 0.5142517006802729, 0.6350000000000009, 0.3526870748299327, -0.07758503401360516, -0.5214625850340133, -0.5860884353741493]
  out "CH 0 Bin Readings":dbl[](array[numeric])=[131.0, 107.0, 101.0, 98.0, 99.0, 71.0, 90.0, 87.0, 89.0, 85.0, 115.0, 106.0, 102.0, 104.0, 113.0, 94.0, 120.0, 126.0, 128.0, 138.0, 139.0, 131.0, 149.0, 142.0, 163.0, 142.0, 170.0, 154.0, 152.0, 170.0, 180.0, 173.0, 145.0, 164.0, 158.0, 129.0, 171.0, 131.0, 164.0, 162.0, 136.0, 132.0, 128.0, 147.0, 142.0, 155.0, 128.0, 125.0, 138.0, 131.0, 111.0, 125.0, 113.0, 112.0, 112.0, 127.0, 118.0, 119.0, 92.0, 99.0, 110.0, 107.0, 90.0, 92.0, 101.0, 84.0, 96.0, 99.0, 100.0, 69.0, 87.0, 74.0, 79.0, 77.0, 93.0, 84.0, 83.0, 86.0, 93.0, 80.0, 66.0, 70.0, 81.0, 58.0, 69.0, 78.0, 78.0, 88.0, 95.0, 93.0, 104.0, 97.0, 98.0, 98.0, 103.0, 111.0, 124.0, 199.0, 268.0, 398.0, 432.0, 426.0, 418.0, 289.0, 164.0, 87.0, 65.0, 64.0, 55.0, 67.0, 66.0, 58.0, 75.0, 79.0, 66.0, 65.0, 55.0, 76.0, 60.0, 68.0, 67.0, 58.0, 37.0, 55.0, 72.0, 51.0, 59.0, 60.0, 66.0, 55.0, 51.0, 52.0, 68.0, 73.0, 57.0, 66.0, 81.0, 90.0, 103.0, 140.0, 144.0, 172.0, 195.0, 175.0, 169.0, 175.0, 131.0, 100.0, 134.0, 103.0, 129.0, 123.0, 142.0, 154.0, 167.0, 165.0, 198.0, 220.0, 223.0, 216.0, 187.0, 180.0, 171.0, 156.0, 150.0, 139.0, 150.0, 139.0, 134.0, 124.0, 112.0, 125.0, 133.0, 116.0, 125.0, 126.0, 151.0, 167.0, 189.0, 163.0, 153.0, 140.0, 120.0, 113.0, 98.0, 106.0, 124.0, 117.0, 99.0, 88.0, 112.0, 104.0, 104.0, 102.0, 91.0, 87.0, 90.0, 89.0, 92.0, 93.0, 62.0, 78.0, 71.0, 75.0, 82.0, 78.0, 73.0, 84.0, 83.0, 89.0, 92.0, 109.0, 85.0, 90.0, 61.0, 55.0, 53.0, 57.0, 59.0, 74.0, 64.0, 67.0, 77.0, 74.0, 75.0, 61.0, 71.0, 55.0, 50.0, 69.0, 61.0, 59.0, 59.0, 70.0, 66.0, 52.0, 47.0, 59.0, 62.0, 61.0, 56.0, 51.0, 53.0, 57.0, 53.0, 68.0, 61.0, 65.0, 42.0, 56.0, 49.0, 45.0, 52.0, 57.0, 67.0, 63.0, 77.0, 56.0, 48.0, 60.0, 51.0, 55.0, 53.0, 47.0, 58.0, 61.0, 51.0, 56.0, 41.0, 42.0, 48.0, 46.0, 50.0, 52.0, 63.0, 46.0, 57.0, 62.0, 50.0, 57.0, 56.0, 53.0, 49.0, 47.0, 64.0, 65.0, 60.0, 57.0, 43.0, 59.0, 50.0, 44.0, 59.0, 40.0, 47.0, 42.0, 48.0, 67.0, 52.0, 52.0, 53.0, 64.0, 52.0, 53.0, 44.0, 49.0, 50.0, 66.0, 40.0, 54.0, 50.0, 57.0, 70.0, 57.0, 55.0, 43.0, 49.0, 50.0, 62.0, 48.0, 40.0, 57.0, 53.0, 51.0, 49.0, 64.0, 53.0, 66.0, 62.0, 59.0, 39.0, 55.0, 58.0, 47.0, 50.0, 50.0, 50.0, 58.0, 49.0, 39.0, 65.0, 51.0, 50.0, 42.0, 53.0, 51.0, 56.0, 51.0, 56.0, 61.0, 60.0, 58.0, 68.0, 57.0, 32.0, 63.0, 58.0, 62.0, 55.0, 68.0, 59.0, 43.0, 57.0, 61.0, 51.0, 45.0, 49.0, 61.0, 56.0, 52.0, 44.0, 58.0, 55.0, 55.0, 57.0, 47.0, 50.0, 48.0, 45.0, 54.0, 31.0, 51.0, 53.0, 45.0, 51.0, 63.0, 63.0, 53.0, 44.0, 43.0, 53.0, 49.0, 49.0, 50.0, 54.0, 58.0, 59.0, 39.0, 45.0, 45.0, 46.0, 59.0, 59.0, 48.0, 55.0, 49.0, 55.0, 55.0, 43.0, 48.0, 48.0, 49.0, 60.0, 46.0, 65.0, 47.0, 57.0, 59.0, 52.0, 52.0, 74.0, 67.0, 44.0, 60.0, 42.0, 52.0, 43.0, 48.0, 54.0, 45.0, 46.0, 52.0, 54.0, 51.0, 49.0, 50.0, 40.0, 55.0, 50.0, 57.0, 57.0, 54.0, 60.0, 50.0, 64.0, 62.0, 46.0, 42.0, 56.0, 58.0, 52.0, 42.0, 42.0, 51.0, 44.0, 63.0, 57.0, 61.0, 66.0, 46.0, 58.0, 54.0, 54.0, 53.0, 68.0, 60.0, 57.0, 57.0, 60.0, 49.0, 41.0, 50.0, 46.0, 52.0, 56.0, 55.0, 54.0, 51.0, 50.0, 44.0, 51.0, 57.0, 57.0, 53.0, 54.0, 55.0, 51.0, 52.0, 49.0, 52.0, 56.0, 52.0, 59.0, 58.0, 47.0, 55.0, 50.0, 42.0, 44.0, 48.0, 60.0, 53.0, 53.0, 71.0, 55.0, 43.0, 61.0, 61.0, 42.0, 59.0, 40.0, 45.0, 57.0, 53.0, 64.0, 53.0, 53.0, 67.0, 52.0, 54.0, 47.0, 56.0, 52.0, 58.0, 64.0, 46.0, 44.0, 52.0, 49.0, 64.0, 57.0, 58.0, 55.0, 54.0, 45.0, 45.0, 45.0, 57.0, 47.0, 47.0, 56.0, 52.0, 58.0, 60.0, 57.0, 60.0, 56.0, 44.0, 56.0, 50.0, 59.0, 47.0, 47.0, 32.0, 56.0, 64.0, 45.0, 56.0, 64.0]
  out "Range Corrected Altitude Array":dbl[](array[numeric])=[1406.25, 5625.0, 12656.25, 22500.0, 35156.25, 50625.0, 68906.25, 90000.0, 113906.25, 140625.0, 170156.25, 202500.0, 237656.25, 275625.0, 316406.25, 360000.0, 406406.25, 455625.0, 507656.25, 562500.0, 620156.25, 680625.0, 743906.25, 810000.0, 878906.25, 950625.0, 1025156.25, 1102500.0, 1182656.25, 1265625.0, 1351406.25, 1440000.0, 1531406.25, 1625625.0, 1722656.25, 1822500.0, 1925156.25, 2030625.0, 2138906.25, 2250000.0, 2363906.25, 2480625.0, 2600156.25, 2722500.0, 2847656.25, 2975625.0, 3106406.25, 3240000.0, 3376406.25, 3515625.0, 3657656.25, 3802500.0, 3950156.25, 4100625.0, 4253906.25, 4410000.0, 4568906.25, 4730625.0, 4895156.25, 5062500.0, 5232656.25, 5405625.0, 5581406.25, 5760000.0, 5941406.25, 6125625.0, 6312656.25, 6502500.0, 6695156.25, 6890625.0, 7088906.25, 7290000.0, 7493906.25, 7700625.0, 7910156.25, 8122500.0, 8337656.25, 8555625.0, 8776406.25, 9000000.0, 9226406.25, 9455625.0, 9687656.25, 9922500.0, 10160156.25, 10400625.0, 10643906.25, 10890000.0, 11138906.25, 11390625.0, 11645156.25, 11902500.0, 12162656.25, 12425625.0, 12691406.25, 12960000.0, 13231406.25, 13505625.0, 13782656.25, 14062500.0, 14345156.25, 14630625.0, 14918906.25, 15210000.0, 15503906.25, 15800625.0, 16100156.25, 16402500.0, 16707656.25, 17015625.0, 17326406.25, 17640000.0, 17956406.25, 18275625.0, 18597656.25, 18922500.0, 19250156.25, 19580625.0, 19913906.25, 20250000.0, 20588906.25, 20930625.0, 21275156.25, 21622500.0, 21972656.25, 22325625.0, 22681406.25, 23040000.0, 23401406.25, 23765625.0, 24132656.25, 24502500.0, 24875156.25, 25250625.0, 25628906.25, 26010000.0, 26393906.25, 26780625.0, 27170156.25, 27562500.0, 27957656.25, 28355625.0, 28756406.25, 29160000.0, 29566406.25, 29975625.0, 30387656.25, 30802500.0, 31220156.25, 31640625.0, 32063906.25, 32490000.0, 32918906.25, 33350625.0, 33785156.25, 34222500.0, 34662656.25, 35105625.0, 35551406.25, 36000000.0, 36451406.25, 36905625.0, 37362656.25, 37822500.0, 38285156.25, 38750625.0, 39218906.25, 39690000.0, 40163906.25, 40640625.0, 41120156.25, 41602500.0, 42087656.25, 42575625.0, 43066406.25, 43560000.0, 44056406.25, 44555625.0, 45057656.25, 45562500.0, 46070156.25, 46580625.0, 47093906.25, 47610000.0, 48128906.25, 48650625.0, 49175156.25, 49702500.0, 50232656.25, 50765625.0, 51301406.25, 51840000.0, 52381406.25, 52925625.0, 53472656.25, 54022500.0, 54575156.25, 55130625.0, 55688906.25, 56250000.0, 56813906.25, 57380625.0, 57950156.25, 58522500.0, 59097656.25, 59675625.0, 60256406.25, 60840000.0, 61426406.25, 62015625.0, 62607656.25, 63202500.0, 63800156.25, 64400625.0, 65003906.25, 65610000.0, 66218906.25, 66830625.0, 67445156.25, 68062500.0, 68682656.25, 69305625.0, 69931406.25, 70560000.0, 71191406.25, 71825625.0, 72462656.25, 73102500.0, 73745156.25, 74390625.0, 75038906.25, 75690000.0, 76343906.25, 77000625.0, 77660156.25, 78322500.0, 78987656.25, 79655625.0, 80326406.25, 81000000.0, 81676406.25, 82355625.0, 83037656.25, 83722500.0, 84410156.25, 85100625.0, 85793906.25, 86490000.0, 87188906.25, 87890625.0, 88595156.25, 89302500.0, 90012656.25, 90725625.0, 91441406.25, 92160000.0, 92881406.25, 93605625.0, 94332656.25, 95062500.0, 95795156.25, 96530625.0, 97268906.25, 98010000.0, 98753906.25, 99500625.0, 100250156.25, 101002500.0, 101757656.25, 102515625.0, 103276406.25, 104040000.0, 104806406.25, 105575625.0, 106347656.25, 107122500.0, 107900156.25, 108680625.0, 109463906.25, 110250000.0, 111038906.25, 111830625.0, 112625156.25, 113422500.0, 114222656.25, 115025625.0, 115831406.25, 116640000.0, 117451406.25, 118265625.0, 119082656.25, 119902500.0, 120725156.25, 121550625.0, 122378906.25, 123210000.0, 124043906.25, 124880625.0, 125720156.25, 126562500.0, 127407656.25, 128255625.0, 129106406.25, 129960000.0, 130816406.25, 131675625.0, 132537656.25, 133402500.0, 134270156.25, 135140625.0, 136013906.25, 136890000.0, 137768906.25, 138650625.0, 139535156.25, 140422500.0, 141312656.25, 142205625.0, 143101406.25, 144000000.0, 144901406.25, 145805625.0, 146712656.25, 147622500.0, 148535156.25, 149450625.0, 150368906.25, 151290000.0, 152213906.25, 153140625.0, 154070156.25, 155002500.0, 155937656.25, 156875625.0, 157816406.25, 158760000.0, 159706406.25, 160655625.0, 161607656.25, 162562500.0, 163520156.25, 164480625.0, 165443906.25, 166410000.0, 167378906.25, 168350625.0, 169325156.25, 170302500.0, 171282656.25, 172265625.0, 173251406.25, 174240000.0, 175231406.25, 176225625.0, 177222656.25, 178222500.0, 179225156.25, 180230625.0, 181238906.25, 182250000.0, 183263906.25, 184280625.0, 185300156.25, 186322500.0, 187347656.25, 188375625.0, 189406406.25, 190440000.0, 191476406.25, 192515625.0, 193557656.25, 194602500.0, 195650156.25, 196700625.0, 197753906.25, 198810000.0, 199868906.25, 200930625.0, 201995156.25, 203062500.0, 204132656.25, 205205625.0, 206281406.25, 207360000.0, 208441406.25, 209525625.0, 210612656.25, 211702500.0, 212795156.25, 213890625.0, 214988906.25, 216090000.0, 217193906.25, 218300625.0, 219410156.25, 220522500.0, 221637656.25, 222755625.0, 223876406.25, 225000000.0, 226126406.25, 227255625.0, 228387656.25, 229522500.0, 230660156.25, 231800625.0, 232943906.25, 234090000.0, 235238906.25, 236390625.0, 237545156.25, 238702500.0, 239862656.25, 241025625.0, 242191406.25, 243360000.0, 244531406.25, 245705625.0, 246882656.25, 248062500.0, 249245156.25, 250430625.0, 251618906.25, 252810000.0, 254003906.25, 255200625.0, 256400156.25, 257602500.0, 258807656.25, 260015625.0, 261226406.25, 262440000.0, 263656406.25, 264875625.0, 266097656.25, 267322500.0, 268550156.25, 269780625.0, 271013906.25, 272250000.0, 273488906.25, 274730625.0, 275975156.25, 277222500.0, 278472656.25, 279725625.0, 280981406.25, 282240000.0, 283501406.25, 284765625.0, 286032656.25, 287302500.0, 288575156.25, 289850625.0, 291128906.25, 292410000.0, 293693906.25, 294980625.0, 296270156.25, 297562500.0, 298857656.25, 300155625.0, 301456406.25, 302760000.0, 304066406.25, 305375625.0, 306687656.25, 308002500.0, 309320156.25, 310640625.0, 311963906.25, 313290000.0, 314618906.25, 315950625.0, 317285156.25, 318622500.0, 319962656.25, 321305625.0, 322651406.25, 324000000.0, 325351406.25, 326705625.0, 328062656.25, 329422500.0, 330785156.25, 332150625.0, 333518906.25, 334890000.0, 336263906.25, 337640625.0, 339020156.25, 340402500.0, 341787656.25, 343175625.0, 344566406.25, 345960000.0, 347356406.25, 348755625.0, 350157656.25, 351562500.0, 352970156.25, 354380625.0, 355793906.25, 357210000.0, 358628906.25, 360050625.0, 361475156.25, 362902500.0, 364332656.25, 365765625.0, 367201406.25, 368640000.0, 370081406.25, 371525625.0, 372972656.25, 374422500.0, 375875156.25, 377330625.0, 378788906.25, 380250000.0, 381713906.25, 383180625.0, 384650156.25, 386122500.0, 387597656.25, 389075625.0, 390556406.25, 392040000.0, 393526406.25, 395015625.0, 396507656.25, 398002500.0, 399500156.25, 401000625.0, 402503906.25, 404010000.0, 405518906.25, 407030625.0, 408545156.25, 410062500.0, 411582656.25, 413105625.0, 414631406.25, 416160000.0, 417691406.25, 419225625.0, 420762656.25, 422302500.0, 423845156.25, 425390625.0, 426938906.25, 428490000.0, 430043906.25, 431600625.0, 433160156.25, 434722500.0, 436287656.25, 437855625.0, 439426406.25, 441000000.0]
  out "Altitude Array (km)":dbl[](array[numeric])=[0.0375, 0.075, 0.11249999999999999, 0.15, 0.1875, 0.225, 0.26249999999999996, 0.3, 0.33749999999999997, 0.37499999999999994, 0.4125, 0.44999999999999996, 0.48749999999999993, 0.525, 0.5625, 0.6, 0.6375, 0.6749999999999999, 0.7124999999999999, 0.75, 0.7875, 0.825, 0.8624999999999999, 0.8999999999999999, 0.9374999999999999, 0.975, 1.0125, 1.05, 1.0875000000000001, 1.125, 1.1625, 1.2, 1.2375, 1.2750000000000001, 1.3125, 1.35, 1.3875, 1.425, 1.4625000000000001, 1.5, 1.5375, 1.575, 1.6125, 1.6500000000000001, 1.6875, 1.725, 1.7625, 1.8, 1.8375, 1.875, 1.9125, 1.95, 1.9875, 2.025, 2.0625, 2.1, 2.1375, 2.175, 2.2125, 2.25, 2.2875, 2.325, 2.3625, 2.4, 2.4375, 2.475, 2.5125, 2.55, 2.5875, 2.625, 2.6625, 2.7, 2.7375, 2.775, 2.8125, 2.85, 2.8875, 2.925, 2.9625, 3.0, 3.0375, 3.075, 3.1125, 3.15, 3.1875, 3.225, 3.2625, 3.3, 3.3375, 3.375, 3.4125, 3.45, 3.4875, 3.525, 3.5625, 3.6, 3.6374999999999997, 3.675, 3.7125, 3.75, 3.7875, 3.8249999999999997, 3.8625, 3.9, 3.9375, 3.975, 4.012499999999999, 4.05, 4.0874999999999995, 4.124999999999999, 4.1625, 4.199999999999999, 4.2375, 4.2749999999999995, 4.312499999999999, 4.35, 4.387499999999999, 4.425, 4.4624999999999995, 4.499999999999999, 4.5375, 4.574999999999999, 4.6125, 4.6499999999999995, 4.687499999999999, 4.725, 4.762499999999999, 4.8, 4.8374999999999995, 4.874999999999999, 4.9125, 4.949999999999999, 4.9875, 5.0249999999999995, 5.062499999999999, 5.1, 5.137499999999999, 5.175, 5.2124999999999995, 5.249999999999999, 5.2875, 5.324999999999999, 5.3625, 5.3999999999999995, 5.437499999999999, 5.475, 5.512499999999999, 5.55, 5.5874999999999995, 5.624999999999999, 5.6625, 5.699999999999999, 5.7375, 5.7749999999999995, 5.812499999999999, 5.85, 5.887499999999999, 5.925, 5.9624999999999995, 5.999999999999999, 6.0375, 6.074999999999999, 6.1125, 6.1499999999999995, 6.187499999999999, 6.225, 6.262499999999999, 6.3, 6.3374999999999995, 6.374999999999999, 6.4125, 6.449999999999999, 6.4875, 6.5249999999999995, 6.562499999999999, 6.6, 6.637499999999999, 6.675, 6.7124999999999995, 6.749999999999999, 6.7875, 6.824999999999999, 6.8625, 6.8999999999999995, 6.937499999999999, 6.975, 7.012499999999999, 7.05, 7.0874999999999995, 7.124999999999999, 7.1625, 7.199999999999999, 7.237499999999999, 7.2749999999999995, 7.312499999999999, 7.35, 7.387499999999999, 7.424999999999999, 7.4624999999999995, 7.499999999999999, 7.5375, 7.574999999999999, 7.612499999999999, 7.6499999999999995, 7.687499999999999, 7.725, 7.762499999999999, 7.799999999999999, 7.8374999999999995, 7.874999999999999, 7.9125, 7.949999999999999, 7.987499999999999, 8.025, 8.0625, 8.1, 8.1375, 8.174999999999999, 8.212499999999999, 8.25, 8.2875, 8.325, 8.362499999999999, 8.399999999999999, 8.4375, 8.475, 8.5125, 8.549999999999999, 8.587499999999999, 8.625, 8.6625, 8.7, 8.737499999999999, 8.774999999999999, 8.8125, 8.85, 8.8875, 8.924999999999999, 8.962499999999999, 9.0, 9.0375, 9.075, 9.112499999999999, 9.149999999999999, 9.1875, 9.225, 9.2625, 9.299999999999999, 9.337499999999999, 9.375, 9.4125, 9.45, 9.487499999999999, 9.524999999999999, 9.5625, 9.6, 9.6375, 9.674999999999999, 9.712499999999999, 9.75, 9.7875, 9.825, 9.862499999999999, 9.899999999999999, 9.9375, 9.975, 10.0125, 10.049999999999999, 10.087499999999999, 10.125, 10.1625, 10.2, 10.237499999999999, 10.274999999999999, 10.3125, 10.35, 10.3875, 10.424999999999999, 10.462499999999999, 10.5, 10.5375, 10.575, 10.612499999999999, 10.649999999999999, 10.6875, 10.725, 10.7625, 10.799999999999999, 10.837499999999999, 10.875, 10.9125, 10.95, 10.987499999999999, 11.024999999999999, 11.0625, 11.1, 11.1375, 11.174999999999999, 11.212499999999999, 11.25, 11.2875, 11.325, 11.362499999999999, 11.399999999999999, 11.4375, 11.475, 11.5125, 11.549999999999999, 11.587499999999999, 11.625, 11.6625, 11.7, 11.737499999999999, 11.774999999999999, 11.8125, 11.85, 11.8875, 11.924999999999999, 11.962499999999999, 12.0, 12.0375, 12.075, 12.112499999999999, 12.149999999999999, 12.1875, 12.225, 12.2625, 12.299999999999999, 12.337499999999999, 12.375, 12.4125, 12.45, 12.487499999999999, 12.524999999999999, 12.5625, 12.6, 12.6375, 12.674999999999999, 12.712499999999999, 12.75, 12.7875, 12.825, 12.862499999999999, 12.899999999999999, 12.9375, 12.975, 13.0125, 13.049999999999999, 13.087499999999999, 13.125, 13.1625, 13.2, 13.237499999999999, 13.274999999999999, 13.3125, 13.35, 13.3875, 13.424999999999999, 13.462499999999999, 13.5, 13.5375, 13.575, 13.612499999999999, 13.649999999999999, 13.6875, 13.725, 13.7625, 13.799999999999999, 13.837499999999999, 13.875, 13.9125, 13.95, 13.987499999999999, 14.024999999999999, 14.0625, 14.1, 14.1375, 14.174999999999999, 14.212499999999999, 14.25, 14.2875, 14.325, 14.362499999999999, 14.399999999999999, 14.437499999999998, 14.475, 14.5125, 14.549999999999999, 14.587499999999999, 14.624999999999998, 14.6625, 14.7, 14.737499999999999, 14.774999999999999, 14.812499999999998, 14.85, 14.8875, 14.924999999999999, 14.962499999999999, 14.999999999999998, 15.0375, 15.075, 15.112499999999999, 15.149999999999999, 15.187499999999998, 15.225, 15.2625, 15.299999999999999, 15.337499999999999, 15.374999999999998, 15.4125, 15.45, 15.487499999999999, 15.524999999999999, 15.562499999999998, 15.6, 15.6375, 15.674999999999999, 15.712499999999999, 15.749999999999998, 15.7875, 15.825, 15.862499999999999, 15.899999999999999, 15.937499999999998, 15.975, 16.0125, 16.05, 16.087500000000002, 16.125, 16.1625, 16.2, 16.2375, 16.275000000000002, 16.3125, 16.35, 16.3875, 16.425, 16.462500000000002, 16.5, 16.5375, 16.575, 16.6125, 16.650000000000002, 16.6875, 16.725, 16.7625, 16.8, 16.837500000000002, 16.875, 16.9125, 16.95, 16.9875, 17.025000000000002, 17.0625, 17.1, 17.1375, 17.175, 17.212500000000002, 17.25, 17.2875, 17.325, 17.3625, 17.400000000000002, 17.4375, 17.475, 17.5125, 17.55, 17.587500000000002, 17.625, 17.6625, 17.7, 17.7375, 17.775000000000002, 17.8125, 17.85, 17.8875, 17.925, 17.962500000000002, 18.0, 18.0375, 18.075, 18.1125, 18.150000000000002, 18.1875, 18.225, 18.2625, 18.3, 18.337500000000002, 18.375, 18.4125, 18.45, 18.4875, 18.525000000000002, 18.5625, 18.6, 18.6375, 18.675, 18.712500000000002, 18.75, 18.7875, 18.825, 18.8625, 18.900000000000002, 18.9375, 18.975, 19.0125, 19.05, 19.087500000000002, 19.125, 19.1625, 19.2, 19.2375, 19.275000000000002, 19.3125, 19.35, 19.3875, 19.425, 19.462500000000002, 19.5, 19.5375, 19.575, 19.6125, 19.650000000000002, 19.6875, 19.725, 19.7625, 19.8, 19.837500000000002, 19.875, 19.9125, 19.95, 19.9875, 20.025000000000002, 20.0625, 20.1, 20.1375, 20.175, 20.212500000000002, 20.25, 20.2875, 20.325, 20.3625, 20.400000000000002, 20.4375, 20.475, 20.5125, 20.55, 20.587500000000002, 20.625, 20.6625, 20.7, 20.7375, 20.775000000000002, 20.8125, 20.85, 20.8875, 20.925, 20.962500000000002, 21.0]
  out "Offline Pulse Energy":dbl=5.135677142857142
  out "Online Pulse Energy":dbl=5.135471428571428
  in  "Instrument Control":T5(tab)=enum."DAQ"
  in  "Device In":refnum<visa-resource-name>="GPIB0::10::INSTR"
  in  "Settings":T6={"Module"=enum."WV Online TEC", "WV Online TEC"=23.18950000000041, "WV Online LD"=0.175, "WV Offline TEC"=29.64900000000008, "WV Offline LD"=0.17, "WV Etalon TEC"=28.0, "HSRL Etalon TEC"=25.954, "HSRL TEC"=14.379749999999587, "HSRL LD"=0.16} {"HSRL LD" min=0.0 max=0.18 step=0.001 format="%.3p"; "HSRL TEC" min=14.0 max=28.0 step=0.1 format="%.3g"; "WV Offline LD" min=0.0 max=0.18 step=0.001 format="%.3p"; "WV Online LD" min=0.0 max=0.18 step=0.001 format="%.3p"; "HSRL Etalon TEC" format="%.2g"; "WV Etalon TEC" format="%.2g"; "WV Offline TEC" min=16.0 max=30.0 step=0.1 format="%.3g"; "WV Online TEC" min=14.0 max=28.0 step=0.1 format="%.3g"}
  out "Readings":T7={"Pro8000"=TRUE, "WV OnLine TEC"=23.194788, "WV Online TEC"=TRUE, "WV Online LD"=0.175152346, "WV Online LD"=TRUE, "WV Offline TEC"=29.6612492, "WV Offline TEC"=TRUE, "WV Offline LD"=0.17038478, "WV Offline LD"=TRUE, "WV EtalonTEC"=28.0131836, "WV Etalon TEC"=TRUE, "HSRL Etalon TEC"=25.9483566, "HSRL Etalon TEC"=TRUE, "HSRL TEC"=14.3906193, "HSRL TEC "=TRUE, "HSRL LD"=0.160277352, "HSRL LD"=TRUE} {"HSRL LD" format="%.3p"; "HSRL TEC" format="%.3g"; "WV Offline LD" format="%.3p"; "WV Online LD" format="%.3p"; "HSRL Etalon TEC" format="%.3g"; "WV EtalonTEC" format="%.3g"; "WV Offline TEC" format="%.3g"; "WV OnLine TEC" format="%.3g"}
  in  "Pulse B Polarity":enum32{"Low", "High"}(ring)=enum."High"
  in  "Pulse A Delay(ns)":u32=1040 min=80 max=327600
  in  "Pulse B Delay(ns)":u32=170000 min=80 max=327600 step=1
  in  "Accumulation Delay(ns)":u32=10 min=10 max=1270 step=1
  in  "Sync Pulse Polarity":enum32{"Low", "High"}(ring)=enum."High"
  in  "Pulse A Polarity":enum32{"Low", "High"}(ring)=enum."High"
  in  "Number of Bins":u32=560 min=2 max=4095 step=1
  in  "Number of Accumulates":u32=14285 min=1 max=32767 step=1
  in  "Time Resolution Per Bin(ns)":u32=250 min=5 max=1063 step=1
  out "AMCS_Profile":i32=6664
  in  "WV Online Set (nm)":dbl=828.198 format="%.5f"
  out "WV Online Read (nm)":dbl=828.1980354483289 format="%.5f"
  out "WV Offline Read (nm)":dbl=828.2976456580193 format="%.5f"
  in  "WV Offline Set (nm)":dbl=828.29765 format="%.5f"
  in  "Bristol In":i32=5
  out "Bristol Out":i32
  out "Online_Diff":dbl=3.544832895840955e-05 format="%#_3e"
  out "Oflline_Diff":dbl=-4.341980684330338e-06 format="%#_3e"
  out "WV Online Locked":bool=TRUE
  out "WV Oflline Locked":bool=TRUE
  in  "calculate absorption cross sections":bool
  in  "Online_Tol":dbl=7.5e-05 format="%#_15g"
  in  "Cancel online":bool
  in  "Offline_Tol":dbl=7.5e-05 format="%#_15g"
  in  "Cancel Offline":bool
  in  "temp step size":dbl=0.00025 format="%#_6p"
  in  "HSRL_Tol":dbl=7.5e-05 format="%#_15g"
  out "HSRL_Diff":dbl=-1.842011624830775e-05 format="%#_3e"
  in  "Cancel HSRL":bool
  out "HSRL Locked":bool=TRUE
  out "HSRL Read (nm)":dbl=780.2461015798838 format="%.5f"
  in  "HSRL Set (nm)":dbl=780.24612 format="%#.5f"
  in  "Smoothing Range":dbl=150.0
  in  "Total DIAL Integration Time (Minutes)":i32=4
  in  "Data Reads (number of loops)":i32=1
  in  "Total Aerosol Integration Time (Minutes)":dbl=0.5
  in  "Scalar Wait Time":u32
  out "Smoothed Bins":dbl=4.0
  out "gate size":dbl
  in  "NewportIn":string
  in  "logging":bool
  out "Newport Device Key":string="1918-R 15120"
  in  "SampleSize":i32=2
  out "NewportRef":refnum<k24>
  in  "Switch Comm Port":refnum<visa-resource-name>="COM3"
  out "FF_On_Ref":refnum<file>
  out "FF_On_Ptr":i64=1734224 format="%.2p"
  out "FF_Off_Ref":refnum<file>
  out "FF_Off_Ptr":i64=1734224 format="%.2p"
  out "NF_On_Ref":refnum<file>
  out "NF_On_Ptr":i64=1734224 format="%.2p"
  out "NF_Off_Ref":refnum<file>
  out "NF_Off_Ptr":i64=1734224 format="%.2p"
  out "DataOpen":bool=TRUE
  out "File Path_Far Field (out)":string="C:\\Users\\H2ODial\\Desktop\\SharedTeleWVData\\170510FF\\01"
  out "File Path_Near Field (out)":string="C:\\Users\\H2ODial\\Desktop\\SharedTeleWVData\\170510NF\\01"
  in  "Data File DIR (in)":string="C:\\Users\\H2ODial\\Desktop\\SharedTeleWVData\\"
  out "TRHP":T8={"Temp C"=16.945207570207558, "RelH %"=59.93894993894994, "Press hPa"=832.1978021978022, "AbH g/m^3"=8.653846153846155}
  in  "WS visa":refnum<visa-resource-name>="COM6"
  in  "WS_On/Off":bool=TRUE
  in  "bins":u32=560 min=2 max=4095 step=1
  out "y offset":u32=10
  in  "ns scale":u32=250
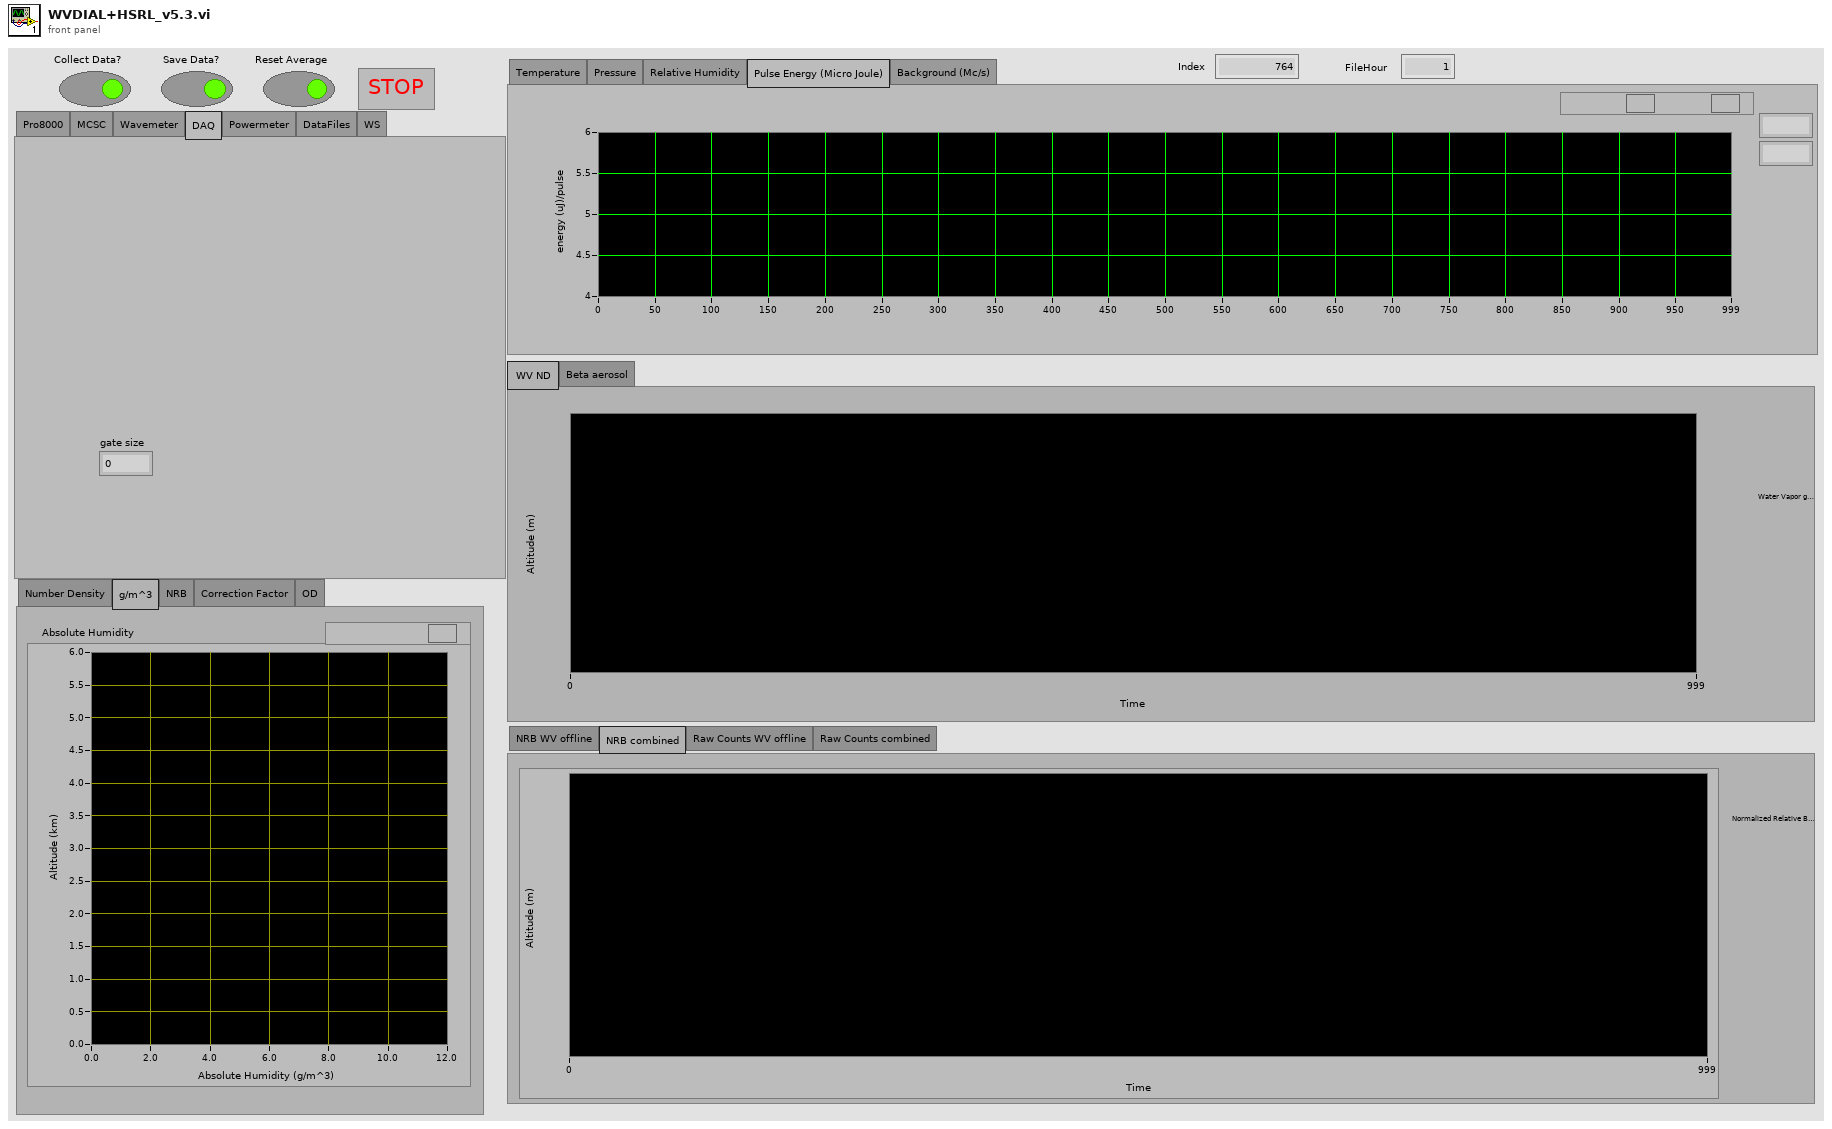
[diagram p1: front panel]
types:
  T1 = enum32{"NRB WV offline", "NRB combined", "Raw Counts WV offline", "Raw Counts combined"}
  T2 = enum32{"Number Density", "g/m^3", "NRB", "Correction Factor", "OD"}
  T3 = enum32{"Temperature", "Pressure", "Relative Humidity", "Pulse Energy (Micro Joule)", "Background (Mc/s)"}
  T4 = cluster{"Online Pulse Energy":dbl, "Pulse Energy Offline":dbl}
  T5 = enum32{"Pro8000", "MCSC", "Wavemeter", "DAQ", "Powermeter", "DataFiles", "WS"}
  T6 = cluster{"Module":enum16{"WV Online TEC", "WV Online LD", "WV Offline TEC", "WV Offline LD", "WV Etalon TEC", "HSRL Etalon TEC", "HSRL TEC", "HSRL LD"}, "WV Online TEC":dbl, "WV Online LD":dbl, "WV Offline TEC":dbl, "WV Offline LD":dbl, "WV Etalon TEC":dbl, "HSRL Etalon TEC":dbl, "HSRL TEC":dbl, "HSRL LD":dbl}
  T7 = cluster{"Pro8000":bool, "WV OnLine TEC":dbl, "WV Online TEC":bool, "WV Online LD":dbl, "WV Online LD":bool, "WV Offline TEC":dbl, "WV Offline TEC":bool, "WV Offline LD":dbl, "WV Offline LD":bool, "WV EtalonTEC":dbl, "WV Etalon TEC":bool, "HSRL Etalon TEC":dbl, "HSRL Etalon TEC":bool, "HSRL TEC":dbl, "HSRL TEC ":bool, "HSRL LD":dbl, "HSRL LD":bool}
  T8 = cluster{"Temp C":dbl, "RelH %":dbl, "Press hPa":dbl, "AbH g/m^3":dbl}
  T9 = enum16{"Open_TL", "Close_TL", "Verify_ID", "TEC_Sensor", "SET", "READ", "ON", "OFF", "Set_Limits", "Read_Limits", "Enable_Status", "Read_Status"}
  T10 = enum16{"Initialize ILX", "Set ON T", "Set Off T", "Set ON I", "Set Off I", "Set On Lim", "Set Off Lim", "Read ILX", "TEC ON/OFF", "LASER ON/OFF", "Status?", "ILX OFF"}
  T11 = enum16{"open", "replace", "create", "open or create", "replace or create", "replace or create with confirmation"}
  T12 = enum16{"WV Online TEC", "WV Online LD", "WV Offline TEC", "WV Offline LD", "WV Etalon TEC", "HSRL Etalon TEC", "HSRL TEC", "HSRL LD"}
  T13 = cluster{"Temp":dbl, "RelH":dbl, "Press":dbl, "AbH":dbl}
  T14 = typedef "LVDateTimeRec.ctl" = cluster{"fractional second":dbl, "second":i32, "minute":i32, "hour":i32, "day of month":i32, "month":i32, "year":i32, "day of week":i32, "day of year":i32, "DST":i32}
  T15 = cluster{"Online Pulse Energy":dbl, "Offline Pulse Energy":dbl}
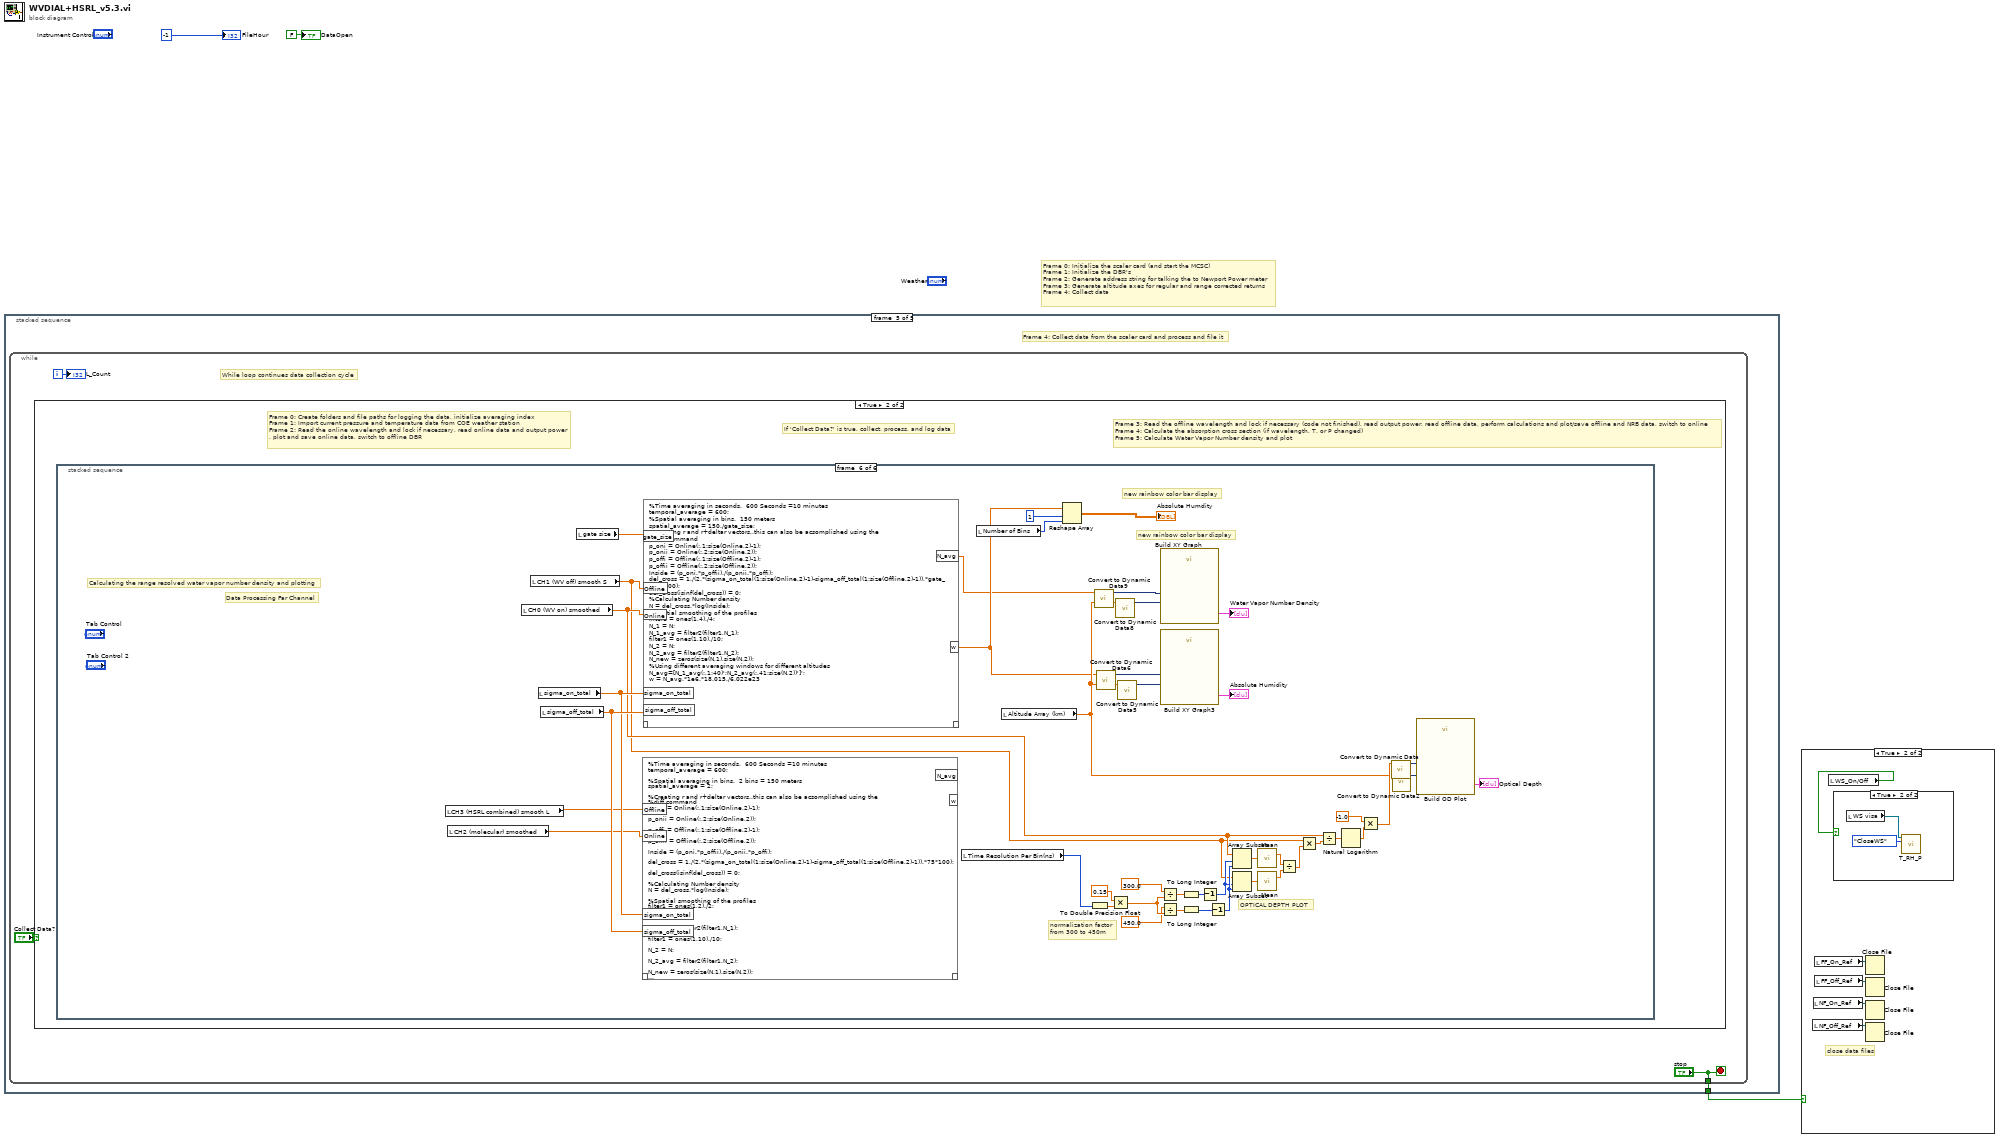
[diagram p0: block diagram]
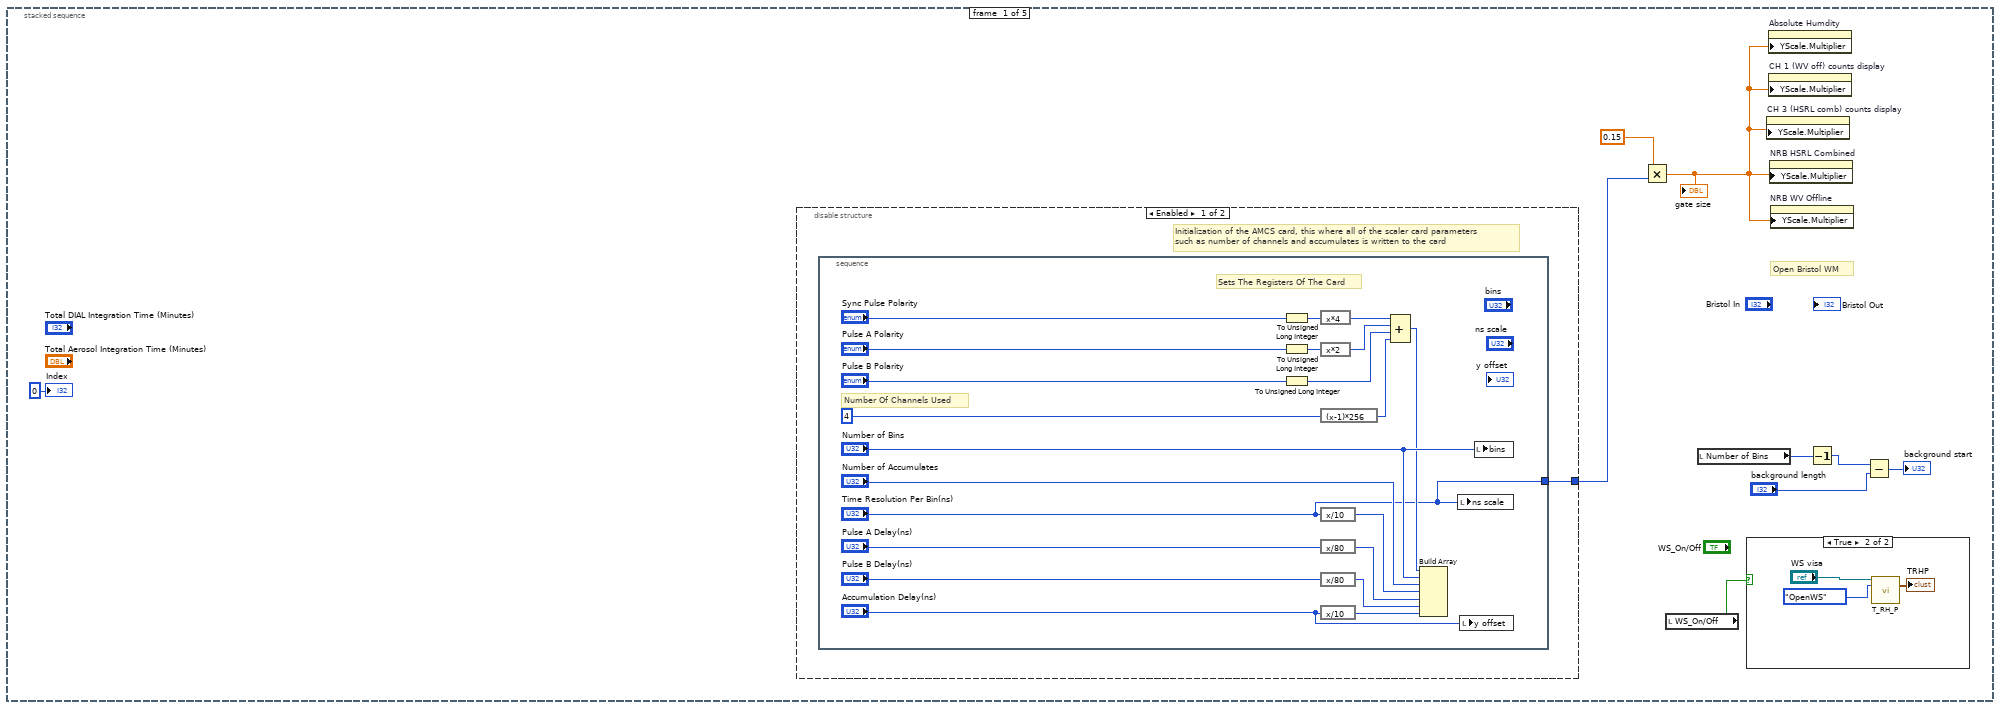
[diagram p4: hidden frame]
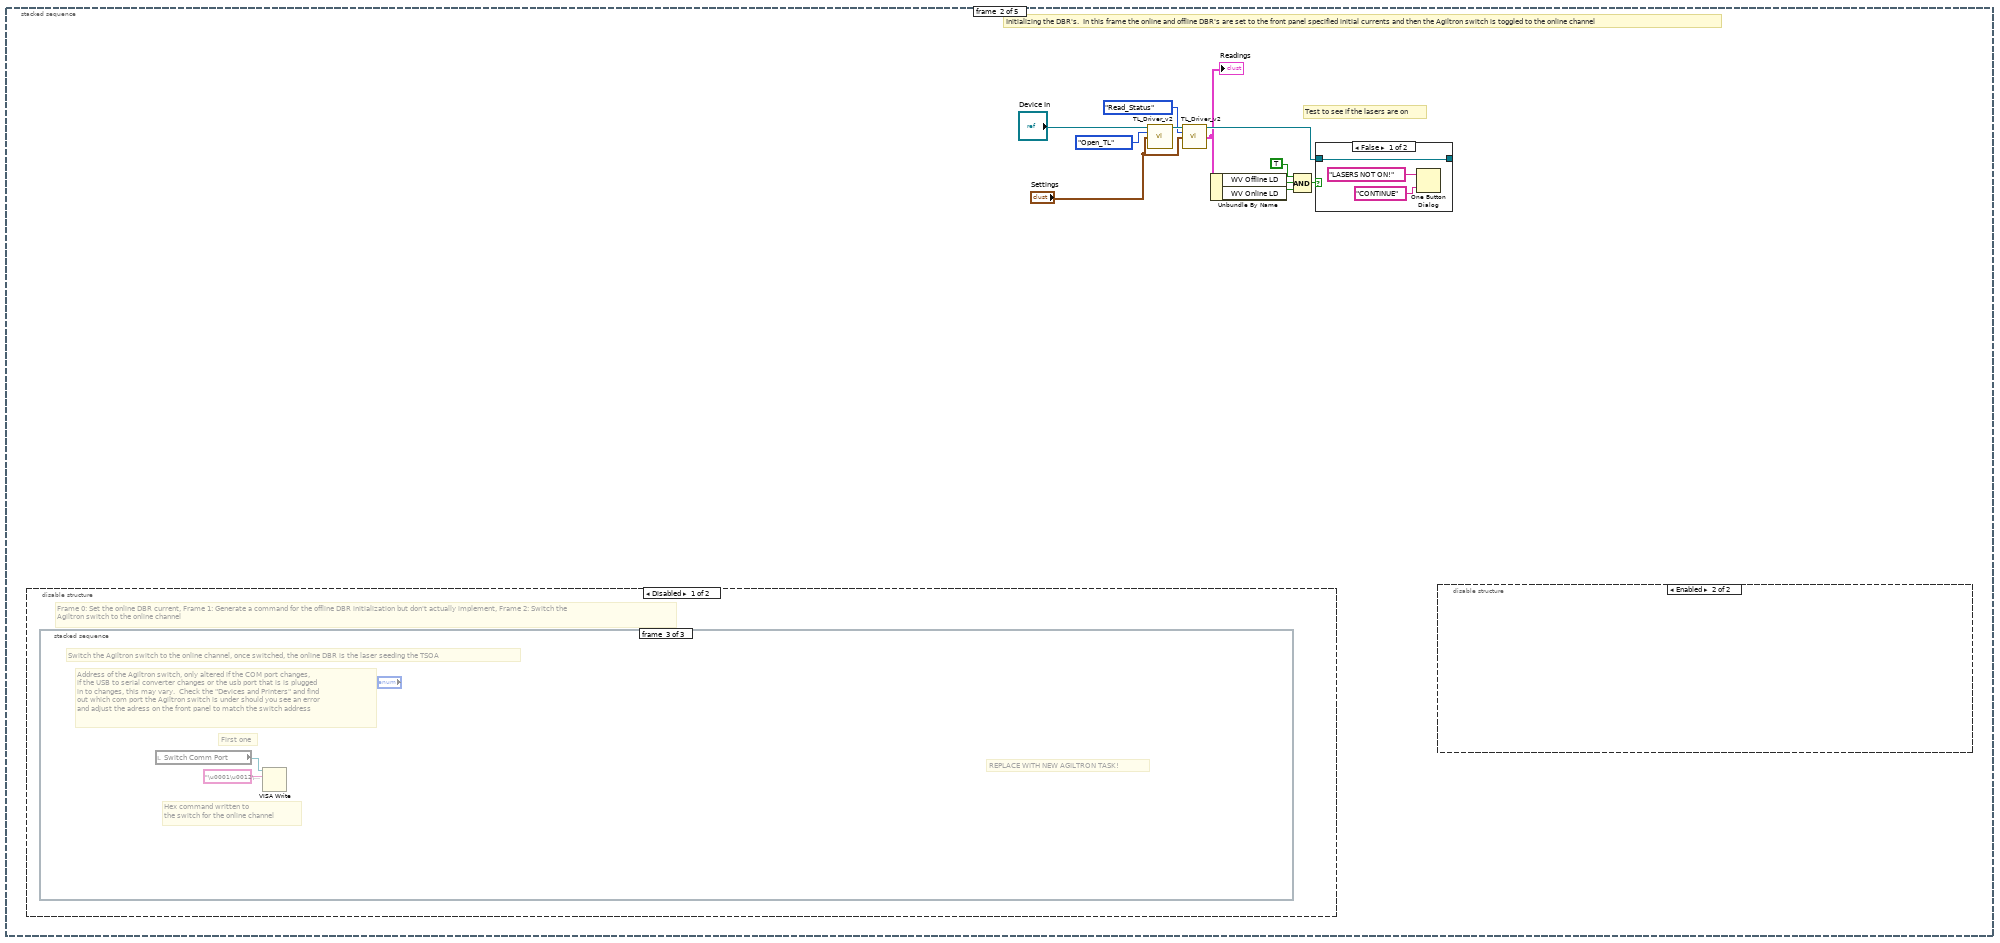
[diagram p7: hidden frame]
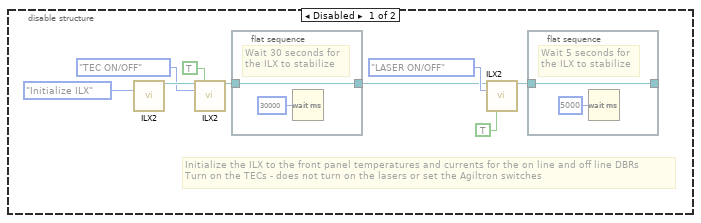
[diagram p9: hidden frame]
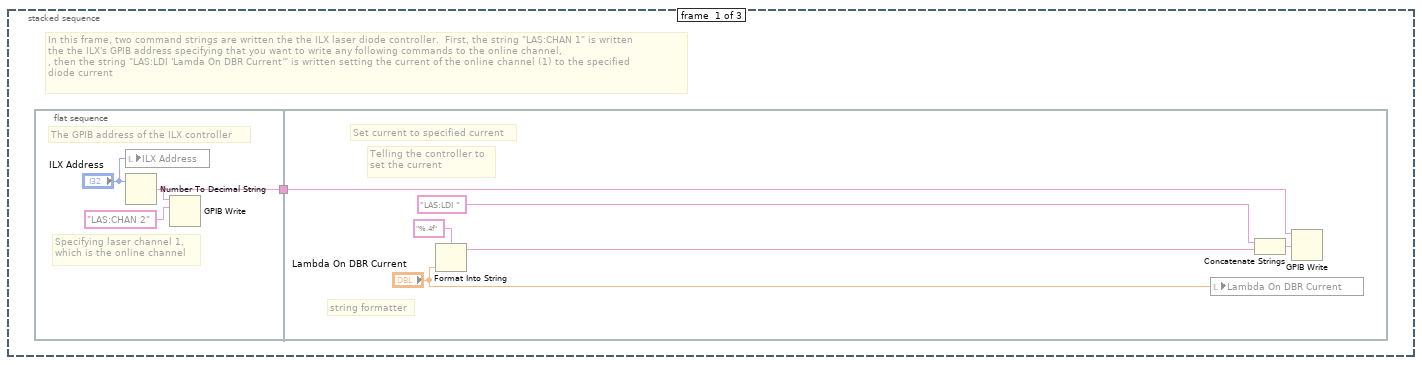
[diagram p10: hidden frame]
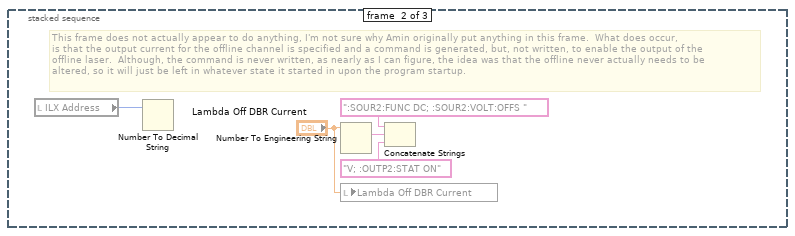
[diagram p11: hidden frame]
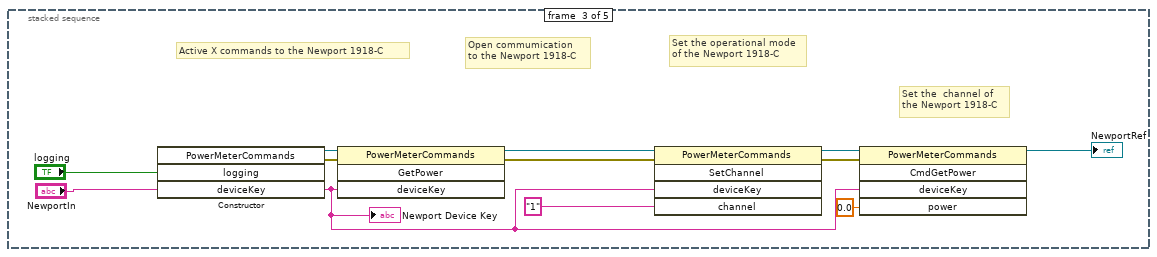
[diagram p13: hidden frame]
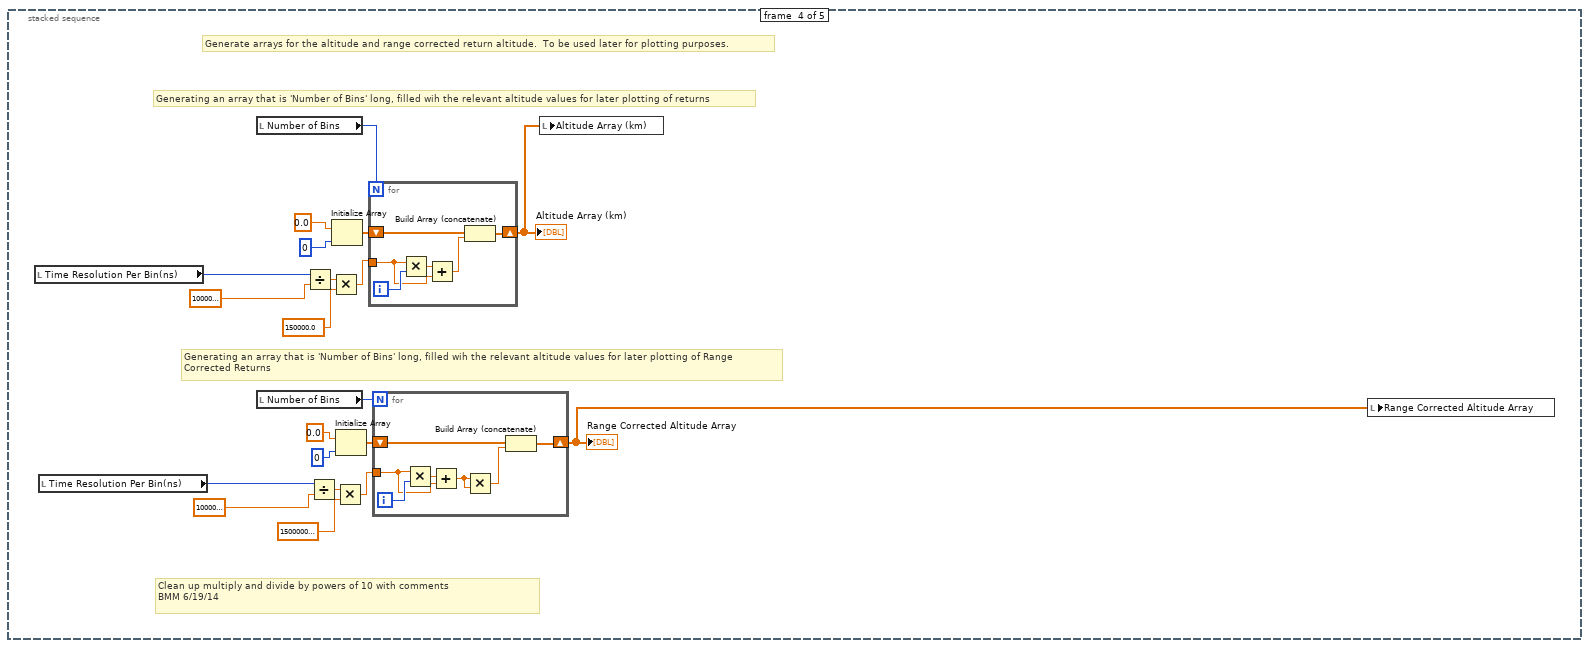
[diagram p14: hidden frame]
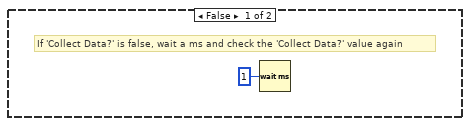
[diagram p15: hidden frame]
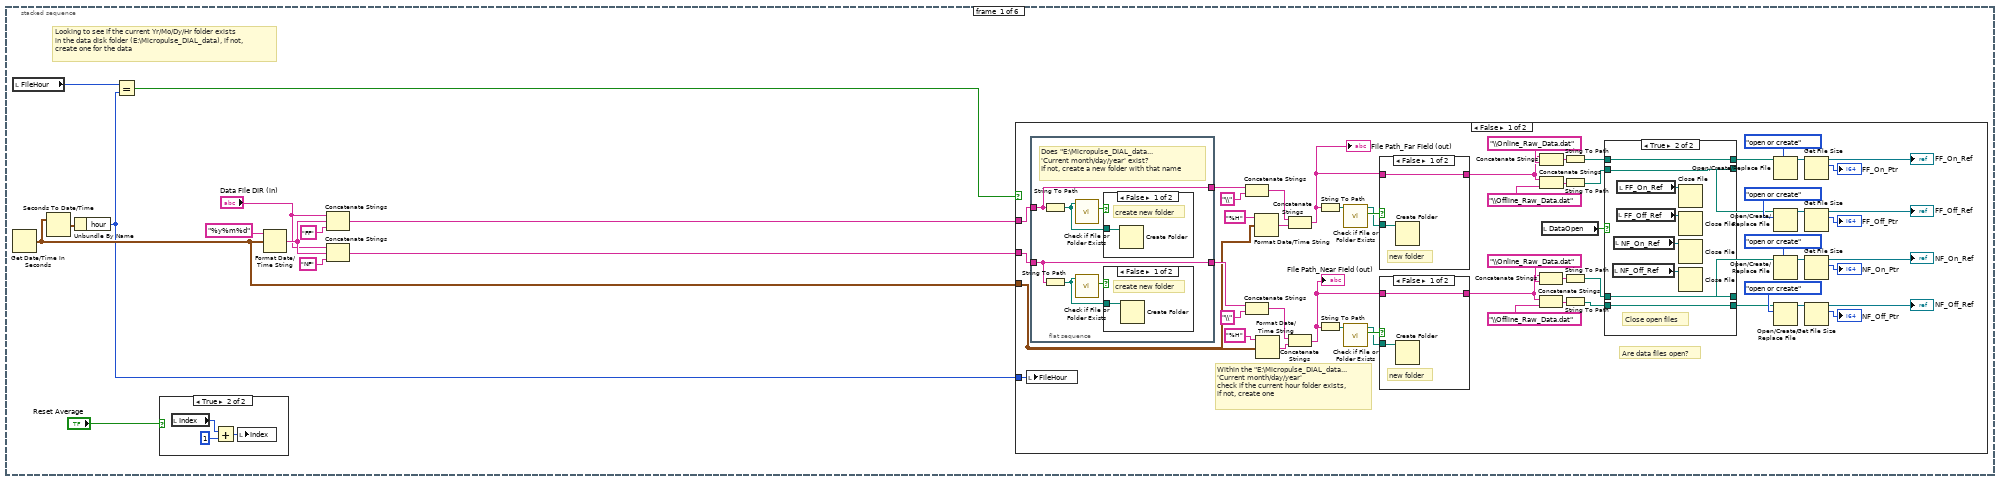
[diagram p16: hidden frame]
diagram:
  # "Frame 0: Initialize the scaler card (and start the MCSC)\nFrame 1: Initialize the DBR's\nFrame 2: Generate address string for talking the to Newport Power meter\nFrame 3: Generate altitude axes for regular and range corrected returns\nFrame 4: Collect data"
  n1 = stacked-sequence {
    tunnel: [_ _ _ _ w128] -> w3
    frame #0 {
      # "Open Bristol WM"
      n2 = disable-structure shown="Enabled" {
        disable-tunnel: [w16 _] -> w5
        frame Enabled {
          # "Initialization of the AMCS card, this where all of the scaler card parameters\nsuch as number of channels and accumulates is written to the card"
          n3 = stacked-sequence {
            tunnel: ["Time Resolution Per Bin(ns)"] -> w16
            frame #0 {
              # "Sets The Registers Of The Card"
              # "Number Of Channels Used"
              n4 = To Unsigned Long Integer(number="Sync Pulse Polarity") -> (unsigned 32bit integer=w18:u32)
              n5 = To Unsigned Long Integer(number="Pulse A Polarity") -> (unsigned 32bit integer=w22:u32)
              n6 = To Unsigned Long Integer(number="Pulse B Polarity") -> (unsigned 32bit integer=w20:u32)
              n7 = expression code="x*4"(w18) -> (w27:u32)
              n8 = expression code="x*2"(w22) -> (w26:u32)
              n9 = expression code="(x-1)*256"(u32 4 ("Number of Channels Used")) -> (w25:u32)
              n10 = expression code="x/10"("Time Resolution Per Bin(ns)") -> (w28:u32)
              n11 = expression code="x/80"("Pulse A Delay(ns)") -> (w35:u32)
              n12 = expression code="x/80"("Pulse B Delay(ns)") -> (w37:u32)
              n13 = expression code="x/10"("Accumulation Delay(ns)") -> (w36:u32)
              n14 = Compound Arithmetic op=ADD(w27, w26, w20, w25) -> (w24:u32)
              n15 = Build Array(w24, "Number of Bins", "Number of Accumulates", w28, w35, w37, w36) -> ()  [unwired: 1 out]
              n16 = local write "ns scale"("Time Resolution Per Bin(ns)") -> ()
              n17 = local write "y offset"("Accumulation Delay(ns)") -> ()
              n18 = local write "bins"("Number of Bins") -> ()
            }
          }
        }
        frame Disabled {
        }
      }
      n19 = Multiply(x=0.15, y=w5) -> (x*y=w4:dbl)
      "gate size" <- w4
      n20 = local read "WS_On/Off"() -> (w7:bool)
      n21 = local read "Number of Bins"() -> (w11:u32)
      n22 = case shown="True" w7 {
        frame False {
        }
        frame True {
          n23 = call "T_RH_P.vi"("VISA in"="WS visa", "WS_Commands"=enum16{"OpenWS", "ReadTRHP", "CloseWS"}."OpenWS") -> ("TRHP"=→"TRHP":T13)  [unwired: 11 in, 2 out]
        }
      }
      n24 = property on="CH 3 (HSRL comb) counts display" class="IntChart (strict)"("YScale.Multiplier"=w4) -> ()  [unwired: 2 in, 2 out]
      n25 = property on="Absolute Humdity" class="IntChart (strict)"("YScale.Multiplier"=w4) -> ()  [unwired: 2 in, 2 out]
      n26 = property on="CH 1 (WV off) counts display" class="IntChart (strict)"("YScale.Multiplier"=w4) -> ()  [unwired: 2 in, 2 out]
      n27 = property on="NRB HSRL Combined" class="IntChart (strict)"("YScale.Multiplier"=w4) -> ()  [unwired: 2 in, 2 out]
      n28 = property on="NRB WV Offline" class="IntChart (strict)"("YScale.Multiplier"=w4) -> ()  [unwired: 2 in, 2 out]
      n29 = Decrement(x=w11) -> (x-1=w10:u32)
      n30 = Subtract(x=w10, y="background length") -> (x-y=→"background start":u32)
      "Index" <- 0 ("Index")
    }
    frame #1 {
      # "Test to see if the lasers are on"
      # "Initializing the DBR's.  In this frame the online and offline DBR's are set to the front panel specified initial currents and then the Agiltron switch is toggled to the online channel"
      n31 = disable-structure shown="Disabled" {
        frame Disabled {
          # "Frame 0: Set the online DBR current, Frame 1: Generate a command for the offline DBR initialization but don't actually implement, Frame 2: Switch the \nAgiltron switch to the online channel"
          n32 = stacked-sequence {
            frame #0 {
              # "In this frame, two command strings are written the the ILX laser diode controller.  First, the string \"LAS:CHAN 1\" is written\nthe the ILX's GPIB address specifying that you want to write any following commands to the online channel,\n, then the string \"LAS:LDI 'Lamda On DBR Current'\" is written setting the current of the online channel (1) to the specified \ndiode current"
              n33 = flat-sequence {
                tunnel: [w68] -> w66
                tunnel: w66 -> [w70]
                frame #0 {
                  # "The GPIB address of the ILX controller"
                  # "Specifying laser channel 1,\nwhich is the online channel"
                  n34 = local write "ILX Address"("ILX Address") -> ()
                  n35 = Number To Decimal String(number="ILX Address") -> (decimal integer string=w68:string)  [unwired: 1 in]
                  n36 = GPIB Write(0:w68, 1:"LAS:CHAN 2") -> ()  [unwired: 3 in, 2 out]
                }
                frame #1 {
                  # "Telling the controller to\nset the current"
                  # "string formatter"
                  # "Set current to specified current"
                  n37 = Format Into String(format string="%.4f" ("Format String"), "Lambda On DBR Current") -> (resulting string=w73:string)  [unwired: 2 in, 1 out]
                  n38 = local write "Lambda On DBR Current"("Lambda On DBR Current") -> ()
                  n39 = Concatenate Strings("LAS:LDI ", w73) -> (w74:string)
                  n40 = GPIB Write(0:w70, 1:w74) -> ()  [unwired: 3 in, 2 out]
                }
              }
            }
            frame #1 {
              # "This frame does not actually appear to do anything, I'm not sure why Amin originally put anything in this frame.  What does occur, \nis that the output current for the offline channel is specified and a command is generated, but, not written, to enable the output of the\noffline laser.  Although, the command is never written, as nearly as I can figure, the idea was that the offline never actually needs to be \naltered, so it will just be left in whatever state it started in upon the program startup."
              n41 = local read "ILX Address"() -> (w76:i32)
              n42 = Number To Decimal String(number=w76) -> ()  [unwired: 1 in, 1 out]
              n43 = Number To Engineering String(4:"Lambda Off DBR Current") -> (0:w80:string)  [unwired: 3 in]
              n44 = local write "Lambda Off DBR Current"("Lambda Off DBR Current") -> ()
              n45 = Concatenate Strings(":SOUR2:FUNC DC; :SOUR2:VOLT:OFFS ", w80, "V; :OUTP2:STAT ON") -> ()  [unwired: 1 out]
            }
            frame #2 {
              # "REPLACE WITH NEW AGILTRON TASK!"
              # "First one"
              # "Address of the Agiltron switch, only altered if the COM port changes,\nif the USB to serial converter changes or the usb port that is is plugged\nin to changes, this may vary.  Check the \"Devices and Printers\" and find \nout which com port the Agiltron switch is under should you see an error \nand adjust the adress on the front panel to match the switch address"
              # "Hex command written to \nthe switch for the online channel"
              # "Switch the Agiltron switch to the online channel, once switched, the online DBR is the laser seeding the TSOA"
              n46 = local read "Switch Comm Port"() -> (w81:refnum<visa-resource-name>)
              n47 = VISA Write(VISA resource name=w81, write buffer="\u0001\u0012\u0000\u0002") -> ()  [unwired: 1 in, 3 out]
            }
          }
        }
        frame Enabled {
        }
      }
      n48 = call "TL_Driver_v2.vi"("Device In"="Device In", "Commands"=T9."Open_TL", "Settings"="Settings") -> ("Device Out"=w46:refnum<visa-resource-name>)  [unwired: 9 in, 3 out]
      n49 = call "TL_Driver_v2.vi"("Device In"=w46, "Commands"=T9."Read_Status", "Settings"="Settings") -> ("Device Out"=w44:refnum<visa-resource-name>, "Readings"=w38:T7)  [unwired: 9 in, 2 out]
      "Readings" <- w38
      n50 = Unbundle By Name(w38) -> ("WV Offline LD"=w41:bool, "WV Online LD"=w42:bool)
      n51 = Compound Arithmetic op=AND(TRUE, w41, w42) -> (w40:bool)
      n52 = case shown="False" w40 {
        tunnel: w44 -> [w49 w52]
        tunnel: [w49 w52] -> _
        frame False {
          n53 = One Button Dialog(message="LASERS NOT ON!", button name ("OK")="CONTINUE") -> ()  [unwired: 1 out]
        }
        frame True {
        }
      }
      n54 = disable-structure shown="Enabled" {
        frame Disabled {
          # "Initialize the ILX to the front panel temperatures and currents for the on line and off line DBRs\nTurn on the TECs - does not turn on the lasers or set the Agiltron switches"
          n55 = call "ILX2.vi"("ILX Command"=T10."Initialize ILX") -> ("Device Out"=w60:refnum<visa-resource-name>)  [unwired: 10 in, 4 out]
          n56 = call "ILX2.vi"("Device In"=w60, "TEC Control"=TRUE, "ILX Command"=T10."TEC ON/OFF") -> ("Device Out"=w57:refnum<visa-resource-name>)  [unwired: 8 in, 4 out]
          n57 = flat-sequence {
            tunnel: w57 -> [w64]
            tunnel: [w64] -> w54
            frame #0 {
              # "Wait 30 seconds for\nthe ILX to stabilize"
              n58 = Wait (ms)(milliseconds to wait=u32 30000) -> ()  [unwired: 1 out]
            }
          }
          n59 = call "ILX2.vi"("Device In"=w54, "ILX Command"=T10."LASER ON/OFF", "Laser Control"=TRUE ("TEC Control")) -> ("Device Out"=w53:refnum<visa-resource-name>)  [unwired: 8 in, 4 out]
          n60 = flat-sequence {
            tunnel: w53 -> [w62]
            tunnel: [w62] -> _
            frame #0 {
              # "Wait 5 seconds for\nthe ILX to stabilize"
              n61 = Wait (ms)(milliseconds to wait=u32 5000) -> ()  [unwired: 1 out]
            }
          }
        }
        frame Enabled {
        }
      }
    }
    frame #2 {
      # "Active X commands to the Newport 1918-C"
      # "Set the  channel of\nthe Newport 1918-C"
      # "Set the operational mode\nof the Newport 1918-C"
      # "Open commumication\nto the Newport 1918-C"
      n62 = constructor class="PowerMeterCommands"("logging"="logging", "deviceKey"="NewportIn") -> (reference out=w94:refnum<k24>, error out=w91:errorcluster, "deviceKey"=w86:string)  [unwired: 3 in, 2 out]
      "Newport Device Key" <- w86
      n63 = invoke class="PowerMeterCommands" method="GetPower"(reference=w94, error in=w91, "deviceKey"=w86) -> (reference out=w93:refnum<k24>, error out=w90:errorcluster)  [unwired: 1 in, 2 out]
      n64 = invoke class="PowerMeterCommands" method="SetChannel"(reference=w93, error in=w90, "deviceKey"=w86, "channel"="1") -> (reference out=w87:refnum<k24>, error out=w89:errorcluster)  [unwired: 1 in, 3 out]
      n65 = invoke class="PowerMeterCommands" method="CmdGetPower"(reference=w87, error in=w89, "deviceKey"=w86, "power"=sgl 0.0) -> (reference out=→"NewportRef":refnum<k24>)  [unwired: 1 in, 4 out]
    }
    frame #3 {
      # "Clean up multiply and divide by powers of 10 with comments\nBMM 6/19/14"
      # "Generating an array that is 'Number of Bins' long, filled wih the relevant altitude values for later plotting of Range \nCorrected Returns"
      # "Generating an array that is 'Number of Bins' long, filled wih the relevant altitude values for later plotting of returns"
      # "Generate arrays for the altitude and range corrected return altitude.  To be used later for plotting purposes."
      n66 = local read "Time Resolution Per Bin(ns)"() -> (w107:u32)
      n67 = local read "Time Resolution Per Bin(ns)"() -> (w97:u32)
      n68 = local read "Number of Bins"() -> (w110:u32)
      n69 = local read "Number of Bins"() -> (w100:u32)
      n70 = Divide(x=w107, y=1000000000.0) -> (x/y=w105:dbl)
      n71 = Divide(x=w97, y=1000000000.0) -> (x/y=w95:dbl)
      n72 = Multiply(x=w105, y=150000.0) -> (x*y=w108:dbl)
      n73 = Initialize Array(0.0, 0) -> (w113:dbl[])
      n74 = Multiply(x=w95, y=150000000.0) -> (x*y=w98:dbl)
      n75 = Initialize Array(0.0, 0) -> (w103:dbl[])
      n76 = for {
        N: w110 -> [_]
        shift-right: [w126] -> w111
        shift-left: w113 -> [w127]
        tunnel: w108 -> [w123]
        i -> [w125]
        n77 = Multiply(x=w123, y=w125) -> (x*y=w124:dbl)
        n78 = Add(x=w124, y=w123) -> (x+y=w122:dbl)
        n79 = Build Array (concatenate)(w127, w122) -> (w126:dbl[])
      }
      "Altitude Array (km)" <- w111
      n80 = for {
        N: w100 -> [_]
        shift-right: [w120] -> w101
        shift-left: w103 -> [w121]
        tunnel: w98 -> [w116]
        i -> [w119]
        n81 = Multiply(x=w116, y=w119) -> (x*y=w117:dbl)
        n82 = Add(x=w117, y=w116) -> (x+y=w115:dbl)
        n83 = Multiply(x=w115, y=w115) -> (x*y=w118:dbl)
        n84 = Build Array (concatenate)(w121, w118) -> (w120:dbl[])
      }
      "Range Corrected Altitude Array" <- w101
      n85 = local write "Altitude Array (km)"(w111) -> ()
      n86 = local write "Range Corrected Altitude Array"(w101) -> ()
    }
    frame #4 {
      # "Frame 4: Collect data from the scaler card and process and file it"
      n87 = while {
        tunnel: ["stop"] -> w128
        i -> [w129]
        stop <- "stop" stop-if-true
        # "While loop continues data collection cycle"
        n88 = case shown="True" "Collect Data?" {
          frame False {
            # "If 'Collect Data?' is false, wait a ms and check the 'Collect Data?' value again"
            n89 = Wait (ms)(milliseconds to wait=u32 1) -> ()  [unwired: 1 out]
          }
          frame True {
            # "Frame 3: Read the offline wavelength and lock if necessary (code not finished), read output power, read offline data, perform calculations and plot/save offline and NRB data, switch to online\nFrame 4: Calculate the absorption cross section (if wavelength, T, or P changed)\nFrame 5: Calculate Water Vapor Number density and plot"
            # "Frame 0: Create folders and file paths for logging the data, initialize averaging index\nFrame 1: Import current pressure and temperature data from COE weather station\nFrame 2: Read the online wavelength and lock if necessary, read online data and output power\n, plot and save online data, switch to offline DBR"
            # "If 'Collect Data?' is true, collect, process, and log data"
            n90 = stacked-sequence {
              frame #0 {
                # "Looking to see if the current Yr/Mo/Dy/Hr folder exists\nin the data disk folder (E:\\Micropulse_DIAL_data), if not,\ncreate one for the data"
                n91 = local read "FileHour"() -> (w142:i32)
                n92 = Get Date/Time In Seconds() -> (seconds since 1Jan1904=w134:timestamp)
                n93 = Seconds To Date/Time(time stamp (now)=w134) -> (date time rec=w144:T14)  [unwired: 1 in]
                n94 = Unbundle By Name(w144) -> ("hour"=w133:i32)
                n95 = Equal?(x=w142, y=w133) -> (x = y?=w143:bool)
                n96 = case shown="True" "Reset Average" {
                  frame False {
                    n97 = local write "Index"(0 ("Index")) -> ()
                  }
                  frame True {
                    n98 = local read "Index"() -> (w232:i32)
                    n99 = Add(x=w232, y=1) -> (x+y=w231:i32)
                    n100 = local write "Index"(w231) -> ()
                  }
                }
                n101 = Format Date/Time String(time format string (%c)="%y%m%d", seconds (now)=w134) -> (date/time string=w138:string)  [unwired: 1 in]
                n102 = Concatenate Strings("Data File DIR (in)", w138, "FF" ("string")) -> (w140:string)
                n103 = Concatenate Strings("Data File DIR (in)", w138, "NF" ("string")) -> (w135:string)
                n104 = case shown="False" w143 {
                  tunnel: w140 -> [w202 _]
                  tunnel: w135 -> [w201 _]
                  tunnel: w134 -> [w188 _]
                  tunnel: w133 -> [w164 _]
                  frame False {
                    # "Are data files open?"
                    # "Within the \"E:\\Micropulse_DIAL_data...\n'Current month/day/year' \ncheck if the current hour folder exists,\nif not, create one"
                    n105 = local write "FileHour"(w164) -> ()
                    n106 = flat-sequence {
                      tunnel: [w222] -> w189
                      tunnel: w202 -> [w221]
                      tunnel: w201 -> [w222]
                      tunnel: [w221] -> w190
                      frame #0 {
                        # "Does \"E:\\Micropulse_DIAL_data...\n'Current month/day/year' exist?\nIf not, create a new folder with that name"
                        n107 = String To Path(string=w221) -> (path=w226:path)
                        n108 = String To Path(string=w222) -> (path=w224:path)
                        n109 = call <vilib>:"Check if File or Folder Exists.vi"("path"=w226) -> ("file or folder exists?"=w225:bool)  [unwired: 8 in, 2 out]
                        n110 = call <vilib>:"Check if File or Folder Exists.vi"("path"=w224) -> ("file or folder exists?"=w223:bool)  [unwired: 8 in, 2 out]
                        n111 = case shown="False" w225 {
                          tunnel: w226 -> [w228 _]
                          frame False {
                            # "create new folder"
                            n112 = Create Folder(path (use dialog)=w228) -> ()  [unwired: 2 in, 3 out]
                          }
                          frame True {
                            # "Folder exists\ndo nothing"
                          }
                        }
                        n113 = case shown="False" w223 {
                          tunnel: w224 -> [w227 _]
                          frame False {
                            # "create new folder"
                            n114 = Create Folder(path (use dialog)=w227) -> ()  [unwired: 2 in, 3 out]
                          }
                          frame True {
                            # "Folder exists\ndo nothing"
                          }
                        }
                      }
                    }
                    n115 = Concatenate Strings(w190, "\\" ("string")) -> (w197:string)
                    n116 = Concatenate Strings(w189, "\\" ("string")) -> (w192:string)
                    n117 = Format Date/Time String(time format string (%c)="%H", seconds (now)=w188) -> (date/time string=w200:string)  [unwired: 1 in]
                    n118 = Format Date/Time String(time format string (%c)="%H", seconds (now)=w188) -> (date/time string=w195:string)  [unwired: 1 in]
                    n119 = Concatenate Strings(w197, w200) -> (w160:string)
                    "File Path_Far Field (out)" <- w160
                    n120 = Concatenate Strings(w192, w195) -> (w161:string)
                    "File Path_Near Field (out)" <- w161
                    n121 = String To Path(string=w160) -> (path=w198:path)
                    n122 = String To Path(string=w161) -> (path=w193:path)
                    n123 = call <vilib>:"Check if File or Folder Exists.vi"("path"=w198) -> ("file or folder exists?"=w187:bool, "dup path"=w185:path)  [unwired: 8 in, 1 out]
                    n124 = call <vilib>:"Check if File or Folder Exists.vi"("path"=w193) -> ("file or folder exists?"=w186:bool, "dup path"=w184:path)  [unwired: 8 in, 1 out]
                    n125 = case shown="False" w187 {
                      tunnel: w185 -> [w219 _]
                      tunnel: w160 -> [w218 w220]
                      tunnel: [w218 w220] -> w158
                      frame False {
                        # "new folder"
                        n126 = Create Folder(path (use dialog)=w219) -> ()  [unwired: 2 in, 3 out]
                      }
                      frame True {
                        # "Folder exists\ndo nothing"
                      }
                    }
                    n127 = case shown="False" w186 {
                      tunnel: w184 -> [w216 _]
                      tunnel: w161 -> [w215 w217]
                      tunnel: [w215 w217] -> w159
                      frame False {
                        # "new folder"
                        n128 = Create Folder(path (use dialog)=w216) -> ()  [unwired: 2 in, 3 out]
                      }
                      frame True {
                        # "Folder exists\ndo nothing"
                      }
                    }
                    n129 = Concatenate Strings(w159, "\\Online_Raw_Data.dat" ("string")) -> (w178:string)
                    n130 = Concatenate Strings(w159, "\\Offline_Raw_Data.dat" ("string")) -> (w177:string)
                    n131 = Concatenate Strings(w158, "\\Online_Raw_Data.dat" ("string")) -> (w183:string)
                    n132 = Concatenate Strings(w158, "\\Offline_Raw_Data.dat" ("string")) -> (w182:string)
                    n133 = local read "DataOpen"() -> (w175:bool)
                    n134 = String To Path(string=w183) -> (path=w174:path)
                    n135 = String To Path(string=w182) -> (path=w173:path)
                    n136 = String To Path(string=w178) -> (path=w172:path)
                    n137 = String To Path(string=w177) -> (path=w171:path)
                    n138 = case shown="True" w175 {
                      tunnel: w174 -> [w206 w210]
                      tunnel: [w206 w210] -> w168
                      tunnel: w173 -> [w205 w209]
                      tunnel: [w205 w209] -> w167
                      tunnel: w172 -> [w204 w208]
                      tunnel: [w204 w208] -> w166
                      tunnel: [w203 w207] -> w165
                      tunnel: w171 -> [w203 w207]
                      frame False {
                        # "No files open\ndo nothing"
                      }
                      frame True {
                        # "Close open files"
                        n139 = local read "NF_Off_Ref"() -> (w212:refnum<file>)
                        n140 = local read "NF_On_Ref"() -> (w211:refnum<file>)
                        n141 = local read "FF_Off_Ref"() -> (w214:refnum<file>)
                        n142 = local read "FF_On_Ref"() -> (w213:refnum<file>)
                        n143 = Close File(refnum=w213) -> ()  [unwired: 1 in, 2 out]
                        n144 = Close File(refnum=w214) -> ()  [unwired: 1 in, 2 out]
                        n145 = Close File(refnum=w211) -> ()  [unwired: 1 in, 2 out]
                        n146 = Close File(refnum=w212) -> ()  [unwired: 1 in, 2 out]
                      }
                    }
                    n147 = Open/Create/Replace File(file path (use dialog)=w168, operation (0:open)=T11."open or create") -> (refnum out=w154:refnum<file>)  [unwired: 4 in, 2 out]
                    n148 = Open/Create/Replace File(file path (use dialog)=w167, operation (0:open)=T11."open or create") -> (refnum out=w155:refnum<file>)  [unwired: 4 in, 2 out]
                    n149 = Open/Create/Replace File(file path (use dialog)=w166, operation (0:open)=T11."open or create") -> (refnum out=w156:refnum<file>)  [unwired: 4 in, 2 out]
                    n150 = Open/Create/Replace File(file path (use dialog)=w165, operation (0:open)=T11."open or create") -> (refnum out=w157:refnum<file>)  [unwired: 4 in, 2 out]
                    n151 = Get File Size(file=w154) -> (refnum out=→"FF_On_Ref":refnum<file>, size (in bytes)=→"FF_On_Ptr":i64)  [unwired: 1 in, 1 out]
                    n152 = Get File Size(file=w155) -> (refnum out=→"FF_Off_Ref":refnum<file>, size (in bytes)=→"FF_Off_Ptr":i64)  [unwired: 1 in, 1 out]
                    n153 = Get File Size(file=w156) -> (refnum out=→"NF_On_Ref":refnum<file>, size (in bytes)=→"NF_On_Ptr":i64)  [unwired: 1 in, 1 out]
                    n154 = Get File Size(file=w157) -> (refnum out=→"NF_Off_Ref":refnum<file>, size (in bytes)=→"NF_Off_Ptr":i64)  [unwired: 1 in, 1 out]
                  }
                  frame True {
                    # "Don't need to do anything!"
                  }
                }
              }
              frame #1 {
                # "Writing and plotting retrieved\nweather parameters"
                # "Matlab script goes online and retrieves most recent press, temp, and relative humidity data \nfrom the weather station on the roof of Cobleigh"
                # "Importing the current weather conditions from the COE weather station"
                n155 = disable-structure shown="Disabled" {
                  frame Disabled {
                    n156 = script code="%try\n%s=urlread('http://www.coe.montana.edu/ee/weather/mostCurrentCSV.php');\n%amin=textscan(s,'%s %s %s %s %s %s %s %s %s %s %s %s %s');\n%data=amin{1}{2};\n%[test remain]=strtok(data,',');\n%remain=str2num(remain);\n%press=remain(3)./1000;\n%temp=remain(5);\n%RH=remain(7);\n%catch\npress=.850;\ntemp=20;\nRH=40;\n%end"() -> ()  [unwired: 1 in, 4 out]
                  }
                  frame Enabled {
                  }
                }
                n157 = local read "WS_On/Off"() -> (w233:bool)
                n158 = case shown="True" w233 {
                  frame False {
                  }
                  frame True {
                    n159 = local read "WS visa"() -> (w238:refnum<visa-resource-name>)
                    n160 = call "T_RH_P.vi"("VISA in"=w238, "WS_Commands"=enum16{"OpenWS", "ReadTRHP", "CloseWS"}."ReadTRHP") -> ("TRHP"=w234:T13)  [unwired: 11 in, 2 out]
                    n161 = local write "TRHP"(w234) -> ()
                    n162 = Unbundle By Name(w234) -> ("Temp"=→"Temperature (C)":dbl, "RelH"=→"Relative Humdity (%)":dbl, "Press"=→"Pressure (mb)":dbl)
                  }
                }
              }
              frame #2 {
                # "Frame 3: Read, process, and plot online data\nFrame 4:\nFrame 5: Write the data to the folders from Frame 0 of outter sequence"
                # "Frame 0: Read the online wavelength and adjust to locking tolerance if out of range, Switch to offline DBR\nFrame 1: Read the output power from the Newport meter, calculate and plot the output pulse energy\nFrame 2: Wait 'Scalar Wait Time' for buffer to clear other wavelength data"
                # "Online"
                n163 = stacked-sequence {
                  frame #0 {
                    # "Read the online wavelength and continue adjusting the online DBR if outside the wavelength tolerance\nuntil it is within tolerance"
                    n164 = while {
                      i -> [w241]
                      stop <- w240 stop-if-true
                      # "Frame 2: Decrement DBR current if above tolerance\nFrame 3: Increment DBR current if below tolerance"
                      # "Frame 0: Read the current wavelength from the wavemeter\nFrame 1: Calculate the difference between desired and actual wavelength"
                      # "Continue reading and adjusting online DBR current until within locking tolerance"
                      n165 = stacked-sequence {
                        tunnel: w241 -> [w243 _ _ _ _]
                        tunnel: [_ _ w259 _ _] -> w240
                        frame #0 {
                          n166 = Equal To 0?(x=w243) -> (x = 0?=w242:bool)
                          n167 = case shown="True" w242 {
                            frame False {
                            }
                            frame True {
                              # "Set the wavemeter switch to WV Online"
                              n168 = flat-sequence {
                                frame #0 {
                                n169 = Build Array(FALSE ("Boolean")) -> (w246:bool[])
                                n170 = call-poly <vilib>:"DAQmx Write.vi"("task/channels in"=refnum<k21> "BristolWM", "data"=w246) -> ()  [unwired: 11 in, 3 out]
                                }
                                frame #1 {
                                n171 = Build Array(FALSE ("Boolean")) -> (w249:bool[])
                                n172 = call-poly <vilib>:"DAQmx Write.vi"("task/channels in"=refnum<k21> "HSRL_WV_switch", "data"=w249) -> ()  [unwired: 11 in, 3 out]
                                }
                              }
                            }
                          }
                        }
                        frame #1 {
                          # "Reading the wavelength from the wavemeter"
                          n173 = flat-sequence {
                            tunnel: [w252] -> w251
                            tunnel: w251 -> [w255]
                            tunnel: [w254] -> w250
                            tunnel: w250 -> [w258]
                            frame #0 {
                              n174 = local read "Bristol In"() -> (w253:i32)
                              n175 = dll-call lib="C:/Users/H2ODial/Desktop/Shared Telescope WV DIAL Code/bristol/CLDevIface.dll" fn="CLOpenUSBSerialDevice"("commPort"=w253) -> ("return type"=w252:i32)  [unwired: 4 in, 2 out]
                            }
                            frame #1 {
                              n176 = dll-call lib="C:/Users/H2ODial/Desktop/Shared Telescope WV DIAL Code/bristol/CLDevIface.dll" fn="CLGetLambdaReading"("devHandle"=w255) -> ("return type"=→"WV Online Read (nm)":dbl, "devHandle"=w254:i32)  [unwired: 3 in, 2 out]
                            }
                            frame #2 {
                              n177 = dll-call lib="C:/Users/H2ODial/Desktop/Shared Telescope WV DIAL Code/bristol/CLDevIface.dll" fn="CLCloseDevice"("commPort"=w258) -> ("return type"=w257:i32)  [unwired: 4 in, 2 out]
                              n178 = local write "Bristol Out"(w257) -> ()
                            }
                          }
                        }
                        frame #2 {
                          # "If WL difference is within tolerance, stop looping, and illuminate 'Wavelength Lock Online' indicator"
                          # "Calculating the difference between the actual and desired online wavelength"
                          n179 = local read "WV Online Read (nm)"() -> (w262:dbl)
                          n180 = local read "Online_Tol"() -> (w267:dbl)
                          n181 = Multiply(x=-1.0, y=w267) -> (x*y=w268:dbl)
                          n182 = Subtract(x=w262, y="WV Online Set (nm)") -> (x-y=w263:dbl)
                          "Online_Diff" <- w263
                          n183 = Greater?(x=w263, y=w268) -> (0:w264:bool)
                          n184 = Less?(x=w263, y=w267) -> (x < y?=w265:bool)
                          n185 = And(x=w264, y=w265) -> (x .and. y?=w261:bool)
                          "WV Online Locked" <- w261
                          n186 = Or(x=w261, y="Cancel online") -> (x .or. y?=w259:bool)
                        }
                        frame #3 {
                          # "If the wavelength difference is greater that 0.0002 nm, decrement the \nDBR current by 0.01 mA"
                          n187 = local read "Online_Diff"() -> (w272:dbl)
                          n188 = Greater Or Equal?(x=w272, y="Online_Tol") -> (x >= y?=w271:bool)
                          n189 = case shown="True" w271 {
                            frame False {
                              # "Wavelength difference is not greater than 0.0002 nm, do nothing"
                            }
                            frame True {
                              # "Generating a command string\nto decrement the current"
                              # "WL difference is greater than 0.0002 nm,\ndecrement the DBR current by 0.01 mA"
                              n190 = local read "Settings"() -> (w279:T6)
                              n191 = local read "temp step size"() -> (w274:dbl)
                              n192 = Unbundle By Name(w279) -> ("WV Online TEC"=w278:dbl)
                              n193 = local read "Device In"() -> (w275:refnum<visa-resource-name>)
                              n194 = Subtract(x=w278, y=w274) -> (x-y=w277:dbl)
                              n195 = Bundle By Name(cluster=w279, "WV Online TEC"=w277, "Module"=T12."WV Online TEC") -> (w281:T6)
                              n196 = call "TL_Driver_v2.vi"("Device In"=w275, "Commands"=T9."SET", "Settings"=w281) -> ("Readings"=w280:T7)  [unwired: 9 in, 3 out]
                              n197 = local write "Settings"(w281) -> ()
                              n198 = local write "Readings"(w280) -> ()
                            }
                          }
                        }
                        frame #4 {
                          # "If WL difference is < 0.0002 nm, increment the DBR current"
                          n199 = local read "Online_Tol"() -> (w283:dbl)
                          n200 = local read "Online_Diff"() -> (w286:dbl)
                          n201 = Multiply(x=-1.0, y=w283) -> (x*y=w282:dbl)
                          n202 = Less Or Equal?(x=w286, y=w282) -> (x <= y?=w285:bool)
                          n203 = case shown="True" w285 {
                            frame False {
                              # "WL difference is no <= to -0.0002 nm, do nothing"
                            }
                            frame True {
                              # "WL difference is < -0.0002,\nincrement the DBR current by 0.01 mA"
                              # "Generating a command string\nto decrement the current"
                              n204 = local read "Settings"() -> (w295:T6)
                              n205 = local read "temp step size"() -> (w288:dbl)
                              n206 = Unbundle By Name(w295) -> ("WV Online TEC"=w292:dbl)
                              n207 = local read "Device In"() -> (w289:refnum<visa-resource-name>)
                              n208 = Add(x=w292, y=w288) -> (x+y=w291:dbl)
                              n209 = Bundle By Name(cluster=w295, "WV Online TEC"=w291, "Module"=T12."WV Online TEC") -> (w294:T6)
                              n210 = call "TL_Driver_v2.vi"("Device In"=w289, "Commands"=T9."SET", "Settings"=w294) -> ("Readings"=w293:T7)  [unwired: 9 in, 3 out]
                              n211 = local write "Settings"(w294) -> ()
                              n212 = local write "Readings"(w293) -> ()
                            }
                          }
                        }
                      }
                    }
                  }
                  frame #1 {
                    # "Converting to pulse energy, assumes 5 percent pickoff"
                    # "Reading the Newport Power meter"
                    # "Reading the output power of the laser transmitter from the Newport power meter, once read, convert to corresponding pulse energy and plot"
                    n213 = local read "Newport Device Key"() -> (w300:string)
                    n214 = local read "NewportRef"() -> (w296:refnum<k24>)
                    n215 = disable-structure shown="Enabled" {
                      frame Enabled {
                        # "Plotting the online and offling pulse energies"
                        n216 = local read "Online Pulse Energy"() -> (w311:dbl)
                        n217 = local read "Offline Pulse Energy"() -> (w310:dbl)
                        n218 = Bundle("Online Pulse Energy"=w311, "Offline Pulse Energy"=w310) -> (→"Pulse Energy (Micro Joule)":T15)  [unwired: 1 in]
                      }
                      frame Disabled {
                      }
                    }
                    n219 = Number To Decimal String(number="SampleSize") -> (decimal integer string=w298:string)  [unwired: 1 in]
                    n220 = invoke class="PowerMeterCommands" method="PerformDAQ"(reference=w296, "deviceKey"=w300, "interval"="1", "sampleSize"=w298) -> ("PerformDAQ"=w301:dbl[])  [unwired: 2 in, 5 out]
                    n221 = call-poly <vilib>:"Mean.vi"("X"=w301) -> ("mean"=w299:dbl)  [unwired: 1 out]
                    n222 = Multiply(x=w299, y=1000.0) -> (x*y=w307:dbl)
                    n223 = Divide(x=w307, y=0.05) -> (x/y=w305:dbl)
                    n224 = Divide(x=w305, y=7.0) -> (x/y=→"Online Pulse Energy":dbl)
                  }
                  frame #2 {
                    # "Wait 'Scalar Wait Time' for the next available batch of scalar card data"
                    n225 = local read "AMCS_Profile"() -> (w312:i32)
                    n226 = disable-structure shown="Disabled" {
                      frame Disabled {
                        # "Waiting 'Scalar Wait Time'"
                        n227 = Wait (ms)(milliseconds to wait="Scalar Wait Time") -> ()  [unwired: 1 out]
                      }
                      frame Enabled {
                      }
                    }
                    n228 = while {
                      tunnel: [w319] -> w313
                      tunnel: [w315] -> _
                      tunnel: w312 -> [w315]
                      stop <- w317 stop-if-true
                      n229 = global read "AMCS_Data.vi" "AMCS_Profile"() -> (w319:i32)
                      n230 = Wait (ms)(milliseconds to wait=u32 10) -> ()  [unwired: 1 out]
                      n231 = Equal?(x=w319, y=w315) -> (x = y?=w318:bool)
                      n232 = case shown="False" w318 {
                        tunnel: [TRUE FALSE] -> w317
                        frame False {
                        }
                        frame True {
                        }
                      }
                    }
                    "AMCS_Profile" <- w313
                  }
                  frame #3 {
                    # "convert time per range bin to meters\nand calculate smoothed bins using\nsmoothing range"
                    # "Plotting online cross section and smoothed online data"
                    # "Calculate the bin by bin mean of the data"
                    # "Collect 'Integration Period (Seconds)' number\nof scalar data"
                    # "Reading, processing, and plotting the online data"
                    n233 = local read "Data Reads (number of loops)"() -> (w347:i32)
                    n234 = for {
                      N: w347 -> [_]
                      tunnel: [w368] -> w359 mode=indexing
                      tunnel: [w367] -> w322 mode=indexing
                      # "Scalar Data is retrieved from Global \nVariable that scaler.vi is writing to,"
                      n235 = global read "AMCS_Data.vi" "AMCS_Data"() -> (w371:u16[][])
                      n236 = disable-structure shown="Disabled" {
                        frame Disabled {
                          n237 = global read "Scalar_Data_3.vi" "Scalar Data 3"() -> ()  [unwired: 1 out]
                          n238 = global read "Scalar_Data.vi" "Scalar Data"() -> ()  [unwired: 1 out]
                        }
                        frame Enabled {
                        }
                      }
                      n239 = Index Array(array=w371, index (row) #1=0 ("index (row)"), index (row) #2=2 ("index (row)")) -> (element #1=w368:u16[], element #2=w367:u16[])  [unwired: 2 in]
                    }
                    n240 = Transpose 2D Array(2D array=w359) -> (transposed array=w363:u16[][])
                    n241 = Transpose 2D Array(2D array=w322) -> (transposed array=w345:u16[][])
                    n242 = for {
                      tunnel: w363 -> [w373] mode=indexing
                      tunnel: [w372] -> w364 mode=indexing
                      n243 = call-poly <vilib>:"Mean.vi"("X"=w373) -> ("mean"=w372:dbl)  [unwired: 1 out]
                    }
                    n244 = for {
                      tunnel: w345 -> [w366] mode=indexing
                      tunnel: [w365] -> w346 mode=indexing
                      n245 = call-poly <vilib>:"Mean.vi"("X"=w366) -> ("mean"=w365:dbl)  [unwired: 1 out]
                    }
                    n246 = local read "bins"() -> (w339:u32)
                    n247 = Array Subset(array=w364, index=1 ("dimension size"), length=w339) -> (w351:dbl[])
                    n248 = Array Subset(array=w346, index=1 ("dimension size"), length=w339) -> (w343:dbl[])
                    n249 = local read "background length"() -> (w329:i32)
                    n250 = local read "background start"() -> (w330:u32)
                    n251 = Array Size(array=w351) -> (size(s)=w348:i32)
                    n252 = Array Size(array=w343) -> (size(s)=w340:i32)
                    n253 = Initialize Array(1.0 ("element"), w348) -> (w350:dbl[])
                    n254 = Initialize Array(1.0 ("element"), w340) -> (w342:dbl[])
                    n255 = Multiply(x=w351, y=w350) -> (x*y=w352:dbl[])
                    "CH 0 Bin Readings" <- w352
                    n256 = Multiply(x=w343, y=w342) -> (x*y=w333:dbl[])
                    "CH 2 Bin Readings" <- w333
                    n257 = local read "Total DIAL Integration Time (Minutes)"() -> (w355:i32)
                    n258 = local read "Time Resolution Per Bin(ns)"() -> (w325:u32)
                    n259 = Array Subset(array=w352, index=w330, length=w329) -> (w361:dbl[])
                    n260 = Array Subset(array=w333, index=w330, length=w329) -> (w335:dbl[])
                    n261 = call-poly <vilib>:"Mean.vi"("X"=w361) -> ("mean"=w360:dbl)  [unwired: 1 out]
                    n262 = call-poly <vilib>:"Mean.vi"("X"=w335) -> ("mean"=w336:dbl)  [unwired: 1 out]
                    n263 = Divide(x=w355, y=w347) -> (x/y=w353:dbl)
                    n264 = local read "Index"() -> (w334:i32)
                    n265 = Subtract(x=w352, y=w360) -> (x-y=w357:dbl[])
                    n266 = Subtract(x=w333, y=w336) -> (x-y=w337:dbl[])
                    n267 = To Double Precision Float(number=w325) -> (double precision float=w326:dbl)
                    n268 = Multiply(x=w353, y=60.0) -> (x*y=w331:dbl)
                    n269 = Multiply(x=w326, y=0.15) -> (x*y=w328:dbl)
                    n270 = call "Ring Buffer CH2 rev2.vi"("Index"=w334, "Profiles to Average"=w331, "Input Array"=w337) -> ("AvgArray"=w338:dbl[])  [unwired: 7 in, 1 out]
                    n271 = call "Ring Buffer CH0 rev2.vi"("Index"=w334, "Profiles to Average"=w331, "Input Array"=w357) -> ("AvgArray"=w356:dbl[])  [unwired: 7 in, 1 out]
                    n272 = Divide(x="Smoothing Range", y=w328) -> (x/y=w323:dbl)
                    "Smoothed Bins" <- w323
                    n273 = call "Smooth Arrray.vi"("smooth size"=w323, "Raw Array"=w356) -> ("Smoothed Array"=→"CH0 (WV on) smoothed":dbl[])  [unwired: 9 in]
                    n274 = call "Smooth Arrray.vi"("smooth size"=w323, "Raw Array"=w338) -> ("Smoothed Array"=→"CH2 (molecular) smoothed":dbl[])  [unwired: 9 in]
                    n275 = disable-structure shown="Disabled" {
                      frame Disabled {
                        n276 = script code="format long;\ncounts=sum(Online);\nif counts >=0.5e6\ntime=time;\nelse\ntime=time\nend"() -> ()  [unwired: 3 in, 2 out]
                      }
                      frame Enabled {
                      }
                    }
                  }
                  frame #4 {
                    # "Toggling the Agiltron switch to the offline DBR seed laser"
                    n277 = disable-structure shown="Disabled" {
                      frame Disabled {
                        n278 = flat-sequence {
                          frame #0 {
                            # "Second one"
                            # "Command the switch to switch to position 2\ncorresponding to the offline DBR"
                            # "Hex string command \ncorrespond to offline"
                            n279 = VISA Write(VISA resource name="Switch Comm Port", write buffer="\u0001\u0012\u0000\u0001") -> ()  [unwired: 1 in, 3 out]
                          }
                        }
                      }
                      frame Enabled {
                      }
                    }
                  }
                  frame #5 {
                    # "Save the recently collected online data if 'Save Data?' is true"
                    n280 = case shown="True" "Save Data?" {
                      frame False {
                        # "'Save Data?' is false, do nothing"
                      }
                      frame True {
                        # "'Save Data?' is true, save onfline data to the Data Disk"
                        # "Write only one copy of data at this time"
                        # "Retrieve Julian Date"
                        n281 = local read "Readings"() -> (w379:T7)
                        n282 = local read "Time Resolution Per Bin(ns)"() -> (w387:u32)
                        n283 = Unbundle By Name(w379) -> ("WV OnLine TEC"=w378:dbl)
                        n284 = local read "Number of Accumulates"() -> (w385:u32)
                        n285 = Unbundle By Name(w379) -> ("HSRL TEC"=w377:dbl)
                        n286 = local read "WV Online Read (nm)"() -> (w380:dbl)
                        n287 = local write "DataOpen"(TRUE ("DataOpen")) -> ()
                        n288 = local read "Number of Bins"() -> (w386:u32)
                        n289 = local read "HSRL Read (nm)"() -> (w381:dbl)
                        n290 = local read "Online Pulse Energy"() -> (w408:dbl)
                        n291 = local read "CH 0 Bin Readings"() -> (w410:dbl[])
                        n292 = To Double Precision Float(number=w387) -> (double precision float=w382:dbl)
                        n293 = To Double Precision Float(number=w386) -> (double precision float=w383:dbl)
                        n294 = To Double Precision Float(number=w385) -> (double precision float=w384:dbl)
                        n295 = local read "CH 2 Bin Readings"() -> (w407:dbl[])
                        n296 = call "Julian_Date_2.vi"() -> ("Julian Date"=w409:dbl)  [unwired: 11 in]
                        n297 = Build Array (concatenate)(w409, w380, w378, w408, w382, w383, w384, w410) -> (w402:dbl[])
                        n298 = Build Array (concatenate)(w409, w381, w377, w408, w382, w383, w384, w407) -> (w392:dbl[])
                        n299 = local read "NF_On_Ref"() -> (w390:refnum<file>)
                        n300 = local read "FF_On_Ref"() -> (w406:refnum<file>)
                        n301 = local read "NF_On_Ptr"() -> (w391:i64)
                        n302 = local read "FF_On_Ptr"() -> (w405:i64)
                        n303 = Set File Position(offset (in bytes) (0)=w405, refnum=w406) -> (refnum out=w403:refnum<file>, error out=w400:errorcluster)  [unwired: 2 in]
                        n304 = Set File Position(offset (in bytes) (0)=w391, refnum=w390) -> (refnum out=w396:refnum<file>, error out=w394:errorcluster)  [unwired: 2 in]
                        n305 = Write to Binary File(file (use dialog)=w396, data=w392, error in=w394, 5:FALSE ("prepend array or string size? (T)")) -> (refnum out=w395:refnum<file>, error out=w393:errorcluster)  [unwired: 2 in, 1 out]
                        n306 = Write to Binary File(file (use dialog)=w403, data=w402, error in=w400, 5:FALSE ("prepend array or string size? (T)")) -> (refnum out=w401:refnum<file>, error out=w399:errorcluster)  [unwired: 2 in, 1 out]
                        n307 = Get File Position(4:w393, 7:w395) -> (2:w389:i64)  [unwired: 2 out]
                        n308 = Get File Position(4:w399, 7:w401) -> (2:w398:i64)  [unwired: 2 out]
                        n309 = local write "NF_On_Ptr"(w389) -> ()
                        n310 = local write "FF_On_Ptr"(w398) -> ()
                      }
                    }
                  }
                }
              }
              frame #3 {
                # "Frame 3: Read offline data, calculate aerosol data, and plot offline and normalized relative backscatter\nFrame 4:\nFrame 5: Save the offline data and related information"
                # "Frame 0: Read the offline wavelength and lock if necessary, Switch to online DBR\nFrame 1: Read the output power from the Newport power meter\nFrame 2: Wait 'Scalar Wait Time' for buffers to clear of online contiminated data"
                # "offline"
                n311 = stacked-sequence {
                  frame #0 {
                    # "Following Locking the Offline wavelength, check and lock the HSRL 780 nm wavelength"
                    # "Every 60 data collection cycles, read the offline DBR wavelength, and if outside of wavelength tolerance, adjust DBR current until within tolerance"
                    n312 = local read "L_Count"() -> (w412:i32)
                    n313 = Quotient & Remainder(x=w412, y=60.0) -> (x-y*floor(x/y)=w413:dbl)  [unwired: 1 out]
                    n314 = Equal To 0?(x=w413) -> (x = 0?=w411:bool)
                    n315 = case shown="True" w411 {
                      frame False {
                      }
                      frame True {
                        n316 = flat-sequence {
                          frame #0 {
                            n317 = while {
                              i -> [w418]
                              stop <- w416 stop-if-true
                              # "If WL difference is within tolerance, stop looping, and illuminate 'Wavelength Lock Offline' indicator"
                              # "Frame 2: Decrement DBR if above tolerance\nFrame 3: Increment DBR if below tolerance"
                              # "Frame 0: Read the wavelength from the wavemeter\nFrame 1: Calculate the difference between desired and actual wavelength"
                              # "Continue reading and adjusting offline DBR until within locking tolerance"
                              n318 = stacked-sequence {
                                tunnel: w418 -> [w420 _ _ _ _]
                                tunnel: [_ _ w434 _ _] -> w415
                                frame #0 {
                                n319 = Equal To 0?(x=w420) -> (x = 0?=w419:bool)
                                n320 = case shown="True" w419 {
                                frame False {
                                }
                                frame True {
                                # "Set the TSOA switch to\namplify the offline wavelength"
                                n321 = Build Array(TRUE ("Boolean")) -> (w422:bool[])
                                n322 = call-poly <vilib>:"DAQmx Write.vi"("task/channels in"=refnum<k21> "BristolWM", "data"=w422) -> ()  [unwired: 11 in, 3 out]
                                n323 = Wait (ms)(milliseconds to wait=u32 3200) -> ()  [unwired: 1 out]
                                }
                                }
                                }
                                frame #1 {
                                # "Reading the wavelength from the wavemeter"
                                n324 = flat-sequence {
                                tunnel: [w427] -> w426
                                tunnel: w426 -> [w430]
                                tunnel: [w429] -> w425
                                tunnel: w425 -> [w433]
                                frame #0 {
                                n325 = local read "Bristol In"() -> (w428:i32)
                                n326 = dll-call lib="C:/Users/H2ODial/Desktop/Shared Telescope WV DIAL Code/bristol/CLDevIface.dll" fn="CLOpenUSBSerialDevice"("commPort"=w428) -> ("return type"=w427:i32)  [unwired: 4 in, 2 out]
                                }
                                frame #1 {
                                n327 = dll-call lib="C:/Users/H2ODial/Desktop/Shared Telescope WV DIAL Code/bristol/CLDevIface.dll" fn="CLGetLambdaReading"("devHandle"=w430) -> ("return type"=→"WV Offline Read (nm)":dbl, "devHandle"=w429:i32)  [unwired: 3 in, 2 out]
                                }
                                frame #2 {
                                n328 = dll-call lib="C:/Users/H2ODial/Desktop/Shared Telescope WV DIAL Code/bristol/CLDevIface.dll" fn="CLCloseDevice"("commPort"=w433) -> ("return type"=w432:i32)  [unwired: 4 in, 2 out]
                                n329 = local write "Bristol Out"(w432) -> ()
                                }
                                }
                                }
                                frame #2 {
                                # "Calculating the difference between the actual and desired online wavelength"
                                n330 = local read "Offline_Tol"() -> (w436:dbl)
                                n331 = local read "WV Offline Read (nm)"() -> (w442:dbl)
                                n332 = Multiply(x=-1.0, y=w436) -> (x*y=w435:dbl)
                                n333 = Subtract(x=w442, y="WV Offline Set (nm)") -> (x-y=w438:dbl)
                                "Oflline_Diff" <- w438
                                n334 = Greater?(x=w438, y=w435) -> (0:w439:bool)
                                n335 = Less?(x=w438, y=w436) -> (x < y?=w440:bool)
                                n336 = And(x=w439, y=w440) -> (x .and. y?=w434:bool)
                                "WV Oflline Locked" <- w434
                                n337 = case shown="True" w434 {
                                frame False {
                                }
                                frame True {
                                # "Set the Wavemeter switch to\nthe HSRL wavelength"
                                n338 = Build Array(TRUE ("Boolean")) -> (w444:bool[])
                                n339 = call-poly <vilib>:"DAQmx Write.vi"("task/channels in"=refnum<k21> "HSRL_WV_switch", "data"=w444) -> ()  [unwired: 11 in, 3 out]
                                n340 = Wait (ms)(milliseconds to wait=u32 3200) -> ()  [unwired: 1 out]
                                }
                                }
                                }
                                frame #3 {
                                # "If the wavelength difference is greater that 0.0002 nm, decrement the \nDBR current by 0.01 mA"
                                n341 = local read "Oflline_Diff"() -> (w449:dbl)
                                n342 = Greater Or Equal?(x=w449, y="Offline_Tol") -> (x >= y?=w448:bool)
                                n343 = case shown="True" w448 {
                                frame False {
                                # "Wavelength difference is not greater than 0.0002 nm, do nothing"
                                }
                                frame True {
                                # "Generating a command string\nto decrement the current"
                                n344 = local read "Settings"() -> (w456:T6)
                                n345 = Unbundle By Name(w456) -> ("WV Offline TEC"=w454:dbl)
                                n346 = Subtract(x=w454, y="temp step size") -> (x-y=w453:dbl)
                                n347 = local read "Device In"() -> (w451:refnum<visa-resource-name>)
                                n348 = Bundle By Name(cluster=w456, "WV Offline TEC"=w453, "Module"=T12."WV Offline TEC") -> (w457:T6)
                                n349 = call "TL_Driver_v2.vi"("Device In"=w451, "Commands"=T9."SET", "Settings"=w457) -> ("Readings"=w458:T7)  [unwired: 9 in, 3 out]
                                n350 = local write "Settings"(w457) -> ()
                                n351 = local write "Readings"(w458) -> ()
                                }
                                }
                                }
                                frame #4 {
                                # "If WL difference is < 0.0002 nm, increment the DBR temperature"
                                n352 = local read "Oflline_Diff"() -> (w461:dbl)
                                n353 = Less Or Equal?(x=w461, y=-0.0001) -> (x <= y?=w459:bool)
                                n354 = case shown="True" w459 {
                                frame False {
                                # "WL difference is no <= to -0.0002 nm, do nothing"
                                }
                                frame True {
                                # "Generating a command string\nto decrement the current"
                                # "WL difference is less than 0.0002 nm,\nincrement the DBR current by 0.01 mA"
                                n355 = local read "Settings"() -> (w469:T6)
                                n356 = Unbundle By Name(w469) -> ("WV Offline TEC"=w467:dbl)
                                n357 = local read "temp step size"() -> (w463:dbl)
                                n358 = Add(x=w467, y=w463) -> (x+y=w466:dbl)
                                n359 = local read "Device In"() -> (w464:refnum<visa-resource-name>)
                                n360 = Bundle By Name(cluster=w469, "WV Offline TEC"=w466, "Module"=T12."WV Offline TEC") -> (w470:T6)
                                n361 = call "TL_Driver_v2.vi"("Device In"=w464, "Commands"=T9."SET", "Settings"=w470) -> ("Readings"=w468:T7)  [unwired: 9 in, 3 out]
                                n362 = local write "Settings"(w470) -> ()
                                n363 = local write "Readings"(w468) -> ()
                                }
                                }
                                }
                              }
                              n364 = Or(x=w415, y="Cancel Offline") -> (x .or. y?=w416:bool)
                            }
                          }
                          frame #1 {
                            n365 = while {
                              i -> [w474]
                              stop <- w472 stop-if-true
                              # "If WL difference is within tolerance, stop looping, and illuminate 'Wavelength Lock Offline' indicator"
                              # "Frame 2: Decrement DBR if above tolerance\nFrame 3: Increment DBR if below tolerance"
                              # "Frame 0: Read the wavelength from the wavemeter\nFrame 1: Calculate the difference between desired and actual wavelength"
                              # "Continue reading and adjusting offline DBR until within locking tolerance"
                              n366 = stacked-sequence {
                                tunnel: w474 -> [w476 _ _ _ _]
                                tunnel: [_ _ w489 _ _] -> w471
                                frame #0 {
                                n367 = Equal To 0?(x=w476) -> (x = 0?=w475:bool)
                                n368 = case shown="True" w475 {
                                frame False {
                                }
                                frame True {
                                # "Set the Wavemeter to\nthe non HSRL wavelength"
                                n369 = Build Array(TRUE ("Boolean")) -> (w477:bool[])
                                n370 = call-poly <vilib>:"DAQmx Write.vi"("task/channels in"=refnum<k21> "HSRL_WV_switch", "data"=w477) -> ()  [unwired: 11 in, 3 out]
                                }
                                }
                                }
                                frame #1 {
                                # "Reading the wavelength from the wavemeter"
                                n371 = flat-sequence {
                                tunnel: [w482] -> w481
                                tunnel: w481 -> [w485]
                                tunnel: [w484] -> w480
                                tunnel: w480 -> [w488]
                                frame #0 {
                                n372 = local read "Bristol In"() -> (w483:i32)
                                n373 = dll-call lib="C:/Users/H2ODial/Desktop/Shared Telescope WV DIAL Code/bristol/CLDevIface.dll" fn="CLOpenUSBSerialDevice"("commPort"=w483) -> ("return type"=w482:i32)  [unwired: 4 in, 2 out]
                                }
                                frame #1 {
                                n374 = dll-call lib="C:/Users/H2ODial/Desktop/Shared Telescope WV DIAL Code/bristol/CLDevIface.dll" fn="CLGetLambdaReading"("devHandle"=w485) -> ("return type"=→"HSRL Read (nm)":dbl, "devHandle"=w484:i32)  [unwired: 3 in, 2 out]
                                }
                                frame #2 {
                                n375 = dll-call lib="C:/Users/H2ODial/Desktop/Shared Telescope WV DIAL Code/bristol/CLDevIface.dll" fn="CLCloseDevice"("commPort"=w488) -> ("return type"=w487:i32)  [unwired: 4 in, 2 out]
                                n376 = local write "Bristol Out"(w487) -> ()
                                }
                                }
                                }
                                frame #2 {
                                # "Calculating the difference between the actual and desired online wavelength"
                                n377 = local read "HSRL_Tol"() -> (w491:dbl)
                                n378 = local read "HSRL Read (nm)"() -> (w497:dbl)
                                n379 = Multiply(x=-1.0, y=w491) -> (x*y=w490:dbl)
                                n380 = Subtract(x=w497, y="HSRL Set (nm)") -> (x-y=w493:dbl)
                                "HSRL_Diff" <- w493
                                n381 = Greater?(x=w493, y=w490) -> (0:w494:bool)
                                n382 = Less?(x=w493, y=w491) -> (x < y?=w495:bool)
                                n383 = And(x=w494, y=w495) -> (x .and. y?=w489:bool)
                                "HSRL Locked" <- w489
                                n384 = case shown="True" w489 {
                                frame False {
                                }
                                frame True {
                                # "Set the Wavementer switch to WV Online"
                                n385 = Build Array(FALSE ("Boolean")) -> (w499:bool[])
                                n386 = Build Array(FALSE ("Boolean")) -> (w503:bool[])
                                n387 = call-poly <vilib>:"DAQmx Write.vi"("task/channels in"=refnum<k21> "BristolWM", "data"=w503) -> ("error out"=w498:errorcluster)  [unwired: 11 in, 2 out]
                                n388 = call-poly <vilib>:"DAQmx Write.vi"("task/channels in"=refnum<k21> "HSRL_WV_switch", "data"=w499, "error in"=w498) -> ()  [unwired: 10 in, 3 out]
                                n389 = Wait (ms)(milliseconds to wait=u32 3200) -> ()  [unwired: 1 out]
                                }
                                }
                                }
                                frame #3 {
                                # "If the wavelength difference is greater that 0.0002 nm, decrement the \nDBR current by 0.01 mA"
                                n390 = local read "HSRL_Diff"() -> (w508:dbl)
                                n391 = Greater Or Equal?(x=w508, y="HSRL_Tol") -> (x >= y?=w507:bool)
                                n392 = case shown="True" w507 {
                                frame False {
                                # "Wavelength difference is not greater than 0.0002 nm, do nothing"
                                }
                                frame True {
                                # "Generating a command string\nto decrement the current"
                                n393 = local read "Settings"() -> (w515:T6)
                                n394 = local read "temp step size"() -> (w509:dbl)
                                n395 = Unbundle By Name(w515) -> ("HSRL TEC"=w514:dbl)
                                n396 = Subtract(x=w514, y=w509) -> (x-y=w513:dbl)
                                n397 = local read "Device In"() -> (w511:refnum<visa-resource-name>)
                                n398 = Bundle By Name(cluster=w515, "HSRL TEC"=w513, "Module"=T12."HSRL TEC") -> (w516:T6)
                                n399 = call "TL_Driver_v2.vi"("Device In"=w511, "Commands"=T9."SET", "Settings"=w516) -> ("Readings"=w517:T7)  [unwired: 9 in, 3 out]
                                n400 = local write "Settings"(w516) -> ()
                                n401 = local write "Readings"(w517) -> ()
                                }
                                }
                                }
                                frame #4 {
                                # "If WL difference is < 0.0002 nm, increment the DBR temperature"
                                n402 = local read "HSRL_Diff"() -> (w520:dbl)
                                n403 = Less Or Equal?(x=w520, y=-0.0001) -> (x <= y?=w518:bool)
                                n404 = case shown="True" w518 {
                                frame False {
                                # "WL difference is no <= to -0.0002 nm, do nothing"
                                }
                                frame True {
                                # "Generating a command string\nto decrement the current"
                                # "WL difference is less than 0.0002 nm,\nincrement the DBR current by 0.01 mA"
                                n405 = local read "Settings"() -> (w528:T6)
                                n406 = local read "temp step size"() -> (w521:dbl)
                                n407 = Unbundle By Name(w528) -> ("HSRL TEC"=w526:dbl)
                                n408 = Add(x=w526, y=w521) -> (x+y=w525:dbl)
                                n409 = local read "Device In"() -> (w523:refnum<visa-resource-name>)
                                n410 = Bundle By Name(cluster=w528, "HSRL TEC"=w525, "Module"=T12."HSRL TEC") -> (w529:T6)
                                n411 = call "TL_Driver_v2.vi"("Device In"=w523, "Commands"=T9."SET", "Settings"=w529) -> ("Readings"=w527:T7)  [unwired: 9 in, 3 out]
                                n412 = local write "Settings"(w529) -> ()
                                n413 = local write "Readings"(w527) -> ()
                                }
                                }
                                }
                              }
                              n414 = Or(x=w471, y="Cancel HSRL") -> (x .or. y?=w472:bool)
                            }
                          }
                        }
                      }
                    }
                  }
                  frame #1 {
                    # "Reading the power meter"
                    # "Updating the pulse energy plot"
                    # "Converting to pulse energy"
                    # "Reading the offline output power, converting to pulse energy,  and updating the Pulse energy plot"
                    n415 = local read "SampleSize"() -> (w532:i32)
                    n416 = local read "Newport Device Key"() -> (w533:string)
                    n417 = local read "Online Pulse Energy"() -> (w539:dbl)
                    n418 = local read "Offline Pulse Energy"() -> (w538:dbl)
                    n419 = local read "NewportRef"() -> (w530:refnum<k24>)
                    n420 = Number To Decimal String(number=w532) -> (decimal integer string=w534:string)  [unwired: 1 in]
                    n421 = invoke class="PowerMeterCommands" method="PerformDAQ"(reference=w530, "deviceKey"=w533, "interval"="1", "sampleSize"=w534) -> ("PerformDAQ"=w535:dbl[])  [unwired: 2 in, 5 out]
                    n422 = Bundle("Online Pulse Energy"=w539, "Offline Pulse Energy"=w538) -> (w537:T15)  [unwired: 1 in]
                    n423 = local write "Pulse Energy (Micro Joule)"(w537) -> ()
                    n424 = call-poly <vilib>:"Mean.vi"("X"=w535) -> ("mean"=w531:dbl)  [unwired: 1 out]
                    n425 = Multiply(x=w531, y=1000.0) -> (x*y=w544:dbl)
                    n426 = Divide(x=w544, y=0.05) -> (x/y=w542:dbl)
                    n427 = Divide(x=w542, y=7.0) -> (x/y=→"Offline Pulse Energy":dbl)
                  }
                  frame #2 {
                    # "Added in the ability to interactively control the ThorLab  setting (just etalon temp for now)"
                    # "Wait 'Scalar Wait Time' for buffers to clear of online contiminated offline data"
                    n428 = disable-structure shown="Disabled" {
                      frame Disabled {
                        # "Wait 'Scalar Wait Time'"
                        n429 = local read "Scalar Wait Time"() -> (w561:u32)
                        n430 = Wait (ms)(milliseconds to wait=w561) -> ()  [unwired: 1 out]
                      }
                      frame Enabled {
                      }
                    }
                    n431 = event shown="[2] \"Settings.HSRL Etalon TEC\": Value Change" {
                      selector: _ -> [_ _ _]
                      dyn-events: _ -> [_ _ _]
                      timeout: 1 -> [_ _ _]
                      event Timeout {
                        n432 = event-data() -> ()  [unwired: 1 in, 2 out]
                      }
                      event "Settings.WV Etalon TEC": Value Change {
                        # "Generating a command string\nto update the etalon"
                        n433 = event-data() -> ()  [unwired: 1 in, 5 out]
                        n434 = local read "Settings"() -> (w551:T6)
                        n435 = Unbundle By Name(w551) -> ("WV Etalon TEC"=w553:dbl)
                        n436 = local read "Device In"() -> (w547:refnum<visa-resource-name>)
                        n437 = Bundle By Name(cluster=w551, "WV Etalon TEC"=w553, "Module"=T12."WV Etalon TEC") -> (w549:T6)
                        n438 = call "TL_Driver_v2.vi"("Device In"=w547, "Commands"=T9."SET", "Settings"=w549) -> ("Readings"=w550:T7)  [unwired: 9 in, 3 out]
                        n439 = local write "Readings"(w550) -> ()
                        n440 = local write "Settings"(w549) -> ()
                      }
                      event "Settings.HSRL Etalon TEC": Value Change {
                        # "Generating a command string\nto update the etalon"
                        n441 = event-data() -> ()  [unwired: 1 in, 5 out]
                        n442 = local read "Settings"() -> (w558:T6)
                        n443 = Unbundle By Name(w558) -> ("HSRL Etalon TEC"=w560:dbl)
                        n444 = local read "Device In"() -> (w554:refnum<visa-resource-name>)
                        n445 = Bundle By Name(cluster=w558, "HSRL Etalon TEC"=w560, "Module"=T12."HSRL Etalon TEC") -> (w556:T6)
                        n446 = call "TL_Driver_v2.vi"("Device In"=w554, "Commands"=T9."SET", "Settings"=w556) -> ("Readings"=w557:T7)  [unwired: 9 in, 3 out]
                        n447 = local write "Readings"(w557) -> ()
                        n448 = local write "Settings"(w556) -> ()
                      }
                    }
                  }
                  frame #3 {
                    w590 = 1 ("dimension size")
                    # "Read in latest scalar card data from \n'Scalar Data' global variable that \nscaler.vi is writing to, then wait 1 sec\nfor next batch of data"
                    # "Calculating/Plotting smoothed data,\ncross sections etc."
                    # "Pick off data with\nout header"
                    # "Calculate mean bin by bin mean"
                    # "Reading in 'Integration Period (Seconds)' of data"
                    # "Read the offline data from the scalar card, perform smoothing, calculate normalized relative backscatter, and plot"
                    # "Collects Data From Card,\nSends It To The Chart,\nAnd Saves A Copy As A\nFile If Option Selected On\nFront Panel"
                    n449 = for {
                      N: "Data Reads (number of loops)" -> [_]
                      tunnel: [w648] -> w579 mode=indexing
                      tunnel: [w647] -> w578 mode=indexing
                      n450 = global read "AMCS_Data.vi" "AMCS_Data"() -> (w649:u16[][])
                      n451 = disable-structure shown="Disabled" {
                        frame Disabled {
                          n452 = global read "Scalar_Data_4.vi" "Scalar Data 4"() -> ()  [unwired: 1 out]
                          n453 = global read "Scalar_Data_2.vi" "Scalar Data 2"() -> ()  [unwired: 1 out]
                        }
                        frame Enabled {
                        }
                      }
                      n454 = Index Array(array=w649, index (row) #1=1 ("index (row)"), index (row) #2=3 ("index (row)")) -> (element #1=w648:u16[], element #2=w647:u16[])  [unwired: 2 in]
                    }
                    n455 = local read "Total DIAL Integration Time (Minutes)"() -> (w610:i32)
                    n456 = Divide(x=w610, y="Data Reads (number of loops)") -> (x/y=w608:dbl)
                    n457 = local read "Total Aerosol Integration Time (Minutes)"() -> (w612:dbl)
                    n458 = Multiply(x=w608, y=60.0) -> (x*y=w596:dbl)
                    n459 = local read "background length"() -> (w583:i32)
                    n460 = local read "background start"() -> (w584:u32)
                    n461 = Transpose 2D Array(2D array=w579) -> (transposed array=w618:u16[][])
                    n462 = Transpose 2D Array(2D array=w578) -> (transposed array=w602:u16[][])
                    n463 = Divide(x=w612, y="Data Reads (number of loops)") -> (x/y=w613:dbl)
                    n464 = for {
                      tunnel: w618 -> [w655] mode=indexing
                      tunnel: [w654] -> w619 mode=indexing
                      tunnel: w602 -> [w653] mode=indexing
                      tunnel: [w652] -> _ mode=indexing
                      tunnel: [w652] -> w599 mode=indexing
                      n465 = call-poly <vilib>:"Mean.vi"("X"=w655) -> ("mean"=w654:dbl)  [unwired: 1 out]
                      n466 = call-poly <vilib>:"Mean.vi"("X"=w653) -> ("mean"=w652:dbl)  [unwired: 1 out]
                    }
                    n467 = local read "bins"() -> (w591:u32)
                    n468 = Multiply(x=w613, y=60.0) -> (x*y=w575:dbl)
                    n469 = Array Subset(array=w599, index=w590, length=w591) -> (w600:dbl[])
                    "CH3 Bin Readings" <- w600
                    n470 = Array Subset(array=w619, index=w590, length=w591) -> (w598:dbl[])
                    "CH1  Bin Readings" <- w598
                    n471 = Array Subset(array=w600, index=w584, length=w583) -> (w601:dbl[])
                    n472 = Array Subset(array=w598, index=w584, length=w583) -> (w617:dbl[])
                    n473 = local read "Smoothed Bins"() -> (w580:dbl)
                    n474 = call-poly <vilib>:"Mean.vi"("X"=w601) -> ("mean"=w565:dbl)  [unwired: 1 out]
                    n475 = call-poly <vilib>:"Mean.vi"("X"=w617) -> ("mean"=w570:dbl)  [unwired: 1 out]
                    n476 = local read "Index"() -> (w576:i32)
                    n477 = Subtract(x=w600, y=w565) -> (x-y=w577:dbl[])
                    n478 = Subtract(x=w598, y=w570) -> (x-y=w594:dbl[])
                    n479 = call "Ring Buffer CH1 short rev2.vi"("Index"=w576, "Profiles to Average"=w596, "Input Array"=w594) -> ("AvgArray"=w615:dbl[], "RingBufferOut"=→"CH1 RingBuffer long":dbl[][])  [unwired: 7 in]
                    n480 = call "Ring Buffer CH1 long rev2.vi"("Index"=w576, "Profiles to Average"=w575, "Input Array"=w594) -> ("AvgArray"=w611:dbl[], "RingBufferOut"=→"CH1 RingBuffer short":dbl[][])  [unwired: 7 in]
                    n481 = call "Ring Buffer CH3 long rev2.vi"("Index"=w576, "Profiles to Average"=w596, "Input Array"=w577) -> ("AvgArray"=w597:dbl[], "RingBufferOut"=→"CH3 RingBuffer long":dbl[][])  [unwired: 7 in]
                    n482 = call "Ring Buffer CH3 short rev2.vi"("Index"=w576, "Profiles to Average"=w575, "Input Array"=w577) -> ("AvgArray"=w587:dbl[], "RingBufferOut"=→"CH3 RingBuffer short":dbl[][])  [unwired: 7 in]
                    n483 = Reshape Array(w594, w590, w591) -> (→"CH 1 (WV off) counts display":dbl[][])
                    n484 = Reshape Array(w577, w590, w591) -> (→"CH 3 (HSRL comb) counts display":dbl[][])
                    n485 = local read "Time Resolution Per Bin(ns)"() -> (w566:u32)
                    n486 = local read "Number of Accumulates"() -> (w564:u32)
                    n487 = call "Smooth Arrray.vi"("smooth size"=w580, "Raw Array"=w615) -> ("Smoothed Array"=→"CH1 (WV off) smooth S":dbl[])  [unwired: 9 in]
                    n488 = call "Smooth Arrray.vi"("smooth size"=w580, "Raw Array"=w611) -> ("Smoothed Array"=w589:dbl[])  [unwired: 9 in]
                    "CH1 (WV off) smooth L" <- w589
                    n489 = call "Smooth Arrray.vi"("smooth size"=w580, "Raw Array"=w597) -> ("Smoothed Array"=→"CH3 (HSRL combined) smooth L":dbl[])  [unwired: 9 in]
                    n490 = call "Smooth Arrray.vi"("smooth size"=w580, "Raw Array"=w587) -> ("Smoothed Array"=w582:dbl[])  [unwired: 9 in]
                    "CH3 (HSRL combined) smooth S" <- w582
                    n491 = local read "Temperature (C)"() -> (w607:dbl)
                    n492 = local read "Pressure (mb)"() -> (w606:dbl)
                    n493 = To Double Precision Float(number=w564) -> (double precision float=w563:dbl)
                    n494 = To Double Precision Float(number=w566) -> (double precision float=w562:dbl)
                    n495 = Reciprocal(x=w562) -> (1/x=w573:dbl)
                    n496 = disable-structure shown="Enabled" {
                      disable-tunnel: w607 -> [w646 _]
                      disable-tunnel: w606 -> [w645 _]
                      disable-tunnel: w589 -> [w639 _]
                      disable-tunnel: w570 -> [w626 _]
                      disable-tunnel: w565 -> [w625 _]
                      disable-tunnel: w563 -> [w624 _]
                      disable-tunnel: "dead time" -> [w623 _]
                      disable-tunnel: w582 -> [w622 _]
                      disable-tunnel: 6.0 ("Real") -> [w621 _]
                      disable-tunnel: w562 -> [w620 _]
                      frame Enabled {
                        w642 = 1
                        # "Plotting the normalized relative \nbackscatter"
                        # "Calculating the normalized relative backscatter"
                        # "File path in MATLAB script is of old dial is:\nF:\\Micropulse DIAL\\Micropulse DIAL Matlab\\\nFinal Overlap Function.mat')];"
                        n497 = script code="%accum_num=10000;     % scaler card setting number of accumulations\nt_bin = t_bin_in/1e9                 % scaler card setting time per bin\n%t_d = 37.3e-9;                % APD dead time from spec sheet\n\n% conversion from accumulated counts to count rate  (c/s)\nc_convert = 1./t_bin./accum_num;\nCR_far = p_raw_far.*c_convert;\nCR_near = p_raw_near.*c_convert;\nCR_total_far = (p_raw_far+b_far).*c_convert;\nCR_total_near = (p_raw_near+b_near).*c_convert;\nb_CR_far =b_far.*c_convert;\nb_CR_near =b_near.*c_convert;\n \n% create a range array\nsize_p =  size(p_raw_far,2);\ngate = t_bin*3e8/2;\nr = (gate:gate:size_p*gate)./1e3; \n   \n%APD correction factor\n D_far = 1./(1-(t_d*CR_total_far));\n D_near = 1./(1-(t_d*CR_total_near));\n\n %Calculating normalize relative backscatter profile\n nrb_far = CR_far.*D_far.*r.^2.*1e-6;\n nrb_near = CR_near.*D_near.*r.^2.*1e-6;"("E"=w621, "temp"=w646, "press"=w645, "p_raw_far"=w639, "b_far"=w626, "b_near"=w625, "p_raw_near"=w622, "accum_num"=w624, "t_d"=w623, "t_bin_in"=w620) -> ("nrb_far"=w634:cdb[], "D_far"=w631:dbl[], "nrb_near"=w633:cdb[], "D_near"=w630:dbl[])  [unwired: 1 in, 1 out]
                        n498 = local read "bins"() -> (w641:u32)
                        n499 = local read "Altitude Array (km)"() -> (w636:dbl[])
                        n500 = Build Array(w634, w633) -> (w638:cdb[][])
                        n501 = Build Array(w631, w630) -> (w629:dbl[][])
                        n502 = Reshape Array(w633, w642, w641) -> (→"NRB HSRL Combined":cdb[][])
                        n503 = Reshape Array(w634, w642, w641) -> (→"NRB WV Offline":cdb[][])
                        n504 = Build Array(w636, w636) -> (w635:dbl[][])
                        n505 = call "Convert to Dynamic Data7"("2D Array"=w629) -> ("Dynamic Data Type"=w628:dynamicdata)  [unwired: 3 in]
                        n506 = call "Convert to Dynamic Data3"("2D Array"=w638) -> ("Dynamic Data Type"=w637:dynamicdata)  [unwired: 3 in]
                        n507 = call "Convert to Dynamic Data4"("2D Array"=w635) -> ("Dynamic Data Type"=w632:dynamicdata)  [unwired: 3 in]
                        n508 = call "Build XY Graph2"("Y Input"=w632, "X Input"=w637) -> ("XY Graph"=→"NRB plot":cluster{"Y":dbl[], "Y":dbl[]}[])  [unwired: 3 in, 6 out]
                        n509 = call "Build XY Graph4"("Y Input"=w632, "X Input"=w628) -> ("XY Graph"=→"Correction":cluster{"Y":dbl[], "Y":dbl[]}[])  [unwired: 3 in, 6 out]
                      }
                      frame Disabled {
                      }
                    }
                    n510 = Divide(x=w573, y=w563) -> (x/y=w571:dbl)
                    n511 = Multiply(x=1000000000.0, y=w571) -> (x*y=w568:dbl)
                    n512 = Multiply(x=w568, y=w570) -> (x*y=w569:dbl)
                    n513 = Multiply(x=w568, y=w565) -> (x*y=w567:dbl)
                    n514 = Bundle(w569, w567) -> (→"?":cluster{dbl, dbl})  [unwired: 1 in]
                  }
                  frame #4 {
                    # "REPLACE WITH NEW AGILTRON TASK!"
                    # "Toggle Agiltron switch to online DBR"
                    n515 = disable-structure shown="Disabled" {
                      frame Disabled {
                        # "ABSORBING"
                        n516 = flat-sequence {
                          frame #0 {
                            # "Third one"
                            # "Command the switch to switch to position 1\ncorresponding to the online DBR"
                            # "Hex string command \ncorrespond to online"
                            n517 = local read "Switch Comm Port"() -> (w659:refnum<visa-resource-name>)
                            n518 = VISA Write(VISA resource name=w659, write buffer="\u0001\u0012\u0000\u0002") -> ()  [unwired: 1 in, 3 out]
                          }
                        }
                        n519 = Build Array(FALSE ("Boolean")) -> (w658:bool[])
                        n520 = call-poly <vilib>:"DAQmx Write.vi"("task/channels in"=refnum<k21> "AgiltronSwitch", "data"=w658) -> ()  [unwired: 11 in, 3 out]
                      }
                      frame Enabled {
                      }
                    }
                  }
                  frame #5 {
                    # "If 'Save Data?' is true, save all relavant offline info"
                    n521 = local read "Save Data?"() -> (w661:bool)
                    n522 = case shown="True" w661 {
                      frame False {
                        # "'Save Data?' is false, do nothing"
                      }
                      frame True {
                        # "Write only one data file at this time"
                        # "Retrive Julian Date"
                        # "'Save Data?' is true, save offline data to the Data Disk"
                        n523 = local read "Readings"() -> (w662:T7)
                        n524 = Unbundle By Name(w662) -> ("WV Offline TEC"=w663:dbl)
                        n525 = Unbundle By Name(w662) -> ("HSRL TEC"=w664:dbl)
                        n526 = local read "HSRL Read (nm)"() -> (w665:dbl)
                        n527 = local read "WV Offline Read (nm)"() -> (w686:dbl)
                        n528 = local read "Relative Humdity (%)"() -> (w690:dbl)
                        n529 = local read "CH3 Bin Readings"() -> (w684:dbl[])
                        n530 = local read "CH1  Bin Readings"() -> (w691:dbl[])
                        n531 = local read "Offline Pulse Energy"() -> (w687:dbl)
                        n532 = local read "Temperature (C)"() -> (w688:dbl)
                        n533 = local read "Pressure (mb)"() -> (w689:dbl)
                        n534 = call "Julian_Date_2.vi"() -> ("Julian Date"=w685:dbl)  [unwired: 11 in]
                        n535 = Build Array (concatenate)(w685, w686, w663, w687, w688, w689, w690, w691) -> (w670:dbl[])
                        n536 = Build Array (concatenate)(w685, w665, w664, w687, w688, w689, w690, w684) -> (w667:dbl[])
                        n537 = local read "FF_Off_Ref"() -> (w672:refnum<file>)
                        n538 = local read "NF_Off_Ref"() -> (w669:refnum<file>)
                        n539 = local read "FF_Off_Ptr"() -> (w671:i64)
                        n540 = local read "NF_Off_Ptr"() -> (w668:i64)
                        n541 = Set File Position(offset (in bytes) (0)=w671, refnum=w672) -> (refnum out=w683:refnum<file>, error out=w681:errorcluster)  [unwired: 2 in]
                        n542 = Set File Position(offset (in bytes) (0)=w668, refnum=w669) -> (refnum out=w679:refnum<file>, error out=w677:errorcluster)  [unwired: 2 in]
                        n543 = Write to Binary File(file (use dialog)=w683, data=w670, error in=w681, 5:FALSE ("prepend array or string size? (T)")) -> (refnum out=w682:refnum<file>, error out=w680:errorcluster)  [unwired: 2 in, 1 out]
                        n544 = Write to Binary File(file (use dialog)=w679, data=w667, error in=w677, 5:FALSE ("prepend array or string size? (T)")) -> (refnum out=w678:refnum<file>, error out=w676:errorcluster)  [unwired: 2 in, 1 out]
                        n545 = Get File Position(4:w680, 7:w682) -> (2:w673:i64)  [unwired: 2 out]
                        n546 = Get File Position(4:w676, 7:w678) -> (2:w666:i64)  [unwired: 2 out]
                        n547 = local write "FF_Off_Ptr"(w673) -> ()
                        n548 = local write "NF_Off_Ptr"(w666) -> ()
                      }
                    }
                  }
                }
              }
              frame #4 {
                n549 = First Call?() -> (First Call?: T/F=w694:bool)
                n550 = Or(x="calculate absorption cross sections", y=w694) -> (x .or. y?=w692:bool)
                n551 = case shown="True" w692 {
                  frame False {
                  }
                  frame True {
                    # "calculate absorption cross sections from HITRAN data base"
                    n552 = local read "WV Offline Set (nm)"() -> (w697:dbl)
                    n553 = local read "CH1 (WV off) smooth S"() -> (w701:dbl[])
                    n554 = local read "WV Online Read (nm)"() -> (w700:dbl)
                    n555 = local read "Temperature (C)"() -> (w699:dbl)
                    n556 = local read "Pressure (mb)"() -> (w698:dbl)
                    n557 = script code="hitran = dlmread('C:\\Users\\H2ODial\\Desktop\\Shared Telescope WV DIAL Code\\Libraries and VIs\\815nm_841nm_HITRAN_2008.csv', ',',[1 1 1676 8]);\n%hitran = dlmread('C:\\Users\\H2ODial\\Desktop\\Shared Telescope WV DIAL Code\\Libraries and VIs\\824nm_841nm_H2O.csv', ',',[0 1 352 7]);\n%hitran = dlmread('C:\\Users\\H2ODial\\Desktop\\Shared Telescope WV DIAL Code\\Libraries and VIs\\824nm_841nm_H2O_Spectral_Calc.csv', ',',[1 1 1209 7]);\n\n%Range vector in meters\nrange = ([75:75:size(Online,2)*75]);\n\nif lambda< 828\nlambda=828.195;\nelse\nlambda=lambda;\nend;\n\n%%\n\n%Voigt profile calculation\nWNmin = 1/(828+4)*1e7;  % 832.0 nm converted to wavenumber\nWNmax = 1/(828-4)*1e7;  % 824.0 nm converted to wavenumber\n\n%Find lines from WNmin to WNmax to calculate voigt profile\nline_indices = hitran(1:size(hitran,1),1)>WNmin & hitran(1:size(hitran,1),1)<WNmax;\n\nline = double(hitran(line_indices, 1:size(hitran,2)));\n\n%Calculate temperature and pressure profile\nT0 = 273+25; % surface temperature\nT0 = 273+T0_C;\nT = T0-0.0065.*range; % set to match the sounding\n\n% pressure in atmospheres\nP0  = 0.83; % surface pressure\nP0  = P0_mb/1000*0.986; %pressure in mb converted to atm\nP = P0.*(T0./T).^-5.5;   % set this value to match sounding\n\nT00 = 296;              % HITRAN reference temperature [K]\nP00 = 1;                % HITRAN reference pressure [atm]\nnu0_0 = line(:,1);      % absorption line center wavenumber from HITRAN [cm^-1]\nS0 = line(:,2);         % initial linestrength from HITRAN [cm^-1/(mol*cm^-2)]   \ngammal0 = line(:,4);    % air-broadened halfwidth at T_ref and P_ref from HITRAN [cm^-1/atm]\ngamma_s = line(:,5);    % self-broadened halfwidth at T_ref and P_ref from HITRAN [cm^-1/atm]\nE = line(:,6);          % ground state transition energy from HITRAN [cm^-1]  \nalpha = line(:,7);      % linewidth temperature dependence factor from HITRAN\ndelta = line(:,8);      % pressure shift from HiTRAN [cm^-1 atm^-1]\n\nnu_on = 1/(lambda)*1e7;\nnu_off = 1/(lambda_off)*1e7;\n\nfor i = 1:size(Online,2); % calculate the absorption cross section at each range\n  \n    nu0 = nu0_0+delta.*(P(i)./P00); % unclear if it should be Pi/P00  \n    gammal = gammal0.*(P(i)./P00).*((T00./T(i)).^alpha);    %Calculate Lorentz lineweidth at P(i) and T(i)\n\n    const.m = 18.015E-3./6.022E23; % mass of a single water molecule\n    const.k_B = 1.3806488e-23; % (J/K)\n    const.c = 299792458; % (m/s) (exact)\n \n    gammad = (nu0).*((2.0.*const.k_B.*T(i).*log(2.0))./(const.m.*const.c^2)).^(0.5);  %Calculate HWHM Doppler linewidth at T(i)\n     \n    % term 1 in the Voigt profile\n    y = (gammal./gammad).*((log(2.0)).^(0.5));\n    \n    % term 2 in the Voigt profile\n    x_on = ((nu_on-nu0)./gammad).*(log(2.0)).^(0.5);\n    x_off = ((nu_off-nu0)./gammad).*(log(2.0)).^(0.5);\n    \n    %setting up Voigt convolution\n    t = (-(size(line,1))/2:1:size(line,1)/2-1); %set up the integration spectral step size\n    t = repmat(t',1,length(x_on))';\n    x_on = repmat(x_on,1,length(t));\n    x_off = repmat(x_off,1,length(t));\n    y = repmat(y,1,length(t));\n    f_on = (exp(-t.^2.0))./(y.^2.0+(x_on-t).^2.0);  % combined Voigt term 1 and 2\n    f_off = (exp(-t.^2.0))./(y.^2.0+(x_off-t).^2.0);\n    %Voigt integration over all of the lines at the on and offline locations\n    z_on = trapz(t(1,:),f_on,2);\n    z_off =  trapz(t(1,:),f_off,2);\n    integral_on = z_on;\n    integral_off = z_off;\n    %Calculate linestrength at temperature T\n    S = S0.*((T00./T(i)).^(1.5)).*exp(1.439.*E.*((1./T00)-(1./T(i))));\n \n    %Calculate the Voigt profile\n    K_on = (y(:,1)./pi).*integral_on;\n    K_off = (y(:,1)./pi).*integral_off;\n    \n    %Calculate the Voigt profile absorption cross section [cm^2]\n    sigmav_on = S.*(1./gammad).*(((log(2.0))./pi).^(0.5)).*K_on; %.*far_wing_on;\n    sigmav_off = S.*(1./gammad).*(((log(2.0))./pi).^(0.5)).*K_off; %.*far_wing_off;\n    \n    %Sum contributions from all of the surrounding lines\n    sigma_on_total(i) = sum(sigmav_on);\n    sigma_off_total(i) = sum(sigmav_off);\n    \nend;"("lambda"=w700, "lambda_off"=w697, "P0_mb"=w698, "T0_C"=w699, "Online"=w701) -> ("sigma_on_total"=→"sigma_on_total":dbl[], "sigma_off_total"=→"sigma_off_total":dbl[])  [unwired: 1 in, 1 out]
                  }
                }
              }
              frame #5 {
                # "new rainbow color bar display"
                # "new rainbow color bar display"
                # "normalization factor\nfrom 300 to 450m"
                # "OPTICAL DEPTH PLOT"
                # "Data Processing Far Channel"
                # "Calculating the range resolved water vapor number density and plotting"
                n558 = local read "CH3 (HSRL combined) smooth L"() -> (w743:dbl[])
                n559 = local read "CH2 (molecular) smoothed"() -> (w742:dbl[])
                n560 = local read "CH0 (WV on) smoothed"() -> (w722:dbl[])
                n561 = local read "CH1 (WV off) smooth S"() -> (w721:dbl[])
                n562 = local read "sigma_on_total"() -> (w744:dbl[])
                n563 = local read "sigma_off_total"() -> (w745:dbl[])
                n564 = local read "gate size"() -> (w702:dbl)
                n565 = script code="%Time averaging in seconds.  600 Seconds =10 minutes\ntemporal_average = 600;\n\n%Spatial averaging in bins.  2 bins = 150 meters\nspatial_average = 2;\n\n%Creating r and r+deltar vectors..this can also be acsomplished using the\n%diff command\np_oni = Online(:,1:size(Online,2)-1);\n\np_onii = Online(:,2:size(Online,2));\n\np_offi = Offline(:,1:size(Offline,2)-1);\n\np_offii = Offline(:,2:size(Offline,2));\n\nInside = (p_oni.*p_offii)./(p_onii.*p_offi);\n\ndel_cross = 1./(2.*(sigma_on_total(1:size(Online,2)-1)-sigma_off_total(1:size(Offline,2)-1)).*75*100);\n\ndel_cross(isinf(del_cross)) = 0;\n\n%Calculating Number density\nN = del_cross.*log(Inside);\n\n%Spatial smoothing of the profiles\nfilter1 = ones(1,2)./2;\n\nN_1 = N;\n\nN_1_avg = filter2(filter1,N_1);\n\nfilter1 = ones(1,10)./10;\n\nN_2 = N;\n\nN_2_avg = filter2(filter1,N_2);\n\nN_new = zeros(size(N,1),size(N,2));\n \n%Using different averaging windows for different altitudes \nN_avg=[N_1_avg(:,1:40)';N_2_avg(:,41:size(N,2))']';\n\n\nw = N_avg.*1e6.*18.015./6.022e23"("Online"=w742, "Offline"=w743, "sigma_on_total"=w744, "sigma_off_total"=w745) -> ()  [unwired: 1 in, 3 out]
                n566 = script code="%Time averaging in seconds.  600 Seconds =10 minutes\ntemporal_average = 600;\n%Spatial averaging in bins.  150 meters\nspatial_average = 150./gate_size;\n%Creating r and r+deltar vectors..this can also be acsomplished using the\n%diff command\np_oni = Online(:,1:size(Online,2)-1);\np_onii = Online(:,2:size(Online,2));\np_offi = Offline(:,1:size(Offline,2)-1);\np_offii = Offline(:,2:size(Offline,2));\nInside = (p_oni.*p_offii)./(p_onii.*p_offi);\ndel_cross = 1./(2.*(sigma_on_total(1:size(Online,2)-1)-sigma_off_total(1:size(Offline,2)-1)).*gate_size*100);\ndel_cross(isinf(del_cross)) = 0;\n%Calculating Number density\nN = del_cross.*log(Inside);\n%Spatial smoothing of the profiles\nfilter1 = ones(1,4)./4;\nN_1 = N;\nN_1_avg = filter2(filter1,N_1);\nfilter1 = ones(1,10)./10;\nN_2 = N;\nN_2_avg = filter2(filter1,N_2);\nN_new = zeros(size(N,1),size(N,2));\n%Using different averaging windows for different altitudes \nN_avg=[N_1_avg(:,1:40)';N_2_avg(:,41:size(N,2))']';\nw = N_avg.*1e6.*18.015./6.022e23"("Online"=w722, "Offline"=w721, "sigma_on_total"=w744, "sigma_off_total"=w745, "gate_size"=w702) -> ("N_avg"=w704:cdb[], "w"=w705:cdb[])  [unwired: 1 in, 1 out]
                n567 = local read "Time Resolution Per Bin(ns)"() -> (w720:u32)
                n568 = local read "Number of Bins"() -> (w711:u32)
                n569 = local read "Altitude Array (km)"() -> (w708:dbl[])
                n570 = Reshape Array(w705, 1, w711) -> (→"Absolute Humdity":cdb[][])
                n571 = To Double Precision Float(number=w720) -> (double precision float=w741:dbl)
                n572 = call "Convert to Dynamic Data9"("Array"=w704) -> ("Dynamic Data Type"=w709:dynamicdata)  [unwired: 3 in]
                n573 = call "Convert to Dynamic Data6"("Array"=w705) -> ("Dynamic Data Type"=w706:dynamicdata)  [unwired: 3 in]
                n574 = Multiply(x=0.15, y=w741) -> (x*y=w739:dbl)
                n575 = call "Convert to Dynamic Data8"("Array"=w708) -> ("Dynamic Data Type"=w710:dynamicdata)  [unwired: 3 in]
                n576 = call "Convert to Dynamic Data5"("Array"=w708) -> ("Dynamic Data Type"=w707:dynamicdata)  [unwired: 3 in]
                n577 = call "Build XY Graph"("Y Input"=w710, "X Input"=w709) -> ("XY Graph"=→"Water Vapor Number Density":cluster{"Y":dbl[], "Y":dbl[]}[])  [unwired: 3 in, 6 out]
                n578 = call "Build XY Graph3"("Y Input"=w707, "X Input"=w706) -> ("XY Graph"=→"Absolute Humidity":cluster{"Y":dbl[], "Y":dbl[]}[])  [unwired: 3 in, 6 out]
                n579 = Divide(x=300.0, y=w739) -> (x/y=w736:dbl)
                n580 = Divide(x=450.0, y=w739) -> (x/y=w735:dbl)
                n581 = To Long Integer(number=w736) -> (32bit integer=w734:i32)
                n582 = To Long Integer(number=w735) -> (32bit integer=w733:i32)
                n583 = Decrement(x=w734) -> (x-1=w731:i32)
                n584 = Decrement(x=w733) -> (x-1=w732:i32)
                n585 = Array Subset(array=w722, index=w731, length=w732) -> (w730:dbl[])
                n586 = Array Subset(array=w721, index=w731, length=w732) -> (w729:dbl[])
                n587 = call-poly <vilib>:"Mean.vi"("X"=w730) -> ("mean"=w728:dbl)  [unwired: 1 out]
                n588 = call-poly <vilib>:"Mean.vi"("X"=w729) -> ("mean"=w727:dbl)  [unwired: 1 out]
                n589 = Divide(x=w728, y=w727) -> (x/y=w726:dbl)
                n590 = Multiply(x=w721, y=w726) -> (x*y=w725:dbl[])
                n591 = Divide(x=w722, y=w725) -> (x/y=w724:dbl[])
                n592 = Natural Logarithm(1:w724) -> (0:w723:dbl[])
                n593 = Multiply(x=-1.0, y=w723) -> (x*y=w717:dbl[])
                n594 = call "Convert to Dynamic Data"("Array"=w717) -> ("Dynamic Data Type"=w719:dynamicdata)  [unwired: 3 in]
                n595 = call "Convert to Dynamic Data2"("Array"=w708) -> ("Dynamic Data Type"=w716:dynamicdata)  [unwired: 3 in]
                n596 = call "Build OD Plot"("Y Input"=w716, "X Input"=w719) -> ("XY Graph"=→"Optical Depth":cluster{"Y":dbl[], "Y":dbl[]}[])  [unwired: 3 in, 6 out]
              }
            }
          }
        }
        "L_Count" <- w129
      }
    }
  }
  n597 = case shown="True" w3 {
    frame False {
    }
    frame True {
      # "close data files"
      n598 = local read "NF_Off_Ref"() -> (w747:refnum<file>)
      n599 = local read "NF_On_Ref"() -> (w748:refnum<file>)
      n600 = local read "FF_Off_Ref"() -> (w749:refnum<file>)
      n601 = local read "FF_On_Ref"() -> (w750:refnum<file>)
      n602 = local read "WS_On/Off"() -> (w746:bool)
      n603 = case shown="True" w746 {
        frame False {
        }
        frame True {
          n604 = local read "WS visa"() -> (w751:refnum<visa-resource-name>)
          n605 = call "T_RH_P.vi"("VISA in"=w751, "WS_Commands"=enum16{"OpenWS", "ReadTRHP", "CloseWS"}."CloseWS") -> ()  [unwired: 11 in, 3 out]
        }
      }
      n606 = Close File(refnum=w750) -> ()  [unwired: 1 in, 2 out]
      n607 = Close File(refnum=w749) -> ()  [unwired: 1 in, 2 out]
      n608 = Close File(refnum=w748) -> ()  [unwired: 1 in, 2 out]
      n609 = Close File(refnum=w747) -> ()  [unwired: 1 in, 2 out]
    }
  }
  "FileHour" <- -1 ("FileHour")
  "DataOpen" <- FALSE
